vi "新想法.vi"() -> ()   [LabVIEW 2020]
uses:
  <vilib>/Utility/miscctls.llb/LVBoundsTypeDef.ctl
  <vilib>/Utility/miscctls.llb/LVRectTypeDef.ctl
  <vilib>/Instr/_visa.llb/VISA Find Search Mode.ctl
  <vilib>/Utility/miscctls.llb/LVPointTypeDef.ctl
  <vilib>/Utility/config.llb/Write Key (String).vi
  <vilib>/Utility/config.llb/Read Key (String).vi
  <vilib>/Utility/file.llb/Write Delimited Spreadsheet (string).vi
  <vilib>/Modbus/master/Modbus Master.lvclass
  <vilib>/Utility/config.llb/NI_LVConfig.lvlib
  pem/LABVIEW.dll
  <vilib>/Modbus/master/Create Master Instance (Serial).vi
panel:
  in  "数据分析":bool
  in  "实时数据":bool
  in  "按钮":bool
  in  "文本下拉列表":u16(ring)=50 items=["30"=300, "35"=350, "40"=400, "45"=450, "50"=500, "55"=550, "60"=600, "65"=650, "70"=700, "75"=750, "80"=800]
  out "当前温度 2":dbl
  out "error out":errorcluster caption="错误输出"
  out "退出":bool
  out "保存所有":bool
  out "分析":bool
  out "配置":bool
  out "连接":bool
  out "数组 2":refnum<vi>[](array[refnum])
  in  "选项卡控件 3":enum32{"选项卡 2"}(tab)
  in  "搜索设备":bool
  in  "通讯方式选择":enum32{"USB", "ETHERNET", "RS485", "GPIB"}(radio)
  in  "表格":string[][](table)
  in  "通道选择":enum32{"ALL", "A1", "A2", "A3", "A4"}(radio) caption="设置通道"
  in  "测试项目":enum32{"EIS", "极化曲线", "耐久性曲线", "线性扫描"}(radio)
  in  "1":bool
  in  "测试项目 2":enum32{"极化曲线", "耐久性测试", "EIS"}(tab)
  in  "Ⅱ区测试点数:":i32
  in  "Ⅰ区测试点数:":dbl
  in  "膜面积(cm^2):":dbl
  in  "工步 2":i32(listbox)
  out "电流密度(A/cm^2):":dbl
  in  "测试时长(H):":dbl
  in  "施加电流(A):":dbl
  in  "有效膜面积(cm^2):":dbl
  in  "VISA resource name 2":refnum<visa-resource-name>="COM3" caption="VISA resource name"
  in  "保存":bool
  in  "电解槽最大电压":dbl caption="电解槽最高温度设定："
  in  "循环水最差水质":dbl caption="冷却水最高温度："
  in  "水箱最低液位":dbl caption="冷却水最高温度："
  in  "氢气出口最大压力：":dbl caption="电解槽进口压力设定："
  in  "电解槽最高温度：":dbl caption="电解槽最高温度设定："
  in  "氢气最大露点：":dbl caption="氢气露点设定："
  in  "冷却水最高温度：":dbl
  in  "水箱补水液位：":dbl caption="水箱补水液位设定："
  in  "气液分离液位：":dbl caption="气液分离液位设定："
  in  "氢气出口背压设定：":dbl
  in  "水质换水":dbl caption="水质换水设定："
  in  "流量":T1(ring)
  in  "泵头":enum16{"YZ1515", "YZ2515", "KZ25", "YZ35"}(ring)
  in  "单选按钮":enum32{"正转", "反转"}(radio)
  in  "单选按钮 2":enum32{"四线", "二线"}(radio)
  in  "采样率":dbl
  in  "采样数":dbl
  in  "VISA resource name":refnum<visa-resource-name>="COM3"
  in  "温度25":u16(ring)=50 caption="文本下拉列表" items=["30℃"=300, "35℃"=350, "40℃"=400, "45℃"=450, "50℃"=500, "55℃"=550, "60℃"=600, "65℃"=650, "70℃"=700, "75℃"=750, "80℃"=800]
  in  "2":bool
  in  "VISA resource name 3":refnum<visa-resource-name>="COM3" caption="VISA resource name"
  in  "电源类型":u16(ring) items=["ITECH", "TDK"]
  in  "3":bool
  in  "4":bool
  out "停止测试时间:":string
  out "开始测试时间:":string
  out "报警信息":string
  out "当前电压":string
  out "当前电流":string
  in  "报警状态":bool
  in  "运行状态":bool
  out "当前温度":string
  out "通讯方式":string
  out "测试类型 2":string
  out "电压范围":string
  out "电流范围":string
  out "电源模式":string
  out "登录时间：":string
  out "用户：":string
  out "字符串 3":string
  out "队列输出 2":refnum<queue>
  in  "开始测量":bool
  in  "开始测量 3":bool caption="开始测量"
  in  "开始测量 2":bool caption="开始测量"
  in  "开始测量 4":bool caption="开始测量"
  in  "通道选择 2":enum32{"未选择", "A1", "A2", "A3", "A4"}(radio)=enum."A1"
  in  "导出曲线":bool caption="历史曲线"
  in  "保存工步":bool
  in  "添加工步":bool
  in  "历史曲线":bool
  out "刷新":bool
  in  "重排所有视图":bool
  in  "显示所有视图":bool
  in  "水质 2":bool
  in  "工步":bool
  in  "压强":bool
  in  "温度":bool
  in  "电流/电压":bool
  out "水箱液位 2":string
  out "氢中氧 2":string
  out "氢渗 2":string
  out "循环水压 2":string
  out "水质电导率 2":string
  out "电解电流 2":string
  in  "水质x轴网格线":bool
  in  "水质y轴网格线":bool
  in  "文本下拉列表 7":u16(ring) items=["线性", "散点", "分步", "分步水平"]
  in  "文本下拉列表 10":u16(ring) items=["导出数据到excel", "导出数据至剪贴板", "导出图像"]
  in  "压力x轴网格线":bool
  in  "压力y轴网格线":bool
  in  "文本下拉列表 6":u16(ring) items=["线性", "散点", "分步", "分步水平"]
  in  "文本下拉列表 9":u16(ring) items=["导出数据到excel", "导出数据至剪贴板", "导出图像"]
  in  "温度x轴网格线":bool
  in  "温度y轴网格线":bool
  in  "文本下拉列表 5":u16(ring) items=["线性", "散点", "分步", "分步水平"]
  in  "文本下拉列表 8":u16(ring) items=["导出数据到excel", "导出数据至剪贴板", "导出图像"]
  in  "文本下拉列表 2":u16(ring) items=["导出数据到excel", "导出数据至剪贴板", "导出图像"]
  in  "极化y轴网格线":bool
  in  "极化x轴网格线":bool
  in  "文本下拉列表 3":u16(ring) items=["极化曲线1", "极化曲线2"]
  in  "文本下拉列表 4":u16(ring) items=["线性", "散点", "分步", "分步水平"]
  in  "选项卡控件 2":T2(tab)
  in  "树形控件 2":string(tree)
  in  "撤销当前设置":bool
  in  "保存当前设置":bool
  in  "打开历史设置":bool
  out "水箱温度 2":string
  out "冷却水水压 2":string
  out "电解电压 2":string
  out "气分液位 2":string
  out "微量氧 2":string
  out "露点仪 2":string
  out "冷凝器液位 2":string
  out "冷凝器液位":string
  out "露点仪":string
  out "微量氧":string
  out "纯度仪":string
  out "气分液位":string
  out "电解电压":string
  out "电解电流":string
  out "水质电导率":string
  out "循环水压":string
  out "冷却水水压":string
  out "氢渗":string
  out "氢中氧":string
  out "水箱温度":string
  out "水箱液位":string
  out "纯度仪 2":string
  out "new picture":picture caption="新图片"
  in  "选项卡控件 4":enum32{"极化曲线", "温度", "压力", "水质"}(tab)
  in  "极化坐标":string
  in  "字符串 11":string
  in  "字符串 10":string
  in  "字符串 9":string
  in  "字符串 8":string
  out "XY图":cluster{"添加的数组":dbl[], "添加的数组":dbl[]}[](graph)
  in  "温度坐标":string
  out "波形图":dbl[](graph)
  in  "压力坐标":string
  out "波形图 2":dbl[](graph)
  in  "水质坐标":string
  out "波形图 3":dbl[](graph)
  out "字符串 2":string
  in  "寻找设备":bool
  in  "串口号":u16(ring)
  out "数组 8":string[](array[string])
  in  "字符串":string
  out "数值 6":i32
  out "电流":dbl
  out "电压":dbl
  out "数据":string
  in  "数组 4":refnum<vi>[](array[refnum])
  in  "数组 5":refnum<vi>[](array[refnum])
  in  "数组 6":refnum<vi>[](array[refnum])
  in  "数组 7":refnum<vi>[](array[refnum])
  out "新值":bool
  in  "字符串 4":string
  in  "字符串 5":string
  in  "字符串 6":string
  in  "字符串 7":string
  out "查找列表":string[](array[string])
  in  "数值 5":i32
  in  "数组 12":string[][](array[string]) caption="数组"
  in  "数组 11":string[][](array[string]) caption="数组"
  in  "数组 10":string[][](array[string]) caption="数组"
  in  "数组":string[][](array[string])
  in  "压力3":string[][](array[string])
  in  "压力4":string[][](array[string])
  in  "压力2":string[][](array[string])
  in  "压力1":string[][](array[string])
  out "数值":i32
  in  "test":bool
  in  "水质4":string[][](array[string])
  in  "温度4":string[][](array[string])
  in  "水质3":string[][](array[string])
  in  "温度3":string[][](array[string])
  in  "水质2":string[][](array[string])
  in  "温度2":string[][](array[string])
  in  "温度显示 4":dbl
  in  "温度显示 3":dbl
  in  "温度显示 2":dbl
  in  "温度显示":dbl
  in  "所有数据4":string[][](array[string])
  in  "所有数据3":string[][](array[string])
  in  "所有数据2":string[][](array[string])
  in  "所有数据":string[][](array[string])
  out "数值 4":i32
  out "数值 3":i32
  out "数值 2":i32
  in  "极化曲线4":dbl[][](array[numeric])
  in  "极化电压4":dbl
  in  "极化电流4":dbl
  in  "电压4":dbl[](array[numeric])
  in  "电流4":dbl[](array[numeric])
  in  "极化曲线3":dbl[][](array[numeric])
  in  "极化电压3":dbl
  in  "极化电流3":dbl
  in  "电压3":dbl[](array[numeric])
  in  "电流3":dbl[](array[numeric])
  in  "极化曲线2":dbl[][](array[numeric])
  in  "极化电压2":dbl
  in  "极化电流2":dbl
  in  "电压2":dbl[](array[numeric])
  in  "电流2":dbl[](array[numeric])
  in  "极化曲线1":dbl[][](array[numeric])
  in  "极化电压1":dbl
  in  "极化电流1":dbl
  in  "电压1":dbl[](array[numeric])
  in  "电流1":dbl[](array[numeric])
  in  "水质1":string[][](array[string])
  in  "温度1":string[][](array[string])
  in  "数组 3":refnum<vi>[](array[refnum])
  out "输出电磁阀":bool
  out "露点电磁阀":bool
  out "流量电磁阀":bool
  out "补水电磁阀":bool
  out "排水电磁阀":bool
  out "冷水控温阀":bool
  out "排尽电磁阀":bool
  out "冷却水温度过高报警":bool
  out "电堆超压报警":bool
  out "露点报警":bool
  out "电堆温度报警":bool
  out "积水报警":bool
  out "水质报警":bool
  out "水箱缺水报警":bool
  out "循环水温度报警":bool
  out "循环水流量报警":bool
  out "氢气出口超压报警":bool
  # "设备列表"
  # "参数设置"
  # "测试设置"
  # "VISA"
  # "VISA"
  # "MPa"
  # "MΩ.cm"
  # "cm"
  # "cm"
  # "报警参数设置"
  # "℃"
  # "℃"
  # "V"
  # "℃"
  # "cm"
  # "MPa"
  # "MΩ.cm"
  # "工作设置"
  # "电源设置"
  # "VISA"
  # "通道设置"
  # "工步设置"
  # "测试通道"
  # "CH1"
  # "CH2"
  # "CH3"
  # "CH4"
  # "电磁阀状态"
  # "报警状态"
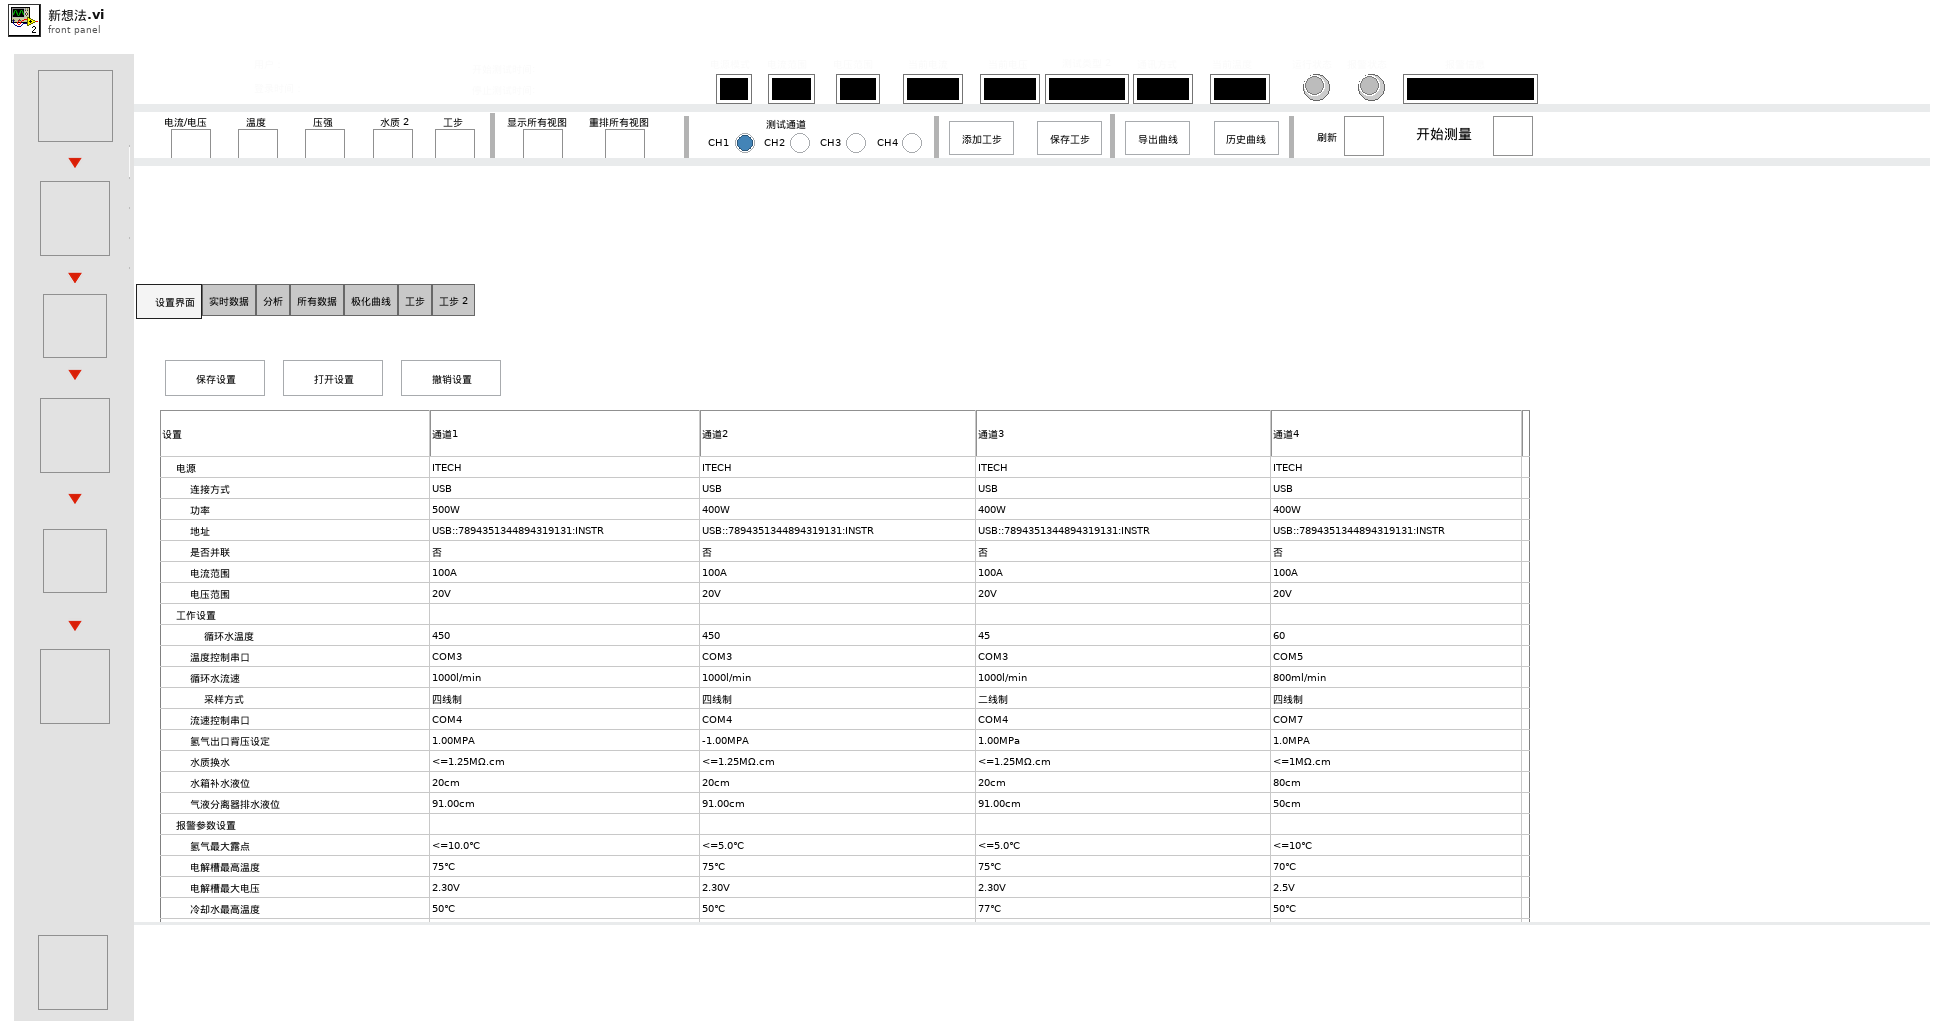
[diagram p1: front panel]
types:
  T1 = enum16{"200ml/min", "400lml/min", "600ml/min", "800ml/min", "1000ml/min", "1200ml/min", "1400ml/min", "1600ml/min"}
  T2 = enum32{"    设置界面", "实时数据", "分析", "所有数据", "极化曲线", "工步", "工步 2"}
  T3 = enum16{"Always On", "Always Off", "Off While Running"}
  T4 = enum8{"Enabled", "Disabled", "Disabled and Grayed Out"}
  T5 = typedef "LVBoundsTypeDef.ctl" = cluster{"Width":u32, "Height":u32}
  T6 = typedef "imagedata.ctl" = cluster{"image type":i32, "image depth":i32, "image":u8[], "mask":u8[], "colors":u32[], "Rectangle":cluster{"left":i16, "top":i16, "right":i16, "bottom":i16}}
  T7 = typedef "LVPointTypeDef.ctl" = cluster{"Horizontal":i16, "Vertical":i16}
  T8 = cluster{"温度1":refnum<vi>, "温度2":refnum<vi>, "温度3":refnum<vi>, "温度4":refnum<vi>}
  T9 = cluster{"水质1":refnum<vi>, "水质2":refnum<vi>, "水质3":refnum<vi>, "水质4":refnum<vi>}
  T10 = cluster{"极化曲线1":refnum<vi>, "极化曲线2":refnum<vi>, "极化曲线3":refnum<vi>, "极化曲线4":refnum<vi>}
  T11 = cluster{"电压1":refnum<vi>, "电压2":refnum<vi>, "电压3":refnum<vi>, "电压4":refnum<vi>}
  T12 = cluster{"电流1":refnum<vi>, "电流2":refnum<vi>, "电流3":refnum<vi>, "电流4":refnum<vi>}
  T13 = cluster{"压力1":refnum<vi>, "压力2":refnum<vi>, "压力3":refnum<vi>, "压力4":refnum<vi>}
  T14 = cluster{"所有数据":refnum<vi>, "所有数据2":refnum<vi>, "所有数据3":refnum<vi>, "所有数据4":refnum<vi>}
  T15 = enum32{"Invalid", "Standard", "Closed", "Hidden", "Minimized", "Maximized"}
  T16 = cluster{"所有数据":refnum<vi>, "数值":refnum<vi>, "极化曲线1":refnum<vi>, "极化电压1":refnum<vi>, "极化电流1":refnum<vi>, "电压1":refnum<vi>, "电流1":refnum<vi>, "水质1":refnum<vi>, "温度1":refnum<vi>, "温度显示":refnum<vi>, "压力1":refnum<vi>}
  T17 = cluster{"水质2":refnum<vi>, "温度2":refnum<vi>, "温度显示 2":refnum<vi>, "所有数据2":refnum<vi>, "数值 2":refnum<vi>, "极化曲线2":refnum<vi>, "极化电压2":refnum<vi>, "极化电流2":refnum<vi>, "电压2":refnum<vi>, "电流2":refnum<vi>, "压力2":refnum<vi>}
  T18 = cluster{"水质3":refnum<vi>, "温度3":refnum<vi>, "温度显示 3":refnum<vi>, "所有数据3":refnum<vi>, "数值 3":refnum<vi>, "极化曲线3":refnum<vi>, "极化电压3":refnum<vi>, "极化电流3":refnum<vi>, "电压3":refnum<vi>, "电流3":refnum<vi>, "压力3":refnum<vi>}
  T19 = cluster{"水质4":refnum<vi>, "温度4":refnum<vi>, "温度显示 4":refnum<vi>, "所有数据4":refnum<vi>, "数值 4":refnum<vi>, "极化曲线4":refnum<vi>, "极化电压4":refnum<vi>, "极化电流4":refnum<vi>, "电压4":refnum<vi>, "电流4":refnum<vi>, "压力4":refnum<vi>}
  T20 = typedef "LVRectTypeDef.ctl" = cluster{"Left":i16, "Top":i16, "Right":i16, "Bottom":i16}
  T21 = enum16{"open", "replace", "create", "open or create", "replace or create", "replace or create with confirmation"}
  T22 = typedef "LVPoint32TypeDef.ctl" = cluster{"Horizontal":i32, "Vertical":i32}
  T23 = enum32{"Bad", "Idle", "Run top level", "Running"}
  T24 = cluster{"添加的数组":dbl[], "添加的数组":dbl[], "添加的数组":dbl[], "添加的数组":dbl[], dbl}
  T25 = typedef "NI_LVConfig.lvlib/Config Data RefNum.ctl" = refnum<k1>
  T26 = cluster{string, string[], string, i32, bool, i32}
  T27 = typedef "VISA Find Search Mode.ctl" = u32
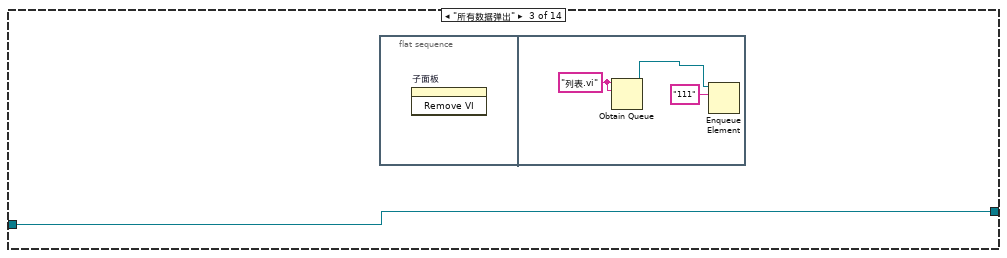
[diagram p4: hidden frame]
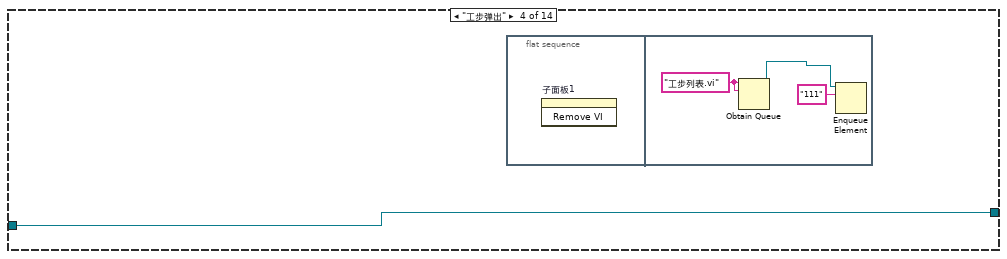
[diagram p5: hidden frame]
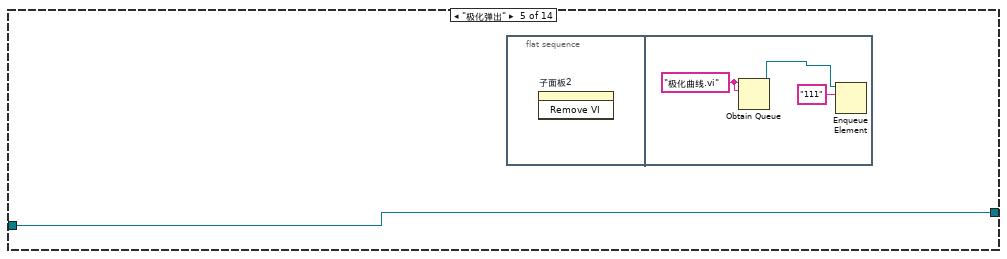
[diagram p6: hidden frame]
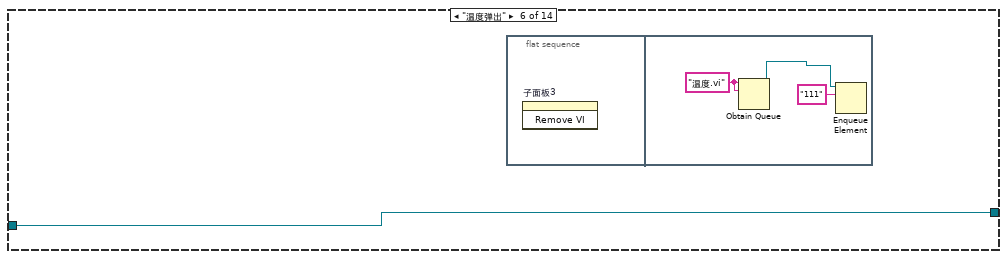
[diagram p7: hidden frame]
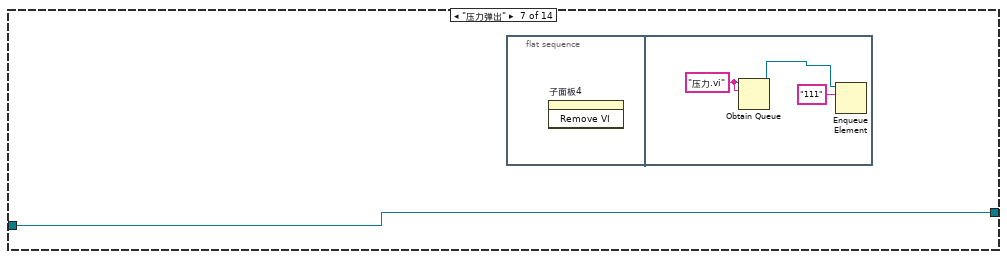
[diagram p8: hidden frame]
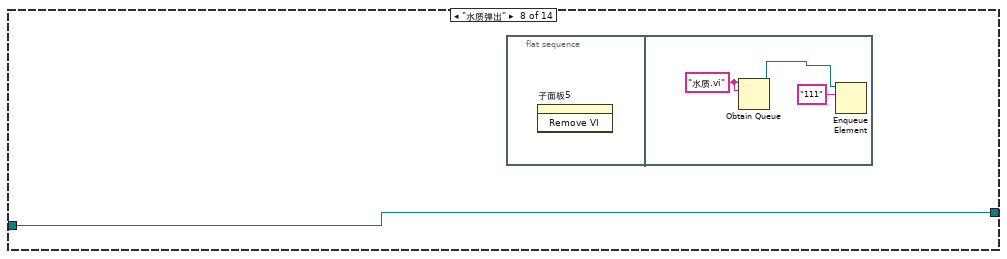
[diagram p9: hidden frame]
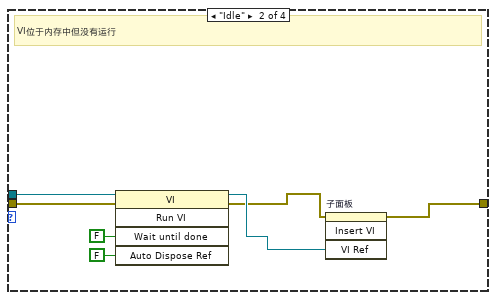
[diagram p12: hidden frame]
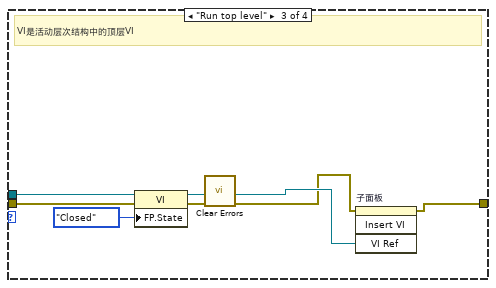
[diagram p13: hidden frame]
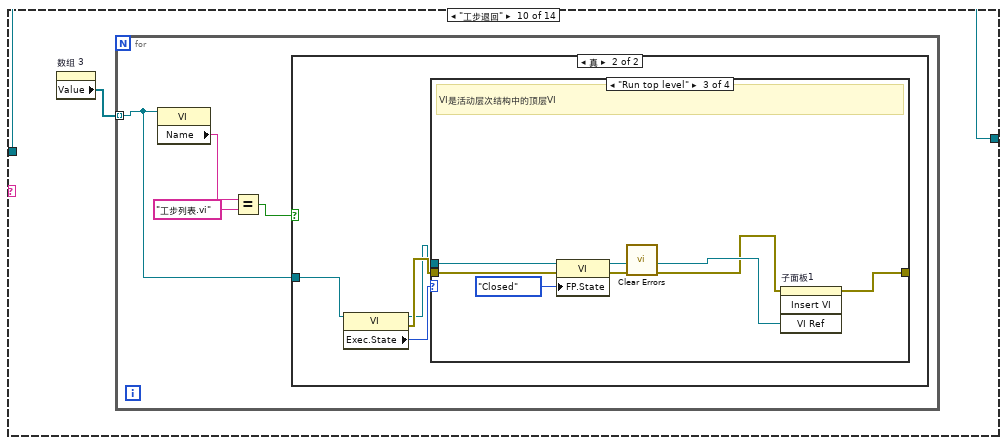
[diagram p14: hidden frame]
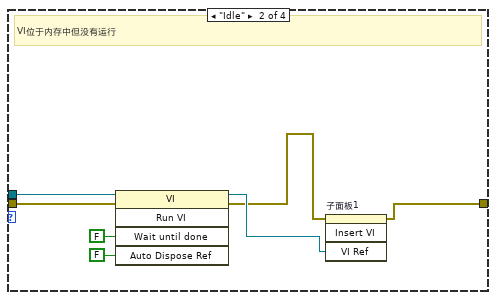
[diagram p17: hidden frame]
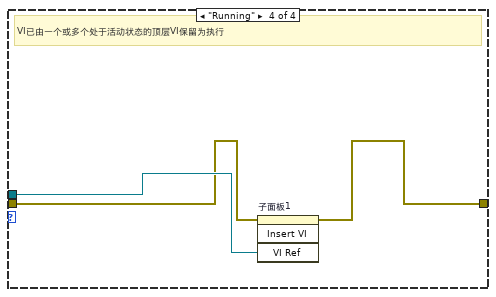
[diagram p18: hidden frame]
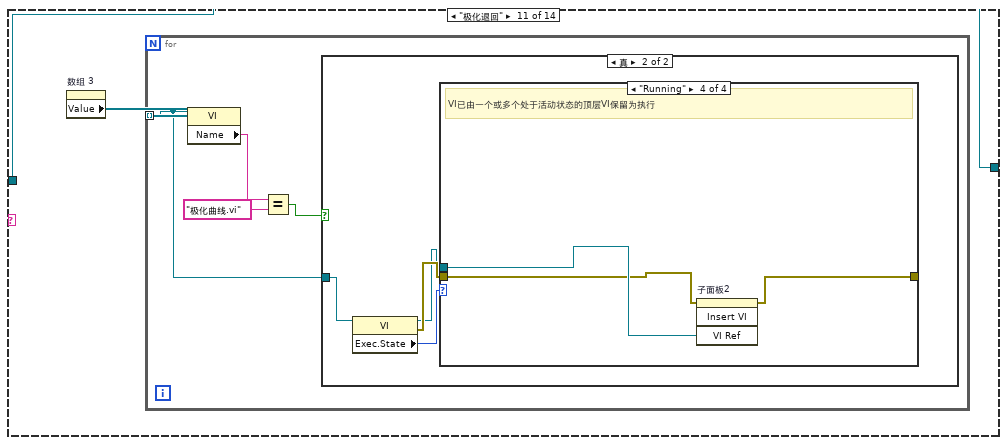
[diagram p19: hidden frame]
diagram:
  (unwired) string[] ["循环水温度", "温度控制串口", "循环水流速", "流速控制串口", "采样方式", "氢气出口背压设定", "水质换水", "水箱补水液位", "气液分离器排水液位", "氢气最大露点", "电解槽最高温度", "电解槽最大电压", "冷却水最高温度", "水箱最低液位", "氢气出口最大压力", "循环水最差水质"]
  (unwired) TRUE ("布尔 17")
  (unwired) "添加工步"
  # "A2"
  # "USB0::0x2EC7::0x3000::803489033757710010::INSTR"
  # "a1"
  # "USB0::0x2EC7::0x3000::803489033757710011::INSTR"
  n1 = flat-sequence {
    frame #0 {
      n2 = control-ref of="冷凝器液位 2"() -> (w98:refnum<vi>)
      n3 = control-ref of="露点仪 2"() -> (w99:refnum<vi>)
      n4 = control-ref of="微量氧 2"() -> (w100:refnum<vi>)
      n5 = control-ref of="纯度仪 2"() -> (w101:refnum<vi>)
      n6 = control-ref of="气分液位 2"() -> (w102:refnum<vi>)
      n7 = control-ref of="电解电压 2"() -> (w103:refnum<vi>)
      n8 = control-ref of="电解电流 2"() -> (w104:refnum<vi>)
      n9 = control-ref of="水质电导率 2"() -> (w105:refnum<vi>)
      n10 = control-ref of="循环水压 2"() -> (w106:refnum<vi>)
      n11 = control-ref of="冷却水水压 2"() -> (w107:refnum<vi>)
      n12 = control-ref of="氢渗 2"() -> (w108:refnum<vi>)
      n13 = control-ref of="氢中氧 2"() -> (w109:refnum<vi>)
      n14 = control-ref of="水箱温度 2"() -> (w110:refnum<vi>)
      n15 = control-ref of="水箱液位 2"() -> (w111:refnum<vi>)
      n16 = Build Array(w98, w99, w100, w101, w102, w103, w104, w105, w106, w107, w108, w109, w110, w111) -> (w112:refnum<vi>[])
      n17 = control-ref of="冷凝器液位"() -> (w83:refnum<vi>)
      n18 = control-ref of="露点仪"() -> (w84:refnum<vi>)
      n19 = control-ref of="微量氧"() -> (w85:refnum<vi>)
      n20 = control-ref of="纯度仪"() -> (w86:refnum<vi>)
      n21 = control-ref of="气分液位"() -> (w87:refnum<vi>)
      n22 = control-ref of="电解电压"() -> (w88:refnum<vi>)
      n23 = control-ref of="电解电流"() -> (w89:refnum<vi>)
      n24 = control-ref of="水质电导率"() -> (w90:refnum<vi>)
      n25 = control-ref of="循环水压"() -> (w91:refnum<vi>)
      n26 = control-ref of="冷却水水压"() -> (w92:refnum<vi>)
      n27 = control-ref of="氢渗"() -> (w93:refnum<vi>)
      n28 = control-ref of="氢中氧"() -> (w94:refnum<vi>)
      n29 = control-ref of="水箱温度"() -> (w95:refnum<vi>)
      n30 = control-ref of="水箱液位"() -> (w96:refnum<vi>)
      n31 = Build Array(w83, w84, w85, w86, w87, w88, w89, w90, w91, w92, w93, w94, w95, w96) -> (w97:refnum<vi>[])
      n32 = for {
        tunnel: w97 -> [w116] mode=indexing
        tunnel: w112 -> [w114] mode=indexing
        n33 = property class="Str"(reference=w114, "Visible"=FALSE ("可见")) -> ()  [unwired: 1 in, 2 out]
        n34 = property class="Str"(reference=w116, "Visible"=FALSE ("可见")) -> ()  [unwired: 1 in, 2 out]
      }
    }
    frame #1 {
      n35 = for {
        tunnel: i32[] [5] -> [w120] mode=indexing
        n36 = property on="窗格" class="Pane"() -> ("Decos[]"=w119:refnum<vi>[])  [unwired: 2 in, 2 out]
        n37 = Index Array(array=w119, index=w120) -> (element=w118:refnum<vi>)
        n38 = property class="Decor"(reference=w118, "Visible"=TRUE ("可见")) -> ()  [unwired: 1 in, 2 out]
      }
    }
    frame #2 {
      n39 = disable-structure shown="禁用" {
        frame Disabled {
          n40 = for {
            tunnel: i32[] [0, 1, 2, 3, 4] -> [w126] mode=indexing
            n41 = property on="窗格" class="Pane"() -> ("Decos[]"=w125:refnum<vi>[])  [unwired: 2 in, 2 out]
            n42 = Index Array(array=w125, index=w126) -> (element=w124:refnum<vi>)
            n43 = property class="Decor"(reference=w124, "Visible"=FALSE ("可见")) -> ()  [unwired: 1 in, 2 out]
          }
        }
        frame Enabled {
        }
      }
      n44 = property on="分隔栏 2" class="Splitter"("Position"=113 ("分隔栏位置")) -> ()  [unwired: 2 in, 2 out]
    }
    frame #3 {
      n45 = property on="分隔栏 3" class="Splitter"("Position"=116 ("分隔栏位置")) -> ()  [unwired: 2 in, 2 out]
    }
    frame #4 {
      n46 = stacked-sequence {
        frame #0 {
          n47 = property on="分隔栏 4" class="Splitter"() -> ("Position"=w129:i32)  [unwired: 2 in, 2 out]
          n48 = Add(x=w129, y=32 ("分隔栏位置")) -> (x+y=w131:i32)
          n49 = property on="分隔栏 5" class="Splitter"("Position"=w131) -> ()  [unwired: 2 in, 2 out]
        }
        frame #1 {
          n50 = property on="分隔栏 4" class="Splitter"() -> ("Position"=w134:i32)  [unwired: 2 in, 2 out]
          n51 = Add(x=w134, y=62 ("分隔栏位置")) -> (x+y=w133:i32)
          n52 = property on="分隔栏 6" class="Splitter"("Position"=w133) -> ()  [unwired: 2 in, 2 out]
        }
        frame #2 {
          n53 = property on="分隔栏 4" class="Splitter"() -> ("Position"=w137:i32)  [unwired: 2 in, 2 out]
          n54 = Add(x=w137, y=92 ("分隔栏位置")) -> (x+y=w136:i32)
          n55 = property on="分隔栏 7" class="Splitter"("Position"=w136) -> ()  [unwired: 2 in, 2 out]
        }
        frame #3 {
          n56 = property on="分隔栏 4" class="Splitter"() -> ("Position"=w140:i32)  [unwired: 2 in, 2 out]
          n57 = Add(x=w140, y=122 ("分隔栏位置")) -> (x+y=w138:i32)
          n58 = property on="分隔栏 8" class="Splitter"("Position"=w138) -> ()  [unwired: 2 in, 2 out]
        }
      }
    }
  }
  n59 = disable-structure shown="禁用" {
    frame Disabled {
      n60 = flat-sequence {
        frame #0 {
          w141 = "已完成" ("活动单元格:字符串")
          w142 = 8 ("活动单元格:活动列数")
          w145 = "A1" ("活动项:标识符")
          n61 = Add() -> (x=w144:dbl, x+y=w143:dbl)  [unwired: 1 in]
        }
        frame #1 {
          n62 = Index Array(array=w151, index (col)=0 ("禁用的索引 (列)")) -> (element=w149)  [unwired: 1 in]
          n63 = Search 1D Array(1D array=w149, element=" " ("元素")) -> (index of element=w147:i32)  [unwired: 1 in]
          n64 = Equal?(y=w147) -> (x = y?=w146:bool)  [unwired: 1 in]
          n65 = case shown="假" w146 {
            tunnel: [w157 _] -> w151
            frame False {
              w152 = u32 6618880
              w153 = "正在运行" ("活动单元格:字符串")
              w154 = 8 ("活动单元格:活动列数")
              w155 = "A1" ("活动项:标识符")
              w161 = 3 ("活动单元格:活动列数")
              w162 = "A1" ("活动项:标识符")
              w167 = 5 ("活动单元格:活动列数")
              w168 = "A1" ("活动项:标识符")
              w172 = 4 ("活动单元格:活动列数")
              w171 = "A1" ("活动项:标识符")
              w175 = 7 ("活动单元格:活动列数")
              w174 = "A1" ("活动项:标识符")
              n66 = Index Array(array=w157) -> (element=w164)  [unwired: 2 in]
              n67 = Increment() -> (x+1=w156:dbl)  [unwired: 1 in]
              n68 = Index Array(array=w164, index=3 ("索引")) -> (element=w165)
              n69 = Index Array(array=w164, index=2 ("索引")) -> (element=w169)
              n70 = Index Array(array=w164, index=5 ("索引")) -> (element=w173)
              n71 = Format Into String(w156) -> (resulting string=w159:string)  [unwired: 3 in, 1 out]
              n72 = Concatenate Strings("工步", w159) -> (w158:string)
            }
            frame True {
              w176 = "已完成" ("活动单元格:字符串")
              w177 = 8 ("活动单元格:活动列数")
              w178 = "A1" ("活动项:标识符")
            }
          }
        }
        frame #2 {
          n73 = case shown="真" {
            selector: _ -> [_ _]
            tunnel: [w180 w201] -> w179
            frame False {
              n74 = Index Array(array=w188) -> (element=w189, index=w190:i32)
              n75 = Unbundle(w189) -> (w183, w185)
              n76 = Build Array(w183) -> (w184:void[], w182)
              n77 = Build Array (concatenate)(w185) -> (w186:void[], w181:void[])
              n78 = Bundle(w184, w186) -> (w187:cluster{void[], void[]})  [unwired: 1 in]
              n79 = Replace Array Subset(new element=w187, index=w190) -> (array=w188:cluster{void[], void[]}[], w180:cluster{void[], void[]}[])
            }
            frame True {
              n80 = Array Size() -> (array=w196:dbl[], size(s)=w197:i32)
              n81 = Index Array(array=w196, index=w197) -> (element=w198)
              n82 = Unbundle(w198) -> (w195, w194)
              n83 = Build Array (concatenate)(w195) -> (w193:void[], w200:void[])
              n84 = Build Array (concatenate)(w194) -> (w192:void[], w199:void[])
              n85 = Bundle(w193, w192) -> (w191:cluster{void[], void[]})  [unwired: 1 in]
              n86 = Insert Into Array(array=w196, new element=w191) -> (w201:cluster{void[], void[]}[])  [unwired: 1 in]
            }
          }
        }
      }
    }
    frame Enabled {
    }
  }
  n87 = disable-structure shown="禁用" {
    frame Disabled {
      n88 = case shown="\"YZ35\"" {
        selector: _ -> [_ _ _ _]
        tunnel: ["YZ1515" "yz2515" "KZ25" "YZ35"] -> _
        frame "YZ1515", Default {
        }
        frame "YZ2515" {
        }
        frame "KZ25" {
        }
        frame "YZ35" {
        }
      }
    }
    frame Enabled {
    }
  }
  n89 = property on="电压" class="DigNum (严格)"() -> ("Value"=w45:dbl)  [unwired: 2 in, 2 out]
  n90 = property on="电流" class="DigNum (严格)"() -> ("Value"=w42:dbl)  [unwired: 2 in, 2 out]
  n91 = flat-sequence {
    tunnel: [w222] -> w2
    frame #0 {
      w243 = u16 1 items=["ITECK", "TDK"] ("电源类型")
      w259 = T4."Enabled" ("禁用")
      w247 = string[][] []
      n92 = property on="重排所有视图" class="Bool (严格)"("Value"=FALSE ("重排所有视图")) -> (error out=w209:errorcluster)  [unwired: 2 in, 1 out]
      n93 = property on="显示所有视图" class="Bool (严格)"(error in=w209, "Value"=FALSE ("显示所有视图")) -> (error out=w208:errorcluster)  [unwired: 1 in, 1 out]
      n94 = property on="压强" class="Bool (严格)"(error in=w208, "Value"=FALSE ("压强")) -> (error out=w216:errorcluster)  [unwired: 1 in, 1 out]
      n95 = property on="电流/电压" class="Bool (严格)"(error in=w216, "Value"=FALSE ("电流/电压")) -> (error out=w215:errorcluster)  [unwired: 1 in, 1 out]
      n96 = property on="温度" class="Bool (严格)"(error in=w215, "Value"=FALSE ("温度")) -> (error out=w214:errorcluster)  [unwired: 1 in, 1 out]
      n97 = property on="工步" class="Bool (严格)"(error in=w214, "Value"=FALSE ("工步")) -> (error out=w213:errorcluster)  [unwired: 1 in, 1 out]
      n98 = property on="水质 2" class="Bool (严格)"(error in=w213, "Value"=FALSE ("水质 2")) -> (error out=w212:errorcluster)  [unwired: 1 in, 1 out]
      n99 = property on="选项卡控件 4" class="TabCtl (严格)"(error in=w212, "Value"=enum32{"极化曲线", "温度", "压力", "水质"}."极化曲线" ("选项卡控件 4")) -> (error out=w231:errorcluster)  [unwired: 1 in, 1 out]
      n100 = property on="电源类型" class="Ring (严格)"(error in=w231, "Value"=w243) -> (error out=w242:errorcluster)  [unwired: 1 in, 1 out]
      n101 = property on="选项卡控件 2" class="TabCtl (严格)"(error in=w242, "Value"=T2."    设置界面" ("选项卡控件 2")) -> (error out=w207:errorcluster)  [unwired: 1 in, 1 out]
      n102 = property on="通道选择 2" class="RadioBtnsControl (严格)"(error in=w207, "Value"=enum32{"未选择", "A1", "A2", "A3", "A4"}."A1" ("通道选择 2")) -> (error out=w265:errorcluster)  [unwired: 1 in, 1 out]
      n103 = property on="通道选择" class="RadioBtnsControl (严格)"(error in=w265, "Value"=enum32{"ALL", "A1", "A2", "A3", "A4"}."ALL" ("通道选择")) -> (error out=w263:errorcluster)  [unwired: 1 in, 1 out]
      n104 = property on="测试项目" class="RadioBtnsControl (严格)"(error in=w263, "Value"=enum32{"EIS", "极化曲线", "耐久性曲线", "线性扫描"}."极化曲线" ("测试项目：")) -> (error out=w261:errorcluster)  [unwired: 1 in, 1 out]
      n105 = property on="测试项目 2" class="TabCtl (严格)"(error in=w261, "Value"=enum32{"极化曲线", "耐久性测试", "EIS"}."极化曲线" ("测试项目 2")) -> (error out=w260:errorcluster)  [unwired: 1 in, 1 out]
      n106 = property on="数组 3" class="Arr (严格)"(error in=w260, "Value"=refnum<vi>[] [] ("数组 3")) -> (error out=w289:errorcluster)  [unwired: 1 in, 1 out]
      n107 = property on="数组" class="Arr (严格)"(error in=w289, "Value"=w247) -> (error out=w248:errorcluster)  [unwired: 1 in, 1 out]
      n108 = property on="数组 10" class="Arr (严格)"(error in=w248, "Value"=w247) -> (error out=w245:errorcluster)  [unwired: 1 in, 1 out]
      n109 = property on="数组 11" class="Arr (严格)"(error in=w245, "Value"=w247) -> (error out=w246:errorcluster)  [unwired: 1 in, 1 out]
      n110 = property on="数组 12" class="Arr (严格)"(error in=w246, "Value"=w247) -> (error out=w244:errorcluster)  [unwired: 1 in, 1 out]
      n111 = property on="数组 2" class="Arr (严格)"(error in=w244, "Value"=refnum<vi>[] [] ("数组 2")) -> (error out=w272:errorcluster)  [unwired: 1 in, 1 out]
      n112 = property on="数组 4" class="Arr (严格)"(error in=w272, "Value"=refnum<vi>[] [] ("数组 4")) -> (error out=w258:errorcluster)  [unwired: 1 in, 1 out]
      n113 = property on="分析" class="Bool (严格)"(error in=w258, "DisabledEnum"=w259) -> (error out=w257:errorcluster)  [unwired: 1 in, 1 out]
      n114 = property on="保存所有" class="Bool (严格)"(error in=w257, "DisabledEnum"=w259) -> (error out=w256:errorcluster)  [unwired: 1 in, 1 out]
      n115 = property on="连接" class="Bool (严格)"(error in=w256, "DisabledEnum"=w259) -> (error out=w255:errorcluster)  [unwired: 1 in, 1 out]
      n116 = property on="配置" class="Bool (严格)"(error in=w255, "DisabledEnum"=w259) -> (error out=w254:errorcluster)  [unwired: 1 in, 1 out]
      n117 = property on="通道选择" class="RadioBtnsControl (严格)"(error in=w254, "DisabledEnum"=w259) -> (error out=w253:errorcluster)  [unwired: 1 in, 1 out]
      n118 = property on="2" class="Bool (严格)"(error in=w253, "DisabledEnum"=w259) -> (error out=w252:errorcluster)  [unwired: 1 in, 1 out]
      n119 = property on="3" class="Bool (严格)"(error in=w252, "DisabledEnum"=w259) -> (error out=w251:errorcluster)  [unwired: 1 in, 1 out]
      n120 = property on="4" class="Bool (严格)"(error in=w251, "DisabledEnum"=w259) -> (error out=w250:errorcluster)  [unwired: 1 in, 1 out]
      n121 = property on="数组 5" class="Arr (严格)"(error in=w250, "Value"=refnum<vi>[] [] ("数组 4")) -> (error out=w270:errorcluster)  [unwired: 1 in, 1 out]
      n122 = property on="数组 6" class="Arr (严格)"(error in=w270, "Value"=refnum<vi>[] [] ("数组 4")) -> (error out=w269:errorcluster)  [unwired: 1 in, 1 out]
      n123 = property on="数组 7" class="Arr (严格)"(error in=w269, "Value"=refnum<vi>[] [] ("数组 4")) -> (error out=w241:errorcluster)  [unwired: 1 in, 1 out]
      n124 = property on="开始测量" class="Bool (严格)"(error in=w241, "Visible"=TRUE ("可见")) -> (error out=w284:errorcluster)  [unwired: 1 in, 1 out]
      n125 = property on="开始测量 2" class="Bool (严格)"(error in=w284, "Visible"=FALSE ("可见")) -> (error out=w283:errorcluster)  [unwired: 1 in, 1 out]
      n126 = property on="开始测量 3" class="Bool (严格)"(error in=w283, "Visible"=FALSE ("可见")) -> (error out=w282:errorcluster)  [unwired: 1 in, 1 out]
      n127 = property on="开始测量 4" class="Bool (严格)"(error in=w282, "Visible"=FALSE ("可见")) -> (error out=w281:errorcluster)  [unwired: 1 in, 1 out]
      n128 = property on="开始测量" class="Bool (严格)"(error in=w281, "Value"=FALSE ("开始测量")) -> (error out=w279:errorcluster)  [unwired: 1 in, 1 out]
      n129 = property on="开始测量 2" class="Bool (严格)"(error in=w279, "Value"=FALSE ("开始测量 2")) -> (error out=w277:errorcluster)  [unwired: 1 in, 1 out]
      n130 = property on="开始测量 3" class="Bool (严格)"(error in=w277, "Value"=FALSE ("开始测量 3")) -> (error out=w275:errorcluster)  [unwired: 1 in, 1 out]
      n131 = property on="开始测量 4" class="Bool (严格)"(error in=w275, "Value"=FALSE ("开始测量 4")) -> (error out=w240:errorcluster)  [unwired: 1 in, 1 out]
      n132 = property on="表格" class="Tbl (严格)"(error in=w240, "Value"=string[][] [] ("表格")) -> (error out=w237:errorcluster)  [unwired: 1 in, 1 out]
      n133 = property on="字符串 4" class="Str"(error in=w237, "Value"="" ("字符串 4")) -> (error out=w235:errorcluster)  [unwired: 1 in, 1 out]
      n134 = property on="新值" class="Bool (严格)"(error in=w235, "Value"=FALSE ("新值")) -> (error out=w233:errorcluster)  [unwired: 1 in, 1 out]
      n135 = property on="导出曲线" class="Bool (严格)"(error in=w233, "Value"=FALSE ("导出曲线")) -> (error out=w230:errorcluster)  [unwired: 1 in, 1 out]
      n136 = property on="极化坐标" class="Str"(error in=w230, "Visible"=FALSE ("可见")) -> (error out=w225:errorcluster)  [unwired: 1 in, 1 out]
      n137 = property on="水质坐标" class="Str"(error in=w225, "Visible"=FALSE ("可见")) -> (error out=w224:errorcluster)  [unwired: 1 in, 1 out]
      n138 = property on="压力坐标" class="Str"(error in=w224, "Visible"=FALSE ("可见")) -> (error out=w223:errorcluster)  [unwired: 1 in, 1 out]
      n139 = property on="温度坐标" class="Str"(error in=w223, "Visible"=FALSE ("可见")) -> (error out=w222:errorcluster)  [unwired: 1 in, 1 out]
    }
  }
  n140 = Bundle By Name(cluster=cluster{"状态":bool, "错误码":i32, string} {"状态"=TRUE, "错误码"=0, ""} ("输入簇"), "状态"=TRUE, "错误码"=0) -> (w78:cluster{"状态":bool, "错误码":i32, string})
  n141 = Number To Fractional String(number=w42, precision (6)=i16 1 ("精度(6)")) -> (F-format string=→"当前电压":string)  [unwired: 2 in]
  n142 = Number To Fractional String(number=w45, precision (6)=i16 1 ("精度(6)")) -> (F-format string=→"当前电流":string)  [unwired: 2 in]
  n143 = control-ref of="窗格 9"() -> (w58:refnum<vi>)
  n144 = Obtain Queue(name (unnamed)="数据处理队列" ("名称（未命名）"), element data type=w78, create if not found? (T)=TRUE ("如未找到则创建？(T)")) -> (queue out=w76:refnum<queue>)  [unwired: 2 in, 2 out]
  "队列输出 2" <- w76
  n145 = property class="Pane"(reference=w58, "VertScrollbarVisibility"=T3."Always Off" ("垂直滚动条可见")) -> (error out=w56:errorcluster)  [unwired: 1 in, 1 out]
  n146 = control-ref of="水质1"() -> ()  [unwired: 1 out]
  n147 = control-ref of="水质2"() -> ()  [unwired: 1 out]
  n148 = control-ref of="水质3"() -> ()  [unwired: 1 out]
  n149 = control-ref of="水质4"() -> ()  [unwired: 1 out]
  n150 = property on="4" class="Bool (严格)"(error in=w56, "Value"=FALSE ("3 2")) -> (error out=w59:errorcluster)  [unwired: 1 in, 1 out]
  n151 = while {
    tunnel: w76 -> [w293]
    tunnel: [w292] -> w75
    stop <- FALSE stop-if-true
    n152 = event shown="[0] 超时" {
      selector: _ -> [_]
      dyn-events: _ -> [_]
      timeout: 100 -> [_]
      tunnel: w293 -> [w302]
      tunnel: [w299] -> w292
      event Timeout {
        n153 = event-data() -> ()  [unwired: 1 in, 3 out]
        n154 = Dequeue Element(queue=w302, timeout in ms (-1)=-1 ("超时毫秒(-1)")) -> (queue out=w299:refnum<queue>, element=w300:cluster{"状态":bool, "错误码":i32, string})  [unwired: 1 in, 2 out]
        n155 = Unbundle(w300) -> ("状态"=w296:bool, "错误码"=w297:i32, w298:string)
        n156 = case shown="真" w296 {
          tunnel: w298 -> [_ w308]
          tunnel: w297 -> [_ w306]
          frame False {
          }
          frame True {
            n157 = Format Into String(w306) -> (resulting string=w305:string)  [unwired: 3 in, 1 out]
            n158 = Concatenate Strings(w308, "错误：" ("字符串"), w305) -> (w304:string)
            n159 = One Button Dialog(message=w304, button name ("OK")="确定" ("按钮名称（“确定”）")) -> ()  [unwired: 1 out]
          }
        }
      }
    }
  }
  n160 = property on="1" class="Bool (严格)"(error in=w59, "Value"=FALSE ("1")) -> (error out=w71:errorcluster)  [unwired: 1 in, 1 out]
  n161 = property on="2" class="Bool (严格)"(error in=w71, "Value"=FALSE ("2")) -> (error out=w70:errorcluster)  [unwired: 1 in, 1 out]
  n162 = property on="3" class="Bool (严格)"(error in=w70, "Value"=FALSE ("3")) -> (error out=w67:errorcluster)  [unwired: 1 in, 1 out]
  n163 = control-ref of="窗格 6"() -> (w69:refnum<vi>)
  n164 = property class="Pane"(reference=w69, error in=w67, "VertScrollbarVisibility"=T3."Always Off" ("垂直滚动条可见")) -> (error out=w64:errorcluster)  [unwired: 1 out]
  n165 = Release Queue(queue=w75) -> ()  [unwired: 2 in, 3 out]
  n166 = control-ref of="窗格 7"() -> (w65:refnum<vi>)
  n167 = property class="Pane"(reference=w65, error in=w64, "VertScrollbarVisibility"=T3."Always Off" ("垂直滚动条可见")) -> (error out=w61:errorcluster)  [unwired: 1 out]
  n168 = control-ref of="窗格 8"() -> (w62:refnum<vi>)
  n169 = property class="Pane"(reference=w62, error in=w61, "VertScrollbarVisibility"=T3."Always Off" ("垂直滚动条可见")) -> (error out=w39:errorcluster)  [unwired: 1 out]
  n170 = flat-sequence {
    tunnel: [w347] -> w1
    tunnel: w2 -> [w309]
    frame #0 {
      w339 = 0 ("数值 2")
      w355 = string[][] [] ("温度1")
      w356 = dbl[] [] ("电压1")
      w345 = string[][] [] ("温度1")
      n171 = property on="数值 4" class="DigNum (严格)"(error in=w309, "Value"=0 ("数值 4")) -> (error out=w323:errorcluster)  [unwired: 1 in, 1 out]
      n172 = property on="电压4" class="Arr (严格)"(error in=w323, "Value"=dbl[] [] ("电压4")) -> (error out=w322:errorcluster)  [unwired: 1 in, 1 out]
      n173 = property on="电流4" class="Arr (严格)"(error in=w322, "Value"=dbl[] [] ("电流4")) -> (error out=w321:errorcluster)  [unwired: 1 in, 1 out]
      n174 = property on="极化曲线4" class="Arr (严格)"(error in=w321, "Value"=dbl[][] [] ("极化曲线4")) -> (error out=w320:errorcluster)  [unwired: 1 in, 1 out]
      n175 = property on="所有数据4" class="Arr (严格)"(error in=w320, "Value"=string[][] [] ("所有数据4")) -> (error out=w319:errorcluster)  [unwired: 1 in, 1 out]
      n176 = property on="水质4" class="Arr (严格)"(error in=w319, "Value"=string[][] [] ("水质4")) -> (error out=w318:errorcluster)  [unwired: 1 in, 1 out]
      n177 = property on="温度4" class="Arr (严格)"(error in=w318, "Value"=string[][] [] ("温度4")) -> (error out=w317:errorcluster)  [unwired: 1 in, 1 out]
      n178 = property on="数值 3" class="DigNum (严格)"(error in=w317, "Value"=0 ("数值 3")) -> (error out=w316:errorcluster)  [unwired: 1 in, 1 out]
      n179 = property on="所有数据3" class="Arr (严格)"(error in=w316, "Value"=string[][] [] ("所有数据3")) -> (error out=w315:errorcluster)  [unwired: 1 in, 1 out]
      n180 = property on="水质3" class="Arr (严格)"(error in=w315, "Value"=string[][] [] ("水质3")) -> (error out=w314:errorcluster)  [unwired: 1 in, 1 out]
      n181 = property on="温度3" class="Arr (严格)"(error in=w314, "Value"=string[][] [] ("温度3")) -> (error out=w313:errorcluster)  [unwired: 1 in, 1 out]
      n182 = property on="电压3" class="Arr (严格)"(error in=w313, "Value"=dbl[] [] ("电压3")) -> (error out=w312:errorcluster)  [unwired: 1 in, 1 out]
      n183 = property on="电流3" class="Arr (严格)"(error in=w312, "Value"=dbl[] [] ("电流3")) -> (error out=w311:errorcluster)  [unwired: 1 in, 1 out]
      n184 = property on="极化曲线3" class="Arr (严格)"(error in=w311, "Value"=dbl[][] [] ("极化曲线3")) -> (error out=w310:errorcluster)  [unwired: 1 in, 1 out]
      n185 = property on="数值 2" class="DigNum (严格)"(error in=w310, "Value"=w339) -> (error out=w338:errorcluster)  [unwired: 1 in, 1 out]
      n186 = property on="数值" class="DigNum (严格)"(error in=w338, "Value"=w339) -> (error out=w346:errorcluster)  [unwired: 1 in, 1 out]
      n187 = property on="温度1" class="Arr (严格)"(error in=w346, "Value"=string[][] [] ("温度1")) -> (error out=w344:errorcluster)  [unwired: 1 in, 1 out]
      n188 = property on="压力1" class="Arr (严格)"(error in=w344, "Value"=w345) -> (error out=w343:errorcluster)  [unwired: 1 in, 1 out]
      n189 = property on="压力2" class="Arr (严格)"(error in=w343, "Value"=w345) -> (error out=w342:errorcluster)  [unwired: 1 in, 1 out]
      n190 = property on="压力3" class="Arr (严格)"(error in=w342, "Value"=w345) -> (error out=w341:errorcluster)  [unwired: 1 in, 1 out]
      n191 = property on="压力4" class="Arr (严格)"(error in=w341, "Value"=w345) -> (error out=w340:errorcluster)  [unwired: 1 in, 1 out]
      n192 = property on="水质1" class="Arr (严格)"(error in=w340, "Value"=w345) -> (error out=w363:errorcluster)  [unwired: 1 in, 1 out]
      n193 = property on="所有数据" class="Arr (严格)"(error in=w363, "Value"=string[][] [] ("温度1")) -> (error out=w361:errorcluster)  [unwired: 1 in, 1 out]
      n194 = property on="极化曲线1" class="Arr (严格)"(error in=w361, "Value"=dbl[][] [] ("极化曲线1")) -> (error out=w360:errorcluster)  [unwired: 1 in, 1 out]
      n195 = property on="电流1" class="Arr (严格)"(error in=w360, "Value"=dbl[] [] ("电压1")) -> (error out=w359:errorcluster)  [unwired: 1 in, 1 out]
      n196 = property on="电压1" class="Arr (严格)"(error in=w359, "Value"=dbl[] [] ("电压1")) -> (error out=w353:errorcluster)  [unwired: 1 in, 1 out]
      n197 = property on="电压2" class="Arr (严格)"(error in=w353, "Value"=w356) -> (error out=w352:errorcluster)  [unwired: 1 in, 1 out]
      n198 = property on="电流2" class="Arr (严格)"(error in=w352, "Value"=w356) -> (error out=w351:errorcluster)  [unwired: 1 in, 1 out]
      n199 = property on="水质2" class="Arr (严格)"(error in=w351, "Value"=w355) -> (error out=w350:errorcluster)  [unwired: 1 in, 1 out]
      n200 = property on="温度2" class="Arr (严格)"(error in=w350, "Value"=w355) -> (error out=w349:errorcluster)  [unwired: 1 in, 1 out]
      n201 = property on="所有数据2" class="Arr (严格)"(error in=w349, "Value"=w355) -> (error out=w348:errorcluster)  [unwired: 1 in, 1 out]
      n202 = property on="极化曲线2" class="Arr (严格)"(error in=w348, "Value"=dbl[][] [] ("极化曲线1")) -> (error out=w347:errorcluster)  [unwired: 1 in, 1 out]
    }
  }
  n203 = flat-sequence {
    frame #0 {
      n204 = call <vilib>:"Application Directory.vi"() -> ("Application Directory"=w368:path)
      n205 = Build Path(base path=w368, name or relative path="1.jpg") -> (appended path=w366:path)
      n206 = call <vilib>:"Read JPEG File.vi"("path to JPEG file"=w366) -> ("image data"=w369:T6)  [unwired: 8 in, 2 out]
      n207 = call <vilib>:"Draw Flattened Pixmap.vi"("image data"=w369) -> ("new picture"=→"new picture":picture)  [unwired: 8 in]
    }
    frame #1 {
    }
    frame #2 {
      n208 = property on="new picture" class="Pict"("Draw Area Size"=T5 {"Width"=1776, "Height"=860} ("绘图区域大小")) -> ()  [unwired: 2 in, 2 out]
    }
  }
  n209 = property on="当前温度 2" class="DigNum (严格)" props=["Value"]() -> ()  [unwired: 2 in, 3 out]
  n210 = property on="温度1" class="Arr (严格)" props=["Value"]() -> ()  [unwired: 2 in, 3 out]
  n211 = property on="队列输出 2" class="TypRef (严格)" props=["Value"]() -> ()  [unwired: 2 in, 3 out]
  n212 = while {
    shift-right: [w373] -> _
    shift-left: FALSE -> [w372]
    tunnel: w39 -> [_]
    stop <- FALSE stop-if-true
    n213 = event shown="[1] \"1\", \"2\", \"3\", \"4\": 值改变" {
      selector: _ -> [_ _]
      dyn-events: _ -> [_ _]
      timeout: 100 -> [_ _]
      tunnel: [w376 w381] -> w373
      tunnel: w372 -> [_ w382]
      event Timeout {
        n214 = event-data() -> ()  [unwired: 1 in, 3 out]
        n215 = property on="1" class="Bool (严格)"() -> ("Value"=w380:bool)  [unwired: 2 in, 2 out]
        n216 = property on="2" class="Bool (严格)"() -> ("Value"=w379:bool)  [unwired: 2 in, 2 out]
        n217 = property on="3" class="Bool (严格)"() -> ("Value"=w378:bool)  [unwired: 2 in, 2 out]
        n218 = property on="4" class="Bool (严格)"() -> ("Value"=w377:bool)  [unwired: 2 in, 2 out]
        n219 = Compound Arithmetic op=OR ("复合运算")(w380, w379, w378, w377) -> (w376:bool)
      }
      event "1", "2", "3", "4": Value Change {
        n220 = event-data() -> ("CtlRef"=w384:refnum<vi>, "NewVal"=w383:bool)  [unwired: 1 in, 4 out]
        n221 = case shown="真" w383 {
          tunnel: w384 -> [w386 w426]
          tunnel: w382 -> [_ w425]
          tunnel: [_ w425] -> w381
          frame False {
            n222 = property class="Bool (严格)"(reference=w386) -> ("Label.Text"=w385:string)  [unwired: 1 in, 2 out]
            n223 = Scan From String(format string="%d" ("格式字符串"), input string=w385) -> (output 1=w387:i32)  [unwired: 3 in, 3 out]
            n224 = control-ref of="窗格 6"() -> (w391:refnum<vi>)
            n225 = control-ref of="窗格 7"() -> (w390:refnum<vi>)
            n226 = control-ref of="窗格 8"() -> (w389:refnum<vi>)
            n227 = control-ref of="窗格 9"() -> (w398:refnum<vi>)
            n228 = Build Array(w391, w390, w389, w398) -> (w388:refnum<vi>[])
            n229 = Decrement(x=w387) -> (x-1=w392:i32)
            n230 = Delete From Array(array=w388, length=1 ("长度"), index=w392) -> (deleted portion=w395:refnum<vi>[])  [unwired: 1 out]
            n231 = Index Array(array=w395, index=0 ("索引")) -> (element=w397:refnum<vi>)
            n232 = case shown="\"4\"" w385 {
              tunnel: w397 -> [_ w400 w405 w412 w421]
              frame "假", Default {
              }
              frame "1" {
                n233 = property class="Pane"(reference=w400, "Origin"=T7 {"Horizontal"=0, "Vertical"=0} ("原点")) -> ()  [unwired: 1 in, 2 out]
                n234 = property class="Pane"(reference=w400, "VertScrollbarVisibility"=T3."Always Off" ("垂直滚动条可见")) -> ()  [unwired: 1 in, 2 out]
                n235 = property on="分隔栏 5" class="Splitter"() -> ("Position"=w403:i32)  [unwired: 2 in, 2 out]
                n236 = Subtract(x=w403, y=751) -> (x-y=w404:i32)
                n237 = property on="分隔栏 5" class="Splitter"("Position"=w404) -> ()  [unwired: 2 in, 2 out]
              }
              frame "2" {
                n238 = property on="分隔栏 6" class="Splitter"() -> ("Position"=w409:i32)  [unwired: 2 in, 2 out]
                n239 = property class="Pane"(reference=w405, "Origin"=T7 {"Horizontal"=0, "Vertical"=0} ("原点")) -> ()  [unwired: 1 in, 2 out]
                n240 = property class="Pane"(reference=w405, "VertScrollbarVisibility"=T3."Always Off" ("垂直滚动条可见")) -> ()  [unwired: 1 in, 2 out]
                n241 = Subtract(x=w409, y=751) -> (x-y=w410:i32)
                n242 = property on="分隔栏 6" class="Splitter"("Position"=w410) -> ()  [unwired: 2 in, 2 out]
              }
              frame "3" {
                n243 = property class="Pane"(reference=w412, "VertScrollbarVisibility"=T3."Always Off" ("垂直滚动条可见")) -> (reference out=w411:refnum<vi>)  [unwired: 1 in, 1 out]
                n244 = property on="分隔栏 7" class="Splitter"() -> ("Position"=w416:i32)  [unwired: 2 in, 2 out]
                n245 = Subtract(x=w416, y=751) -> (x-y=w415:i32)
                n246 = property on="分隔栏 7" class="Splitter"("Position"=w415) -> ()  [unwired: 2 in, 2 out]
                n247 = property class="Pane"(reference=w411, "Origin"=T7 {"Horizontal"=0, "Vertical"=0} ("原点")) -> ()  [unwired: 1 in, 2 out]
              }
              frame "4" {
                n248 = property class="Pane"(reference=w421, "VertScrollbarVisibility"=T3."Always Off" ("垂直滚动条可见")) -> (reference out=w420:refnum<vi>)  [unwired: 1 in, 1 out]
                n249 = property on="分隔栏 8" class="Splitter"() -> ("Position"=w419:i32)  [unwired: 2 in, 2 out]
                n250 = Subtract(x=w419, y=751) -> (x-y=w418:i32)
                n251 = property on="分隔栏 8" class="Splitter"("Position"=w418) -> ()  [unwired: 2 in, 2 out]
                n252 = property class="Pane"(reference=w420, "Origin"=T7 {"Horizontal"=0, "Vertical"=0} ("原点")) -> ()  [unwired: 1 in, 2 out]
              }
            }
          }
          frame True {
            n253 = case shown="真" w425 {
              tunnel: w426 -> [w437 w458]
              frame False {
                n254 = property class="Bool (严格)"(reference=w437) -> ("Label.Text"=w432:string)  [unwired: 1 in, 2 out]
                n255 = Scan From String(format string="%d" ("格式字符串"), input string=w432) -> (output 1=w430:i32)  [unwired: 3 in, 3 out]
                n256 = control-ref of="窗格 6"() -> (w435:refnum<vi>)
                n257 = control-ref of="窗格 7"() -> (w434:refnum<vi>)
                n258 = control-ref of="窗格 8"() -> (w433:refnum<vi>)
                n259 = control-ref of="窗格 9"() -> (w436:refnum<vi>)
                n260 = Decrement(x=w430) -> (x-1=w429:i32)
                n261 = Build Array(w435, w434, w433, w436) -> (w428:refnum<vi>[])
                n262 = Delete From Array(array=w428, index=w429) -> (deleted portion=w427:refnum<vi>)  [unwired: 1 in, 1 out]
                n263 = case shown="\"2\"" w432 {
                  tunnel: w427 -> [_ w439 w443 w448 w455]
                  frame "假", Default {
                  }
                  frame "1" {
                    n264 = property class="Pane"(reference=w439, "VertScrollbarVisibility"=T3."Always On" ("垂直滚动条可见")) -> ()  [unwired: 1 in, 2 out]
                    n265 = property on="分隔栏 5" class="Splitter"() -> ("Position"=w441:i32)  [unwired: 2 in, 2 out]
                    n266 = Add(x=w441, y=751) -> (x+y=w442:i32)
                    n267 = property on="分隔栏 5" class="Splitter"("Position"=w442) -> ()  [unwired: 2 in, 2 out]
                  }
                  frame "2" {
                    n268 = property class="Pane"(reference=w443, "VertScrollbarVisibility"=T3."Always On" ("垂直滚动条可见")) -> ()  [unwired: 1 in, 2 out]
                    n269 = property on="分隔栏 6" class="Splitter"() -> ("Position"=w446:i32)  [unwired: 2 in, 2 out]
                    n270 = Add(x=w446, y=751) -> (x+y=w447:i32)
                    n271 = property on="分隔栏 6" class="Splitter"("Position"=w447) -> ()  [unwired: 2 in, 2 out]
                  }
                  frame "3" {
                    n272 = property class="Pane"(reference=w448, "VertScrollbarVisibility"=T3."Always On" ("垂直滚动条可见")) -> ()  [unwired: 1 in, 2 out]
                    n273 = property on="分隔栏 7" class="Splitter"() -> ("Position"=w451:i32)  [unwired: 2 in, 2 out]
                    n274 = Add(x=w451, y=751) -> (x+y=w450:i32)
                    n275 = property on="分隔栏 7" class="Splitter"("Position"=w450) -> ()  [unwired: 2 in, 2 out]
                  }
                  frame "4" {
                    n276 = property class="Pane"(reference=w455, "VertScrollbarVisibility"=T3."Always On" ("垂直滚动条可见")) -> ()  [unwired: 1 in, 2 out]
                    n277 = property on="分隔栏 8" class="Splitter"() -> ("Position"=w454:i32)  [unwired: 2 in, 2 out]
                    n278 = Add(x=w454, y=751) -> (x+y=w453:i32)
                    n279 = property on="分隔栏 8" class="Splitter"("Position"=w453) -> ()  [unwired: 2 in, 2 out]
                  }
                }
              }
              frame True {
                n280 = stacked-sequence {
                  tunnel: w458 -> [w466 _]
                  tunnel: w458 -> [_ w516]
                  frame #0 {
                    n281 = control-ref of="1"() -> (w467:refnum<vi>)
                    n282 = control-ref of="2"() -> (w468:refnum<vi>)
                    n283 = control-ref of="3"() -> (w469:refnum<vi>)
                    n284 = control-ref of="4"() -> (w470:refnum<vi>)
                    n285 = property class="Bool (严格)"(reference=w466) -> ("Label.Text"=w465:string)  [unwired: 1 in, 2 out]
                    n286 = Scan From String(format string="%d" ("格式字符串"), input string=w465) -> (output 1=w463:i32)  [unwired: 3 in, 3 out]
                    n287 = Build Array(w467, w468, w469, w470) -> (w460:refnum<vi>[])
                    n288 = Decrement(x=w463) -> (x-1=w462:i32)
                    n289 = Delete From Array(array=w460, length=1 ("长度"), index=w462) -> (array with subset deleted=w459:refnum<vi>[])  [unwired: 1 out]
                    n290 = for {
                      tunnel: w459 -> [w472] mode=indexing
                      n291 = property class="Bool (严格)"(reference=w472) -> ("Value"=w471:bool)  [unwired: 1 in, 2 out]
                      n292 = Equal?(x=w471, y=TRUE) -> (x = y?=w473:bool)
                      n293 = case shown="真" w473 {
                        tunnel: w472 -> [_ w476]
                        frame False {
                        }
                        frame True {
                          n294 = property class="Bool (严格)"(reference=w476) -> ("Label.Text"=w480:string)  [unwired: 1 in, 2 out]
                          n295 = property class="Bool (严格)"(reference=w476, "Value"=FALSE ("值")) -> ()  [unwired: 1 in, 2 out]
                          n296 = Scan From String(format string="%d" ("格式字符串"), input string=w480) -> (output 1=w475:i32)  [unwired: 3 in, 3 out]
                          n297 = control-ref of="窗格 6"() -> (w484:refnum<vi>)
                          n298 = control-ref of="窗格 7"() -> (w483:refnum<vi>)
                          n299 = control-ref of="窗格 8"() -> (w482:refnum<vi>)
                          n300 = control-ref of="窗格 9"() -> (w488:refnum<vi>)
                          n301 = Decrement(x=w475) -> (x-1=w485:i32)
                          n302 = Build Array(w484, w483, w482, w488) -> (w481:refnum<vi>[])
                          n303 = Delete From Array(array=w481, length=1 ("长度"), index=w485) -> (deleted portion=w486:refnum<vi>[])  [unwired: 1 out]
                          n304 = Index Array(array=w486, index=0 ("索引")) -> (element=w487:refnum<vi>)
                          n305 = case shown="\"1\"" w480 {
                            tunnel: w487 -> [_ w491 w496 w503 w512]
                            frame "假", Default {
                            }
                            frame "1" {
                              n306 = property class="Pane"(reference=w491, "Origin"=T7 {"Horizontal"=0, "Vertical"=0} ("原点")) -> ()  [unwired: 1 in, 2 out]
                              n307 = property class="Pane"(reference=w491, "VertScrollbarVisibility"=T3."Always Off" ("垂直滚动条可见")) -> ()  [unwired: 1 in, 2 out]
                              n308 = property on="分隔栏 5" class="Splitter"() -> ("Position"=w494:i32)  [unwired: 2 in, 2 out]
                              n309 = Subtract(x=w494, y=751) -> (x-y=w495:i32)
                              n310 = property on="分隔栏 5" class="Splitter"("Position"=w495) -> ()  [unwired: 2 in, 2 out]
                            }
                            frame "2" {
                              n311 = property class="Pane"(reference=w496, "Origin"=T7 {"Horizontal"=0, "Vertical"=0} ("原点")) -> ()  [unwired: 1 in, 2 out]
                              n312 = property class="Pane"(reference=w496, "VertScrollbarVisibility"=T3."Always Off" ("垂直滚动条可见")) -> ()  [unwired: 1 in, 2 out]
                              n313 = property on="分隔栏 6" class="Splitter"() -> ("Position"=w500:i32)  [unwired: 2 in, 2 out]
                              n314 = Subtract(x=w500, y=751) -> (x-y=w501:i32)
                              n315 = property on="分隔栏 6" class="Splitter"("Position"=w501) -> ()  [unwired: 2 in, 2 out]
                            }
                            frame "3" {
                              n316 = property class="Pane"(reference=w503, "VertScrollbarVisibility"=T3."Always Off" ("垂直滚动条可见")) -> (reference out=w502:refnum<vi>)  [unwired: 1 in, 1 out]
                              n317 = property on="分隔栏 7" class="Splitter"() -> ("Position"=w507:i32)  [unwired: 2 in, 2 out]
                              n318 = Subtract(x=w507, y=751) -> (x-y=w506:i32)
                              n319 = property on="分隔栏 7" class="Splitter"("Position"=w506) -> ()  [unwired: 2 in, 2 out]
                              n320 = property class="Pane"(reference=w502, "Origin"=T7 {"Horizontal"=0, "Vertical"=0} ("原点")) -> ()  [unwired: 1 in, 2 out]
                            }
                            frame "4" {
                              n321 = property class="Pane"(reference=w512, "VertScrollbarVisibility"=T3."Always Off" ("垂直滚动条可见")) -> (reference out=w511:refnum<vi>)  [unwired: 1 in, 1 out]
                              n322 = property on="分隔栏 8" class="Splitter"() -> ("Position"=w510:i32)  [unwired: 2 in, 2 out]
                              n323 = Subtract(x=w510, y=751) -> (x-y=w509:i32)
                              n324 = property on="分隔栏 8" class="Splitter"("Position"=w509) -> ()  [unwired: 2 in, 2 out]
                              n325 = property class="Pane"(reference=w511, "Origin"=T7 {"Horizontal"=0, "Vertical"=0} ("原点")) -> ()  [unwired: 1 in, 2 out]
                            }
                          }
                        }
                      }
                    }
                  }
                  frame #1 {
                    n326 = property class="Bool (严格)"(reference=w516) -> ("Label.Text"=w522:string)  [unwired: 1 in, 2 out]
                    n327 = Scan From String(format string="%d" ("格式字符串"), input string=w522) -> (output 1=w521:i32)  [unwired: 3 in, 3 out]
                    n328 = control-ref of="窗格 6"() -> (w525:refnum<vi>)
                    n329 = control-ref of="窗格 7"() -> (w524:refnum<vi>)
                    n330 = control-ref of="窗格 8"() -> (w523:refnum<vi>)
                    n331 = control-ref of="窗格 9"() -> (w526:refnum<vi>)
                    n332 = Decrement(x=w521) -> (x-1=w520:i32)
                    n333 = Build Array(w525, w524, w523, w526) -> (w519:refnum<vi>[])
                    n334 = Delete From Array(array=w519, index=w520) -> (deleted portion=w518:refnum<vi>)  [unwired: 1 in, 1 out]
                    n335 = case shown="\"4\"" w522 {
                      tunnel: w518 -> [_ w528 w532 w537 w544]
                      frame "假", Default {
                      }
                      frame "1" {
                        n336 = property on="分隔栏 5" class="Splitter"() -> ("Position"=w530:i32)  [unwired: 2 in, 2 out]
                        n337 = property class="Pane"(reference=w528, "VertScrollbarVisibility"=T3."Always On" ("垂直滚动条可见")) -> ()  [unwired: 1 in, 2 out]
                        n338 = Add(x=w530, y=751) -> (x+y=w531:i32)
                        n339 = property on="分隔栏 5" class="Splitter"("Position"=w531) -> ()  [unwired: 2 in, 2 out]
                      }
                      frame "2" {
                        n340 = property on="分隔栏 6" class="Splitter"() -> ("Position"=w535:i32)  [unwired: 2 in, 2 out]
                        n341 = property class="Pane"(reference=w532, "VertScrollbarVisibility"=T3."Always On" ("垂直滚动条可见")) -> ()  [unwired: 1 in, 2 out]
                        n342 = Add(x=w535, y=751) -> (x+y=w536:i32)
                        n343 = property on="分隔栏 6" class="Splitter"("Position"=w536) -> ()  [unwired: 2 in, 2 out]
                      }
                      frame "3" {
                        n344 = property on="分隔栏 7" class="Splitter"() -> ("Position"=w540:i32)  [unwired: 2 in, 2 out]
                        n345 = property class="Pane"(reference=w537, "VertScrollbarVisibility"=T3."Always On" ("垂直滚动条可见")) -> ()  [unwired: 1 in, 2 out]
                        n346 = Add(x=w540, y=751) -> (x+y=w539:i32)
                        n347 = property on="分隔栏 7" class="Splitter"("Position"=w539) -> ()  [unwired: 2 in, 2 out]
                      }
                      frame "4" {
                        n348 = property on="分隔栏 8" class="Splitter"() -> ("Position"=w543:i32)  [unwired: 2 in, 2 out]
                        n349 = property class="Pane"(reference=w544, "VertScrollbarVisibility"=T3."Always On" ("垂直滚动条可见")) -> ()  [unwired: 1 in, 2 out]
                        n350 = Add(x=w543, y=751) -> (x+y=w542:i32)
                        n351 = property on="分隔栏 8" class="Splitter"("Position"=w542) -> ()  [unwired: 2 in, 2 out]
                      }
                    }
                  }
                }
              }
            }
          }
        }
      }
    }
  }
  n352 = property on="窗格" class="Pane"() -> ("Decos[]"=w36:refnum<vi>[])  [unwired: 2 in, 2 out]
  n353 = for {
    tunnel: w36 -> [w548] mode=indexing
    n354 = property class="Decor"(reference=w548, "Visible"=TRUE ("可见")) -> ()  [unwired: 1 in, 2 out]
  }
  n355 = disable-structure shown="禁用" {
    disable-tunnel: [w550 _] -> w38
    frame Disabled {
      w558 = u16 0 items=["无", "奇", "偶"] ("parity (Even)")
      n356 = To Variant() -> (anything=w549:cluster{}, Variant=w555:variant)
      n357 = Variant To Data(type="", Variant=w555) -> (data=→"数据":string)  [unwired: 1 in, 1 out]
      n358 = call-poly <vilib>:"Create Master Instance.vi"("serial type"=enum16{"RTU", "ASCII"}."RTU", "parity (Even)"=w558, "unit ID"=u8 1, "baud rate (9600)"=u32 9600, "VISA resource name"=w549) -> ("error out"=w552:errorcluster, "serial master instance"=w550:refnum<class "Modbus Master.lvclass">)  [unwired: 5 in]
      n359 = property on="字符串" class="Str"("Value"="1" ("字符串")) -> ()  [unwired: 2 in, 2 out]
      n360 = while {
        tunnel: w550 -> [w563]
        tunnel: w552 -> [w561]
        stop <- FALSE stop-if-true
        n361 = Wait (ms)(milliseconds to wait=u32 100 ("等待时间（毫秒）")) -> ()  [unwired: 1 out]
        n362 = case shown="\"1\", 默认" "字符串" {
          tunnel: w563 -> [w576 w592 _]
          tunnel: w561 -> [w575 w591 _]
          tunnel: [w572 w582 _] -> _
          tunnel: [w571 w581 _] -> _
          frame "1", Default {
            n363 = call-dynamic "Read Holding Registers.vi"("error in (no error)"=w575, "number of holding registers"=u16 1, "starting address"=u16 258, "Modbus master in"=w576) -> ("error out"=w571:errorcluster, "register values"=w570:u16[], "Modbus master out"=w572:refnum<class "Modbus Master.lvclass">)  [unwired: 5 in]
            "error out" <- w571
            n364 = Index Array(array=w570, index=0 ("索引")) -> (element=w568:u16)
            n365 = To Double Precision Float(number=w568) -> (double precision float=w567:dbl)
            n366 = Divide(x=w567, y=10.0) -> (x/y=→"当前温度 2":dbl)
          }
          frame "2" {
            n367 = call-dynamic "Read Holding Registers.vi"("error in (no error)"=w591, "number of holding registers"=u16 1, "starting address"=u16 258, "Modbus master in"=w592) -> ("error out"=w581:errorcluster, "register values"=w588:u16[], "Modbus master out"=w582:refnum<class "Modbus Master.lvclass">)  [unwired: 5 in]
            n368 = Index Array(array=w588, index=0 ("索引")) -> (element=w586:u16)
            n369 = To Double Precision Float(number=w586) -> (double precision float=w585:dbl)
            n370 = Divide(x=w585, y=10.0) -> (x/y=w577:dbl)
            n371 = Divide(x="文本下拉列表", y=u16 100) -> (x/y=w579:dbl)
            n372 = Greater Or Equal?(x=w577, y=w579) -> (x >= y?=w583:bool)
            n373 = case shown="真" w583 {
              tunnel: w582 -> [_ w594]
              tunnel: w581 -> [_ w593]
              frame False {
              }
              frame True {
                n374 = flat-sequence {
                  tunnel: w594 -> [w596]
                  tunnel: w593 -> [w595]
                  frame #0 {
                    n375 = call-dynamic "Write Single Holding Register.vi"("error in (no error)"=w595, "holding register value"=u16 2, "address"=u16 56, "Modbus master in"=w596) -> ()  [unwired: 6 in, 2 out]
                  }
                  frame #1 {
                    n376 = property on="字符串" class="Str"("Value"="1" ("字符串")) -> ()  [unwired: 2 in, 2 out]
                  }
                }
              }
            }
          }
          frame "0" {
          }
        }
      }
    }
    frame Enabled {
    }
  }
  n377 = while {
    tunnel: w38 -> [w600]
    tunnel: w1 -> [_]
    stop <- FALSE stop-if-true
    n378 = event shown="[1] \"保存所有\", \"配置\", \"连接\", \"分析\": 鼠标按下" {
      selector: _ -> [_ _ _ _ _ _ _ _ _ _ _ _ _ _ _ _ _ _ _ _ _ _ _ _ _ _ _ _]
      dyn-events: _ -> [_ _ _ _ _ _ _ _ _ _ _ _ _ _ _ _ _ _ _ _ _ _ _ _ _ _ _ _]
      timeout: 100 -> [_ _ _ _ _ _ _ _ _ _ _ _ _ _ _ _ _ _ _ _ _ _ _ _ _ _ _ _]
      tunnel: w600 -> [_ _ _ _ _ _ _ _ _ _ _ _ _ _ _ _ _ _ _ _ _ _ _ _ _ w2554 _ _]
      event Timeout {
        n379 = event-data() -> ()  [unwired: 1 in, 3 out]
      }
      event "保存所有", "配置", "连接", "分析": Mouse Down {
        n380 = event-data() -> ("CtlRef"=w604:refnum<vi>)  [unwired: 1 in, 7 out]
        n381 = flat-sequence {
          tunnel: w604 -> [w606]
          tunnel: [w605] -> w603
          tunnel: w603 -> [w628]
          frame #0 {
            n382 = property class="Bool (严格)"(reference=w606) -> ("Label.Text"=w605:string)  [unwired: 1 in, 2 out]
            n383 = disable-structure shown="禁用" {
              disable-tunnel: w605 -> [w607 _]
              frame Disabled {
                # "6"
                # "4"
                n384 = Search 1D Array(1D array=string[] ["保存所有", "分析", "配置", "连接", "退出"], element=w607, start index (0)=0 ("开始索引(0)")) -> (index of element=w613:i32)
                n385 = Delete From Array(array=i32[] [0, 0, 0, 0, 0, 0, 0, 0], length=1 ("长度"), index=w613) -> (deleted portion=w610:i32[], array with subset deleted=w611:i32[])
                n386 = Index Array(array=w610, index=0 ("索引")) -> (element=w608:i32)
                n387 = flat-sequence {
                  tunnel: w611 -> [w619]
                  tunnel: [w618] -> w617
                  tunnel: w608 -> [w618]
                  tunnel: w617 -> [w625]
                  frame #0 {
                    n388 = for {
                      tunnel: w619 -> [w623] mode=indexing
                      n389 = property on="窗格" class="Pane"() -> ("Decos[]"=w620:refnum<vi>[])  [unwired: 2 in, 2 out]
                      n390 = Index Array(array=w620, index=w623) -> (element=w622:refnum<vi>)
                      n391 = property class="Decor"(reference=w622, "Visible"=TRUE ("可见")) -> ()  [unwired: 1 in, 2 out]
                    }
                  }
                  frame #1 {
                    n392 = property on="窗格" class="Pane"() -> ("Decos[]"=w624:refnum<vi>[])  [unwired: 2 in, 2 out]
                    n393 = Index Array(array=w624, index=w625) -> (element=w626:refnum<vi>)
                    n394 = property class="Decor"(reference=w626, "Visible"=TRUE ("可见")) -> ()  [unwired: 1 in, 2 out]
                  }
                }
              }
              frame Enabled {
              }
            }
          }
          frame #1 {
            n395 = case shown="\"分析\"" w628 {
              frame "假", Default {
              }
              frame "连接" {
                n396 = disable-structure shown="禁用" {
                  frame Disabled {
                    n397 = control-ref of="冷凝器液位 2"() -> (w645:refnum<vi>)
                    n398 = control-ref of="露点仪 2"() -> (w644:refnum<vi>)
                    n399 = control-ref of="微量氧 2"() -> (w643:refnum<vi>)
                    n400 = control-ref of="纯度仪 2"() -> (w642:refnum<vi>)
                    n401 = control-ref of="气分液位 2"() -> (w641:refnum<vi>)
                    n402 = control-ref of="电解电压 2"() -> (w640:refnum<vi>)
                    n403 = control-ref of="电解电流 2"() -> (w639:refnum<vi>)
                    n404 = control-ref of="水质电导率 2"() -> (w638:refnum<vi>)
                    n405 = control-ref of="循环水压 2"() -> (w637:refnum<vi>)
                    n406 = control-ref of="冷却水水压 2"() -> (w636:refnum<vi>)
                    n407 = control-ref of="氢渗 2"() -> (w635:refnum<vi>)
                    n408 = control-ref of="氢中氧 2"() -> (w634:refnum<vi>)
                    n409 = control-ref of="水箱温度 2"() -> (w633:refnum<vi>)
                    n410 = control-ref of="水箱液位 2"() -> (w632:refnum<vi>)
                    n411 = Build Array(w645, w644, w643, w642, w641, w640, w639, w638, w637, w636, w635, w634, w633, w632) -> (w631:refnum<vi>[])
                    n412 = control-ref of="冷凝器液位"() -> (w660:refnum<vi>)
                    n413 = control-ref of="露点仪"() -> (w659:refnum<vi>)
                    n414 = control-ref of="微量氧"() -> (w658:refnum<vi>)
                    n415 = control-ref of="纯度仪"() -> (w657:refnum<vi>)
                    n416 = control-ref of="气分液位"() -> (w656:refnum<vi>)
                    n417 = control-ref of="电解电压"() -> (w655:refnum<vi>)
                    n418 = control-ref of="电解电流"() -> (w654:refnum<vi>)
                    n419 = control-ref of="水质电导率"() -> (w653:refnum<vi>)
                    n420 = control-ref of="循环水压"() -> (w652:refnum<vi>)
                    n421 = control-ref of="冷却水水压"() -> (w651:refnum<vi>)
                    n422 = control-ref of="氢渗"() -> (w650:refnum<vi>)
                    n423 = control-ref of="氢中氧"() -> (w649:refnum<vi>)
                    n424 = control-ref of="水箱温度"() -> (w648:refnum<vi>)
                    n425 = control-ref of="水箱液位"() -> (w647:refnum<vi>)
                    n426 = Build Array(w660, w659, w658, w657, w656, w655, w654, w653, w652, w651, w650, w649, w648, w647) -> (w646:refnum<vi>[])
                    n427 = for {
                      tunnel: w646 -> [w664] mode=indexing
                      tunnel: w631 -> [w662] mode=indexing
                      n428 = property class="Str"(reference=w662, "Visible"=TRUE ("可见")) -> ()  [unwired: 1 in, 2 out]
                      n429 = property class="Str"(reference=w664, "Visible"=FALSE ("可见")) -> ()  [unwired: 1 in, 2 out]
                    }
                  }
                  frame Enabled {
                  }
                }
                n430 = property on="new picture" class="Pict"("ZoomFactor"=sgl 0.73 ("缩放因子")) -> ()  [unwired: 2 in, 2 out]
                n431 = property on="选项卡控件 2" class="TabCtl (严格)"("Value"=T2."工步 2" ("选项卡控件 2")) -> ()  [unwired: 2 in, 2 out]
                n432 = flat-sequence {
                  frame #0 {
                    n433 = property on="分隔栏 3" class="Splitter"() -> ("Position"=w667:i32)  [unwired: 2 in, 2 out]
                    n434 = Equal?(x=w667, y=116) -> (x = y?=w665:bool)
                    n435 = case shown="假" w665 {
                      frame False {
                        n436 = property on="分隔栏 3" class="Splitter"() -> ("Position"=w669:i32)  [unwired: 2 in, 2 out]
                        n437 = Greater?(x=w669, y=508) -> (0:w668:bool)
                        n438 = case shown="真" w668 {
                          frame False {
                          }
                          frame True {
                            n439 = while {
                              i -> [w678]
                              stop <- w671 stop-if-true
                              n440 = Multiply(x=50, y=w678) -> (x*y=w675:i32)
                              n441 = Subtract(x=509, y=w675) -> (x-y=w672:i32)
                              n442 = Less?(x=w672, y=166) -> (x < y?=w673:bool)
                              n443 = case shown="假" w673 {
                                tunnel: w672 -> [w679 _]
                                tunnel: [FALSE TRUE] -> w671
                                frame False {
                                n444 = property on="分隔栏 3" class="Splitter"("Position"=w679) -> ()  [unwired: 2 in, 2 out]
                                }
                                frame True {
                                n445 = property on="分隔栏 3" class="Splitter"("Position"=116 ("分隔栏位置")) -> ()  [unwired: 2 in, 2 out]
                                }
                              }
                            }
                          }
                        }
                      }
                      frame True {
                      }
                    }
                  }
                  frame #1 {
                    n446 = property on="分隔栏 2" class="Splitter"() -> ("Position"=w685:i32)  [unwired: 2 in, 2 out]
                    n447 = Equal?(x=w685, y=113) -> (x = y?=w684:bool)
                    n448 = case shown="真" w684 {
                      frame True {
                        n449 = while {
                          i -> [w693]
                          stop <- w686 stop-if-true
                          n450 = Multiply(x=50, y=w693) -> (x*y=w690:i32)
                          n451 = Add(x=113, y=w690) -> (x+y=w687:i32)
                          n452 = Greater?(x=w687, y=398) -> (0:w688:bool)
                          n453 = case shown="真" w688 {
                            tunnel: w687 -> [w694 _]
                            tunnel: [FALSE TRUE] -> w686
                            frame False {
                              n454 = property on="分隔栏 2" class="Splitter"("Position"=w694) -> ()  [unwired: 2 in, 2 out]
                            }
                            frame True {
                              n455 = property on="分隔栏 2" class="Splitter"("Position"=505 ("分隔栏位置")) -> ()  [unwired: 2 in, 2 out]
                            }
                          }
                        }
                      }
                      frame False {
                        n456 = while {
                          i -> [w705]
                          stop <- w698 stop-if-true
                          n457 = Multiply(x=50, y=w705) -> (x*y=w702:i32)
                          n458 = Subtract(x=448, y=w702) -> (x-y=w699:i32)
                          n459 = Less?(x=w699, y=163) -> (x < y?=w700:bool)
                          n460 = case shown="真" w700 {
                            tunnel: w699 -> [w706 _]
                            tunnel: [FALSE TRUE] -> w698
                            frame False {
                              n461 = property on="分隔栏 2" class="Splitter"("Position"=w706) -> ()  [unwired: 2 in, 2 out]
                            }
                            frame True {
                              n462 = property on="分隔栏 2" class="Splitter"("Position"=113 ("分隔栏位置")) -> ()  [unwired: 2 in, 2 out]
                            }
                          }
                        }
                      }
                    }
                  }
                }
              }
              frame "配置" {
                n463 = property on="选项卡控件 2" class="TabCtl (严格)"("Value"=T2."    设置界面" ("选项卡控件 2")) -> ()  [unwired: 2 in, 2 out]
                n464 = disable-structure shown="禁用" {
                  frame Disabled {
                    n465 = control-ref of="冷凝器液位 2"() -> (w726:refnum<vi>)
                    n466 = control-ref of="露点仪 2"() -> (w725:refnum<vi>)
                    n467 = control-ref of="微量氧 2"() -> (w724:refnum<vi>)
                    n468 = control-ref of="纯度仪 2"() -> (w723:refnum<vi>)
                    n469 = control-ref of="气分液位 2"() -> (w722:refnum<vi>)
                    n470 = control-ref of="电解电压 2"() -> (w721:refnum<vi>)
                    n471 = control-ref of="电解电流 2"() -> (w720:refnum<vi>)
                    n472 = control-ref of="水质电导率 2"() -> (w719:refnum<vi>)
                    n473 = control-ref of="循环水压 2"() -> (w718:refnum<vi>)
                    n474 = control-ref of="冷却水水压 2"() -> (w717:refnum<vi>)
                    n475 = control-ref of="氢渗 2"() -> (w716:refnum<vi>)
                    n476 = control-ref of="氢中氧 2"() -> (w715:refnum<vi>)
                    n477 = control-ref of="水箱温度 2"() -> (w714:refnum<vi>)
                    n478 = control-ref of="水箱液位 2"() -> (w713:refnum<vi>)
                    n479 = Build Array(w726, w725, w724, w723, w722, w721, w720, w719, w718, w717, w716, w715, w714, w713) -> (w712:refnum<vi>[])
                    n480 = control-ref of="冷凝器液位"() -> (w741:refnum<vi>)
                    n481 = control-ref of="露点仪"() -> (w740:refnum<vi>)
                    n482 = control-ref of="微量氧"() -> (w739:refnum<vi>)
                    n483 = control-ref of="纯度仪"() -> (w738:refnum<vi>)
                    n484 = control-ref of="气分液位"() -> (w737:refnum<vi>)
                    n485 = control-ref of="电解电压"() -> (w736:refnum<vi>)
                    n486 = control-ref of="电解电流"() -> (w735:refnum<vi>)
                    n487 = control-ref of="水质电导率"() -> (w734:refnum<vi>)
                    n488 = control-ref of="循环水压"() -> (w733:refnum<vi>)
                    n489 = control-ref of="冷却水水压"() -> (w732:refnum<vi>)
                    n490 = control-ref of="氢渗"() -> (w731:refnum<vi>)
                    n491 = control-ref of="氢中氧"() -> (w730:refnum<vi>)
                    n492 = control-ref of="水箱温度"() -> (w729:refnum<vi>)
                    n493 = control-ref of="水箱液位"() -> (w728:refnum<vi>)
                    n494 = Build Array(w741, w740, w739, w738, w737, w736, w735, w734, w733, w732, w731, w730, w729, w728) -> (w727:refnum<vi>[])
                    n495 = for {
                      tunnel: w727 -> [w745] mode=indexing
                      tunnel: w712 -> [w743] mode=indexing
                      n496 = property class="Str"(reference=w743, "Visible"=TRUE ("可见")) -> ()  [unwired: 1 in, 2 out]
                      n497 = property class="Str"(reference=w745, "Visible"=FALSE ("可见")) -> ()  [unwired: 1 in, 2 out]
                    }
                  }
                  frame Enabled {
                  }
                }
                n498 = property on="new picture" class="Pict"("ZoomFactor"=sgl 0.73 ("缩放因子")) -> ()  [unwired: 2 in, 2 out]
                n499 = flat-sequence {
                  frame #0 {
                    n500 = property on="分隔栏 2" class="Splitter"() -> ("Position"=w746:i32)  [unwired: 2 in, 2 out]
                    n501 = Equal?(x=w746, y=113) -> (x = y?=w747:bool)
                    n502 = case shown="假" w747 {
                      frame False {
                        n503 = while {
                          i -> [w756]
                          stop <- w749 stop-if-true
                          n504 = Multiply(x=50, y=w756) -> (x*y=w753:i32)
                          n505 = Subtract(x=448, y=w753) -> (x-y=w750:i32)
                          n506 = Less?(x=w750, y=163) -> (x < y?=w751:bool)
                          n507 = case shown="真" w751 {
                            tunnel: w750 -> [w757 _]
                            tunnel: [FALSE TRUE] -> w749
                            frame False {
                              n508 = property on="分隔栏 2" class="Splitter"("Position"=w757) -> ()  [unwired: 2 in, 2 out]
                            }
                            frame True {
                              n509 = property on="分隔栏 2" class="Splitter"("Position"=113 ("分隔栏位置")) -> ()  [unwired: 2 in, 2 out]
                            }
                          }
                        }
                      }
                      frame True {
                      }
                    }
                  }
                  frame #1 {
                    n510 = property on="分隔栏 3" class="Splitter"() -> ("Position"=w761:i32)  [unwired: 2 in, 2 out]
                    n511 = Equal?(x=w761, y=116) -> (x = y?=w763:bool)
                    n512 = case shown="假" w763 {
                      frame True {
                        n513 = while {
                          i -> [w771]
                          stop <- w764 stop-if-true
                          n514 = Multiply(x=50, y=w771) -> (x*y=w768:i32)
                          n515 = Add(x=116, y=w768) -> (x+y=w765:i32)
                          n516 = Greater?(x=w765, y=459) -> (0:w766:bool)
                          n517 = case shown="真" w766 {
                            tunnel: w765 -> [w772 _]
                            tunnel: [FALSE TRUE] -> w764
                            frame False {
                              n518 = property on="分隔栏 3" class="Splitter"("Position"=w772) -> ()  [unwired: 2 in, 2 out]
                            }
                            frame True {
                              n519 = property on="分隔栏 3" class="Splitter"("Position"=509 ("分隔栏位置")) -> ()  [unwired: 2 in, 2 out]
                            }
                          }
                        }
                      }
                      frame False {
                        n520 = while {
                          i -> [w783]
                          stop <- w776 stop-if-true
                          n521 = Multiply(x=50, y=w783) -> (x*y=w780:i32)
                          n522 = Subtract(x=509, y=w780) -> (x-y=w777:i32)
                          n523 = Less?(x=w777, y=166) -> (x < y?=w778:bool)
                          n524 = case shown="真" w778 {
                            tunnel: w777 -> [w784 _]
                            tunnel: [FALSE TRUE] -> w776
                            frame False {
                              n525 = property on="分隔栏 3" class="Splitter"("Position"=w784) -> ()  [unwired: 2 in, 2 out]
                            }
                            frame True {
                              n526 = property on="分隔栏 3" class="Splitter"("Position"=116 ("分隔栏位置")) -> ()  [unwired: 2 in, 2 out]
                            }
                          }
                        }
                      }
                    }
                  }
                }
              }
              frame "保存所有" {
              }
              frame "分析" {
                n527 = invoke on="子面板10" class="SubPnl" method="Remove VI"() -> ()  [unwired: 3 in, 3 out]
                n528 = property on="测试项目" class="RadioBtnsControl (严格)"() -> ("Value"=w788:enum32{"EIS", "极化曲线", "耐久性曲线", "线性扫描"})  [unwired: 2 in, 2 out]
                n529 = case shown="\"极化曲线\"" w788 {
                  frame "EIS", Default {
                  }
                  frame "极化曲线" {
                    n530 = flat-sequence {
                      frame #0 {
                        n531 = flat-sequence {
                          frame #0 {
                            n532 = property on="选项卡控件 2" class="TabCtl (严格)"("Value"=T2."所有数据" ("选项卡控件 2")) -> ()  [unwired: 2 in, 2 out]
                            n533 = property on="数组 3" class="Arr (严格)"() -> ("Value"=w790:refnum<vi>[])  [unwired: 2 in, 2 out]
                            n534 = for {
                              tunnel: w790 -> [w792] mode=indexing
                              n535 = property class="VI"(reference=w792) -> ("Name"=w793:string)  [unwired: 1 in, 2 out]
                              n536 = case shown="\"极化曲线.vi\", 默认" w793 {
                                tunnel: w792 -> [w794 w795 w796 w797 w798 _]
                                frame "极化曲线.vi", Default {
                                n537 = invoke on="子面板6" class="SubPnl" method="Remove VI"() -> ()  [unwired: 3 in, 3 out]
                                n538 = invoke on="子面板2" class="SubPnl" method="Insert VI"("VI Ref"=w794) -> ()  [unwired: 3 in, 4 out]
                                }
                                frame "温度.vi" {
                                n539 = invoke on="子面板3" class="SubPnl" method="Insert VI"("VI Ref"=w795) -> ()  [unwired: 3 in, 4 out]
                                }
                                frame "压力.vi" {
                                n540 = invoke on="子面板4" class="SubPnl" method="Insert VI"("VI Ref"=w796) -> ()  [unwired: 3 in, 4 out]
                                }
                                frame "水质.vi" {
                                n541 = invoke on="子面板5" class="SubPnl" method="Insert VI"("VI Ref"=w797) -> ()  [unwired: 3 in, 4 out]
                                }
                                frame "工步列表.vi" {
                                n542 = invoke on="子面板1" class="SubPnl" method="Insert VI"("VI Ref"=w798) -> ()  [unwired: 3 in, 4 out]
                                }
                                frame "列表.vi" {
                                }
                              }
                            }
                            n543 = property on="数组 8" class="Arr (严格)"("Value"=string[] [] ("数组 8")) -> ()  [unwired: 2 in, 2 out]
                          }
                          frame #1 {
                            n544 = property on="数组 8" class="Arr (严格)"("Value"=string[] ["温度", "水质", "极化曲线", "压力", "工步列表", "列表"]) -> ()  [unwired: 2 in, 2 out]
                          }
                          frame #2 {
                            n545 = property on="数组 3" class="Arr (严格)"() -> ("Value"=w800:refnum<vi>[])  [unwired: 2 in, 2 out]
                            n546 = for {
                              tunnel: w800 -> [w864] mode=indexing
                              n547 = property class="VI"(reference=w864) -> ("Name"=w863:string)  [unwired: 1 in, 2 out]
                              n548 = Search/Split String(string=w863, search string/char (-)=".") -> (substring before match=w861:string)  [unwired: 1 in, 2 out]
                              n549 = property on="数组 8" class="Arr (严格)"() -> ("Value"=w860:string[])  [unwired: 2 in, 2 out]
                              n550 = Search 1D Array(1D array=w860, element=w861) -> (index of element=w859:i32)  [unwired: 1 in]
                              n551 = Delete From Array(array=w860, index=w859) -> (array with subset deleted=w858:string[])  [unwired: 1 in, 1 out]
                              n552 = property on="数组 8" class="Arr (严格)"("Value"=w858) -> ()  [unwired: 2 in, 2 out]
                            }
                            n553 = stacked-sequence {
                              frame #0 {
                                n554 = flat-sequence {
                                frame #0 {
                                n555 = stacked-sequence {
                                frame #0 {
                                n556 = property on="分隔栏 4" class="Splitter"() -> ("Position"=w801:i32)  [unwired: 2 in, 2 out]
                                n557 = Add(x=w801, y=32 ("分隔栏位置")) -> (x+y=w803:i32)
                                n558 = property on="分隔栏 5" class="Splitter"("Position"=w803) -> ()  [unwired: 2 in, 2 out]
                                }
                                frame #1 {
                                n559 = property on="分隔栏 4" class="Splitter"() -> ("Position"=w806:i32)  [unwired: 2 in, 2 out]
                                n560 = Add(x=w806, y=62 ("分隔栏位置")) -> (x+y=w805:i32)
                                n561 = property on="分隔栏 6" class="Splitter"("Position"=w805) -> ()  [unwired: 2 in, 2 out]
                                }
                                frame #2 {
                                n562 = property on="分隔栏 4" class="Splitter"() -> ("Position"=w809:i32)  [unwired: 2 in, 2 out]
                                n563 = Add(x=w809, y=92 ("分隔栏位置")) -> (x+y=w808:i32)
                                n564 = property on="分隔栏 7" class="Splitter"("Position"=w808) -> ()  [unwired: 2 in, 2 out]
                                }
                                frame #3 {
                                n565 = property on="分隔栏 4" class="Splitter"() -> ("Position"=w812:i32)  [unwired: 2 in, 2 out]
                                n566 = Add(x=w812, y=122 ("分隔栏位置")) -> (x+y=w810:i32)
                                n567 = property on="分隔栏 8" class="Splitter"("Position"=w810) -> ()  [unwired: 2 in, 2 out]
                                }
                                }
                                }
                                frame #1 {
                                n568 = property on="1" class="Bool (严格)"("Value"=FALSE ("1")) -> ()  [unwired: 2 in, 2 out]
                                n569 = property on="2" class="Bool (严格)"("Value"=FALSE ("2")) -> ()  [unwired: 2 in, 2 out]
                                n570 = property on="3" class="Bool (严格)"("Value"=FALSE ("3")) -> ()  [unwired: 2 in, 2 out]
                                n571 = property on="4" class="Bool (严格)"("Value"=FALSE ("4")) -> ()  [unwired: 2 in, 2 out]
                                }
                                frame #2 {
                                n572 = control-ref of="窗格 8"() -> (w821:refnum<vi>)
                                n573 = control-ref of="窗格 7"() -> (w822:refnum<vi>)
                                n574 = control-ref of="窗格 6"() -> (w823:refnum<vi>)
                                n575 = control-ref of="窗格 9"() -> (w824:refnum<vi>)
                                n576 = property class="Pane"(reference=w821, "VertScrollbarVisibility"=T3."Always Off" ("垂直滚动条可见")) -> ()  [unwired: 1 in, 2 out]
                                n577 = property class="Pane"(reference=w822, "VertScrollbarVisibility"=T3."Always Off" ("垂直滚动条可见")) -> ()  [unwired: 1 in, 2 out]
                                n578 = property class="Pane"(reference=w823, "VertScrollbarVisibility"=T3."Always Off" ("垂直滚动条可见")) -> ()  [unwired: 1 in, 2 out]
                                n579 = property class="Pane"(reference=w824, "VertScrollbarVisibility"=T3."Always Off" ("垂直滚动条可见")) -> ()  [unwired: 1 in, 2 out]
                                }
                                }
                              }
                              frame #1 {
                                n580 = property on="分隔栏 2" class="Splitter"() -> ("Position"=w828:i32)  [unwired: 2 in, 2 out]
                                n581 = Equal?(x=w828, y=113) -> (x = y?=w827:bool)
                                n582 = case shown="假" w827 {
                                frame False {
                                n583 = while {
                                i -> [w853]
                                stop <- w846 stop-if-true
                                n584 = Multiply(x=10, y=w853) -> (x*y=w850:i32)
                                n585 = Subtract(x=448, y=w850) -> (x-y=w847:i32)
                                n586 = Less?(x=w847, y=163) -> (x < y?=w848:bool)
                                n587 = case shown="假" w848 {
                                tunnel: w847 -> [w854 _]
                                tunnel: [FALSE TRUE] -> w846
                                frame False {
                                n588 = property on="分隔栏 2" class="Splitter"("Position"=w854) -> ()  [unwired: 2 in, 2 out]
                                }
                                frame True {
                                n589 = property on="分隔栏 2" class="Splitter"("Position"=113 ("分隔栏位置")) -> ()  [unwired: 2 in, 2 out]
                                }
                                }
                                }
                                }
                                frame True {
                                }
                                }
                                n590 = property on="分隔栏 3" class="Splitter"() -> ("Position"=w829:i32)  [unwired: 2 in, 2 out]
                                n591 = Equal?(x=w829, y=116) -> (x = y?=w830:bool)
                                n592 = case shown="假" w830 {
                                frame False {
                                n593 = property on="分隔栏 3" class="Splitter"() -> ("Position"=w832:i32)  [unwired: 2 in, 2 out]
                                n594 = Greater?(x=w832, y=508) -> (0:w831:bool)
                                n595 = case shown="真" w831 {
                                frame False {
                                }
                                frame True {
                                n596 = while {
                                i -> [w841]
                                stop <- w834 stop-if-true
                                n597 = Multiply(x=10, y=w841) -> (x*y=w838:i32)
                                n598 = Subtract(x=509, y=w838) -> (x-y=w835:i32)
                                n599 = Less?(x=w835, y=166) -> (x < y?=w836:bool)
                                n600 = case shown="真" w836 {
                                tunnel: w835 -> [w842 _]
                                tunnel: [FALSE TRUE] -> w834
                                frame False {
                                n601 = property on="分隔栏 3" class="Splitter"("Position"=w842) -> ()  [unwired: 2 in, 2 out]
                                }
                                frame True {
                                n602 = property on="分隔栏 3" class="Splitter"("Position"=116 ("分隔栏位置")) -> ()  [unwired: 2 in, 2 out]
                                }
                                }
                                }
                                }
                                }
                                }
                                frame True {
                                }
                                }
                              }
                            }
                          }
                          frame #3 {
                            n603 = property on="数组 8" class="Arr (严格)"() -> ("Value"=w867:string[])  [unwired: 2 in, 2 out]
                            n604 = control-ref of="通道选择 2"() -> (w866:refnum<vi>)
                            n605 = register-events(w866) -> (reference out=w865:refnum<event-registration>)  [unwired: 2 in, 1 out]
                            n606 = for {
                              tunnel: w867 -> [w869] mode=indexing
                              tunnel: w865 -> [w868]
                              n607 = case shown="\"压力\"" w869 {
                                tunnel: w868 -> [w881 w903 w927 w964 _ w1000]
                                frame "温度", Default {
                                # "\\数据显示子程序\\温度.vi"
                                n608 = call <vilib>:"Application Directory.vi"() -> ("Application Directory"=w872:path)
                                n609 = Build Path(base path=w872, name or relative path="数据显示子程序\\温度.vi") -> (appended path=w870:path)
                                n610 = control-ref of="温度1"() -> (w886:refnum<vi>)
                                n611 = control-ref of="温度2"() -> (w887:refnum<vi>)
                                n612 = control-ref of="温度3"() -> (w888:refnum<vi>)
                                n613 = control-ref of="温度4"() -> (w889:refnum<vi>)
                                n614 = Bundle By Name(cluster=T8 {"温度1"=refnum, "温度2"=refnum, "温度3"=refnum, "温度4"=refnum}, "温度1"=w886, "温度2"=w887, "温度3"=w888, "温度4"=w889) -> (w885:T8)
                                n615 = Open VI Reference(type specifier VI Refnum (for type only)=refnum<vi> refnum ("类型说明符VI引用句柄（仅用于类型）"), vi path=w870, options=128 ("选项")) -> (vi reference=w891:refnum<vi>, error out=w890:errorcluster)  [unwired: 3 in]
                                n616 = control-ref of="字符串 4"() -> (w877:refnum<vi>)
                                n617 = control-ref of="字符串 7"() -> (w874:refnum<vi>)
                                n618 = control-ref of="字符串 6"() -> (w875:refnum<vi>)
                                n619 = control-ref of="字符串 5"() -> (w876:refnum<vi>)
                                n620 = control-ref of="新值"() -> (w878:refnum<vi>)
                                n621 = call-by-ref "开始异步调用"(reference=w891, error in=w890, "事件注册引用句柄 2"=w881, "簇"=w885, "Str引用句柄"=w877, "Str引用句柄 2"=w876, "Bool引用句柄 2"=w878, "Str引用句柄 3"=w875, "Str引用句柄 4"=w874) -> (reference out=w873:refnum<vi>)  [unwired: 13 in, 1 out]
                                n622 = property on="数组 3" class="Arr (严格)"() -> ("Value"=w879:refnum<vi>[])  [unwired: 2 in, 2 out]
                                n623 = Insert Into Array(array=w879, new element=w873) -> (w880:refnum<vi>[])  [unwired: 1 in]
                                n624 = property on="数组 3" class="Arr (严格)"("Value"=w880) -> ()  [unwired: 2 in, 2 out]
                                n625 = invoke on="子面板3" class="SubPnl" method="Insert VI"("VI Ref"=w873) -> ()  [unwired: 3 in, 4 out]
                                }
                                frame "水质" {
                                n626 = call <vilib>:"Application Directory.vi"() -> ("Application Directory"=w894:path)
                                n627 = Build Path(base path=w894, name or relative path="数据显示子程序\\水质.vi") -> (appended path=w892:path)
                                n628 = control-ref of="水质1"() -> (w909:refnum<vi>)
                                n629 = control-ref of="水质2"() -> (w910:refnum<vi>)
                                n630 = control-ref of="水质3"() -> (w911:refnum<vi>)
                                n631 = control-ref of="水质4"() -> (w912:refnum<vi>)
                                n632 = Bundle By Name(cluster=T9 {"水质1"=refnum, "水质2"=refnum, "水质3"=refnum, "水质4"=refnum}, "水质1"=w909, "水质2"=w910, "水质3"=w911, "水质4"=w912) -> (w908:T9)
                                n633 = control-ref of="字符串 7"() -> (w896:refnum<vi>)
                                n634 = control-ref of="字符串 6"() -> (w897:refnum<vi>)
                                n635 = control-ref of="字符串 5"() -> (w898:refnum<vi>)
                                n636 = Open VI Reference(type specifier VI Refnum (for type only)=refnum<vi> refnum ("类型说明符VI引用句柄（仅用于类型）"), vi path=w892, options=128 ("选项")) -> (vi reference=w907:refnum<vi>, error out=w913:errorcluster)  [unwired: 3 in]
                                n637 = control-ref of="字符串 4"() -> (w900:refnum<vi>)
                                n638 = control-ref of="新值"() -> (w899:refnum<vi>)
                                n639 = call-by-ref "开始异步调用"(reference=w907, error in=w913, "事件注册引用句柄"=w903, "簇"=w908, "Str引用句柄"=w900, "Str引用句柄 2"=w898, "Str引用句柄 4"=w896, "Str引用句柄 3"=w897, "Bool引用句柄 2"=w899) -> (reference out=w895:refnum<vi>)  [unwired: 13 in, 1 out]
                                n640 = property on="数组 3" class="Arr (严格)"() -> ("Value"=w901:refnum<vi>[])  [unwired: 2 in, 2 out]
                                n641 = Insert Into Array(array=w901, new element=w895) -> (w902:refnum<vi>[])  [unwired: 1 in]
                                n642 = property on="数组 3" class="Arr (严格)"("Value"=w902) -> ()  [unwired: 2 in, 2 out]
                                n643 = invoke on="子面板5" class="SubPnl" method="Insert VI"("VI Ref"=w895) -> ()  [unwired: 3 in, 4 out]
                                }
                                frame "极化曲线" {
                                n644 = control-ref of="电流4"() -> (w935:refnum<vi>)
                                n645 = control-ref of="电流3"() -> (w936:refnum<vi>)
                                n646 = control-ref of="电流2"() -> (w937:refnum<vi>)
                                n647 = control-ref of="电流1"() -> (w938:refnum<vi>)
                                n648 = Bundle By Name(cluster=T12 {"电流1"=refnum, "电流2"=refnum, "电流3"=refnum, "电流4"=refnum}, "电流1"=w938, "电流2"=w937, "电流3"=w936, "电流4"=w935) -> (w926:T12)
                                n649 = call <vilib>:"Application Directory.vi"() -> ("Application Directory"=w916:path)
                                n650 = control-ref of="电压3"() -> (w941:refnum<vi>)
                                n651 = control-ref of="电压4"() -> (w940:refnum<vi>)
                                n652 = control-ref of="电压1"() -> (w939:refnum<vi>)
                                n653 = control-ref of="电压2"() -> (w942:refnum<vi>)
                                n654 = Build Path(base path=w916, name or relative path="数据显示子程序\\极化曲线.vi") -> (appended path=w914:path)
                                n655 = Bundle By Name(cluster=T11 {"电压1"=refnum, "电压2"=refnum, "电压3"=refnum, "电压4"=refnum}, "电压1"=w939, "电压2"=w942, "电压3"=w941, "电压4"=w940) -> (w925:T11)
                                n656 = control-ref of="字符串 4"() -> (w923:refnum<vi>)
                                n657 = control-ref of="新值"() -> (w922:refnum<vi>)
                                n658 = Open VI Reference(type specifier VI Refnum (for type only)=refnum<vi> refnum ("类型说明符VI引用句柄（仅用于类型）"), vi path=w914, options=128 ("选项")) -> (vi reference=w928:refnum<vi>)  [unwired: 3 in, 1 out]
                                n659 = control-ref of="字符串 7"() -> (w918:refnum<vi>)
                                n660 = control-ref of="字符串 6"() -> (w919:refnum<vi>)
                                n661 = control-ref of="字符串 5"() -> (w920:refnum<vi>)
                                n662 = control-ref of="极化曲线3"() -> (w945:refnum<vi>)
                                n663 = control-ref of="极化曲线4"() -> (w946:refnum<vi>)
                                n664 = control-ref of="极化曲线1"() -> (w943:refnum<vi>)
                                n665 = control-ref of="极化曲线2"() -> (w944:refnum<vi>)
                                n666 = property on="数组 3" class="Arr (严格)"() -> ("Value"=w930:refnum<vi>[])  [unwired: 2 in, 2 out]
                                n667 = Bundle By Name(cluster=T10 {"极化曲线1"=refnum, "极化曲线2"=refnum, "极化曲线3"=refnum, "极化曲线4"=refnum}, "极化曲线1"=w943, "极化曲线2"=w944, "极化曲线3"=w945, "极化曲线4"=w946) -> (w924:T10)
                                n668 = call-by-ref "开始异步调用"(reference=w928, "事件注册引用句柄 2"=w927, "输出簇"=w926, "Str引用句柄"=w923, "Bool引用句柄 2"=w922, "输出簇 2"=w925, "输出簇 3"=w924, "Str引用句柄 2"=w920, "Str引用句柄 3"=w919, "Str引用句柄 4"=w918) -> (reference out=w917:refnum<vi>)  [unwired: 12 in, 1 out]
                                n669 = Insert Into Array(array=w930, new element=w917) -> (w931:refnum<vi>[])  [unwired: 1 in]
                                n670 = property on="数组 3" class="Arr (严格)"("Value"=w931) -> ()  [unwired: 2 in, 2 out]
                                n671 = invoke on="子面板2" class="SubPnl" method="Insert VI"("VI Ref"=w917) -> ()  [unwired: 3 in, 4 out]
                                }
                                frame "压力" {
                                n672 = call <vilib>:"Application Directory.vi"() -> ("Application Directory"=w948:path)
                                n673 = Build Path(base path=w948, name or relative path="数据显示子程序\\压力.vi") -> (appended path=w947:path)
                                n674 = control-ref of="压力1"() -> (w960:refnum<vi>)
                                n675 = control-ref of="压力2"() -> (w959:refnum<vi>)
                                n676 = control-ref of="压力3"() -> (w958:refnum<vi>)
                                n677 = control-ref of="压力4"() -> (w957:refnum<vi>)
                                n678 = Bundle By Name(cluster=T13 {"压力1"=refnum, "压力2"=refnum, "压力3"=refnum, "压力4"=refnum}, "压力1"=w960, "压力2"=w959, "压力3"=w958, "压力4"=w957) -> (w956:T13)
                                n679 = control-ref of="字符串 4"() -> (w955:refnum<vi>)
                                n680 = Open VI Reference(type specifier VI Refnum (for type only)=refnum<vi> refnum ("类型说明符VI引用句柄（仅用于类型）"), vi path=w947, options=128 ("选项")) -> (vi reference=w967:refnum<vi>, error out=w968:errorcluster)  [unwired: 3 in]
                                n681 = control-ref of="字符串 7"() -> (w951:refnum<vi>)
                                n682 = control-ref of="字符串 6"() -> (w952:refnum<vi>)
                                n683 = control-ref of="字符串 5"() -> (w953:refnum<vi>)
                                n684 = control-ref of="新值"() -> (w954:refnum<vi>)
                                n685 = call-by-ref "开始异步调用"(reference=w967, error in=w968, "事件注册引用句柄 2"=w964, "簇"=w956, "Str引用句柄"=w955, "Str引用句柄 2"=w953, "Str引用句柄 4"=w951, "Str引用句柄 3"=w952, "Bool引用句柄 2"=w954) -> (reference out=w950:refnum<vi>)  [unwired: 13 in, 1 out]
                                n686 = property on="数组 3" class="Arr (严格)"() -> ("Value"=w962:refnum<vi>[])  [unwired: 2 in, 2 out]
                                n687 = Insert Into Array(array=w962, new element=w950) -> (w963:refnum<vi>[])  [unwired: 1 in]
                                n688 = property on="数组 3" class="Arr (严格)"("Value"=w963) -> ()  [unwired: 2 in, 2 out]
                                n689 = invoke on="子面板4" class="SubPnl" method="Insert VI"("VI Ref"=w950) -> ()  [unwired: 3 in, 4 out]
                                }
                                frame "工步列表" {
                                # "数值 3"
                                n690 = property on="数组" class="Arr (严格)"() -> ("Value"=w976:string[][])  [unwired: 2 in, 2 out]
                                n691 = property on="数组 10" class="Arr (严格)"() -> ("Value"=w975:string[][])  [unwired: 2 in, 2 out]
                                n692 = property on="数组 12" class="Arr (严格)"() -> ("Value"=w973:string[][])  [unwired: 2 in, 2 out]
                                n693 = property on="数组 11" class="Arr (严格)"() -> ("Value"=w974:string[][])  [unwired: 2 in, 2 out]
                                n694 = control-ref of="数值"() -> (w987:refnum<vi>)
                                n695 = control-ref of="数值 2"() -> (w986:refnum<vi>)
                                n696 = control-ref of="数值 4"() -> (w984:refnum<vi>)
                                n697 = control-ref of="数值 3"() -> (w985:refnum<vi>)
                                n698 = call <vilib>:"Application Directory.vi"() -> ("Application Directory"=w971:path)
                                n699 = Build Array(w987, w986, w985, w984) -> (w983:refnum<vi>[])
                                n700 = Build Path(base path=w971, name or relative path="数据显示子程序\\工步列表.vi") -> (appended path=w969:path)
                                n701 = register-events(w983) -> (reference out=w981:refnum<event-registration>)  [unwired: 2 in, 1 out]
                                n702 = Build Array(w976, w975, w974, w973) -> (w982:string[][][])
                                n703 = Open VI Reference(type specifier VI Refnum (for type only)=refnum<vi> refnum ("类型说明符VI引用句柄（仅用于类型）"), vi path=w969, options=128 ("选项")) -> (vi reference=w989:refnum<vi>, error out=w988:errorcluster)  [unwired: 3 in]
                                n704 = call-by-ref "开始异步调用"(reference=w989, error in=w988, "事件注册引用句柄 3"=w981, "添加的数组 2"=w983, "添加的数组"=w982) -> (reference out=w972:refnum<vi>)  [unwired: 9 in, 1 out]
                                n705 = property on="数组 3" class="Arr (严格)"() -> ("Value"=w977:refnum<vi>[])  [unwired: 2 in, 2 out]
                                n706 = Insert Into Array(array=w977, new element=w972) -> (w978:refnum<vi>[])  [unwired: 1 in]
                                n707 = invoke on="子面板1" class="SubPnl" method="Insert VI"("VI Ref"=w972) -> ()  [unwired: 3 in, 4 out]
                                n708 = property on="数组 3" class="Arr (严格)"("Value"=w978) -> ()  [unwired: 2 in, 2 out]
                                }
                                frame "列表" {
                                n709 = call <vilib>:"Application Directory.vi"() -> ("Application Directory"=w992:path)
                                n710 = Build Path(base path=w992, name or relative path="数据显示子程序\\列表.vi") -> (appended path=w990:path)
                                n711 = Open VI Reference(type specifier VI Refnum (for type only)=refnum<vi> refnum ("类型说明符VI引用句柄（仅用于类型）"), vi path=w990, options=128 ("选项")) -> (vi reference=w1006:refnum<vi>, error out=w1005:errorcluster)  [unwired: 3 in]
                                n712 = control-ref of="所有数据4"() -> (w995:refnum<vi>)
                                n713 = control-ref of="所有数据3"() -> (w996:refnum<vi>)
                                n714 = control-ref of="所有数据2"() -> (w997:refnum<vi>)
                                n715 = control-ref of="所有数据"() -> (w998:refnum<vi>)
                                n716 = Bundle By Name(cluster=T14 {"所有数据"=refnum, "所有数据2"=refnum, "所有数据3"=refnum, "所有数据4"=refnum}, "所有数据"=w998, "所有数据2"=w997, "所有数据3"=w996, "所有数据4"=w995) -> (w994:T14)
                                n717 = call-by-ref "开始异步调用"(reference=w1006, error in=w1005, "簇"=w994, "事件注册引用句柄 2"=w1000) -> (reference out=w993:refnum<vi>)  [unwired: 10 in, 1 out]
                                n718 = property on="数组 3" class="Arr (严格)"() -> ("Value"=w1001:refnum<vi>[])  [unwired: 2 in, 2 out]
                                n719 = Insert Into Array(array=w1001, new element=w993) -> (w1002:refnum<vi>[])  [unwired: 1 in]
                                n720 = property on="数组 3" class="Arr (严格)"("Value"=w1002) -> ()  [unwired: 2 in, 2 out]
                                n721 = invoke on="子面板" class="SubPnl" method="Insert VI"("VI Ref"=w993) -> ()  [unwired: 3 in, 4 out]
                                }
                              }
                            }
                          }
                        }
                      }
                      frame #1 {
                        n722 = disable-structure shown="禁用" {
                          frame Disabled {
                            n723 = property on="数组 3" class="Arr (严格)"() -> ("Value"=w1007:refnum<vi>[])  [unwired: 2 in, 2 out]
                            n724 = for {
                              tunnel: w1007 -> [w1008] mode=indexing
                              n725 = property class="VI"(reference=w1008) -> ("Front Panel.Title"=w1019:string)  [unwired: 1 in, 2 out]
                              n726 = Wait (ms)(milliseconds to wait=u32 100 ("等待时间（毫秒）")) -> ()  [unwired: 1 out]
                              n727 = Compound Arithmetic op=OR ("复合运算")(1, 2 ("y"), 64 ("值")) -> (w1020:i32)
                              n728 = dll-call lib="PTH2Dabs CUsers526computerDesktop测试软件pemLABVIEW.dll" fn="findlabview"("lpcallsname"=0, "winname"=w1019, "layer"=-1, "x"=0, "y"=0, "cx"=0, "cy"=0, "flag"=w1020) -> ()  [unwired: 12 in, 2 out]
                            }
                          }
                          frame Enabled {
                          }
                        }
                      }
                    }
                  }
                  frame "耐久性曲线" {
                    n729 = flat-sequence {
                      frame #0 {
                        n730 = property on="数组 8" class="Arr (严格)"("Value"=string[] [] ("数组 8")) -> ()  [unwired: 2 in, 2 out]
                      }
                      frame #1 {
                        n731 = property on="数组 8" class="Arr (严格)"("Value"=string[] ["温度", "水质", "耐久性测试", "压力", "列表"]) -> ()  [unwired: 2 in, 2 out]
                      }
                      frame #2 {
                        n732 = property on="数组 3" class="Arr (严格)"() -> ("Value"=w1023:refnum<vi>[])  [unwired: 2 in, 2 out]
                        n733 = for {
                          tunnel: w1023 -> [w1030] mode=indexing
                          n734 = property class="VI"(reference=w1030) -> ("Name"=w1029:string)  [unwired: 1 in, 2 out]
                          n735 = Search/Split String(string=w1029, search string/char (-)=".") -> (substring before match=w1027:string)  [unwired: 1 in, 2 out]
                          n736 = property on="数组 8" class="Arr (严格)"() -> ("Value"=w1026:string[])  [unwired: 2 in, 2 out]
                          n737 = Search 1D Array(1D array=w1026, element=w1027) -> (index of element=w1025:i32)  [unwired: 1 in]
                          n738 = Delete From Array(array=w1026, index=w1025) -> (array with subset deleted=w1024:string[])  [unwired: 1 in, 1 out]
                          n739 = property on="数组 8" class="Arr (严格)"("Value"=w1024) -> ()  [unwired: 2 in, 2 out]
                        }
                      }
                      frame #3 {
                        n740 = stacked-sequence {
                          frame #0 {
                            n741 = flat-sequence {
                              frame #0 {
                                n742 = stacked-sequence {
                                frame #0 {
                                n743 = property on="分隔栏 4" class="Splitter"() -> ("Position"=w1031:i32)  [unwired: 2 in, 2 out]
                                n744 = Add(x=w1031, y=32 ("分隔栏位置")) -> (x+y=w1033:i32)
                                n745 = property on="分隔栏 5" class="Splitter"("Position"=w1033) -> ()  [unwired: 2 in, 2 out]
                                }
                                frame #1 {
                                n746 = property on="分隔栏 4" class="Splitter"() -> ("Position"=w1036:i32)  [unwired: 2 in, 2 out]
                                n747 = Add(x=w1036, y=62 ("分隔栏位置")) -> (x+y=w1035:i32)
                                n748 = property on="分隔栏 6" class="Splitter"("Position"=w1035) -> ()  [unwired: 2 in, 2 out]
                                }
                                frame #2 {
                                n749 = property on="分隔栏 4" class="Splitter"() -> ("Position"=w1039:i32)  [unwired: 2 in, 2 out]
                                n750 = Add(x=w1039, y=92 ("分隔栏位置")) -> (x+y=w1038:i32)
                                n751 = property on="分隔栏 7" class="Splitter"("Position"=w1038) -> ()  [unwired: 2 in, 2 out]
                                }
                                frame #3 {
                                n752 = property on="分隔栏 4" class="Splitter"() -> ("Position"=w1042:i32)  [unwired: 2 in, 2 out]
                                n753 = Add(x=w1042, y=122 ("分隔栏位置")) -> (x+y=w1040:i32)
                                n754 = property on="分隔栏 8" class="Splitter"("Position"=w1040) -> ()  [unwired: 2 in, 2 out]
                                }
                                }
                              }
                              frame #1 {
                                n755 = property on="1" class="Bool (严格)"("Value"=FALSE ("1")) -> ()  [unwired: 2 in, 2 out]
                                n756 = property on="2" class="Bool (严格)"("Value"=FALSE ("2")) -> ()  [unwired: 2 in, 2 out]
                                n757 = property on="3" class="Bool (严格)"("Value"=FALSE ("3")) -> ()  [unwired: 2 in, 2 out]
                                n758 = property on="4" class="Bool (严格)"("Value"=FALSE ("4")) -> ()  [unwired: 2 in, 2 out]
                              }
                              frame #2 {
                                n759 = control-ref of="窗格 8"() -> (w1051:refnum<vi>)
                                n760 = control-ref of="窗格 7"() -> (w1052:refnum<vi>)
                                n761 = control-ref of="窗格 6"() -> (w1053:refnum<vi>)
                                n762 = control-ref of="窗格 9"() -> (w1054:refnum<vi>)
                                n763 = property class="Pane"(reference=w1051, "VertScrollbarVisibility"=T3."Always Off" ("垂直滚动条可见")) -> ()  [unwired: 1 in, 2 out]
                                n764 = property class="Pane"(reference=w1052, "VertScrollbarVisibility"=T3."Always Off" ("垂直滚动条可见")) -> ()  [unwired: 1 in, 2 out]
                                n765 = property class="Pane"(reference=w1053, "VertScrollbarVisibility"=T3."Always Off" ("垂直滚动条可见")) -> ()  [unwired: 1 in, 2 out]
                                n766 = property class="Pane"(reference=w1054, "VertScrollbarVisibility"=T3."Always Off" ("垂直滚动条可见")) -> ()  [unwired: 1 in, 2 out]
                              }
                            }
                          }
                          frame #1 {
                            n767 = property on="分隔栏 2" class="Splitter"() -> ("Position"=w1058:i32)  [unwired: 2 in, 2 out]
                            n768 = Equal?(x=w1058, y=113) -> (x = y?=w1057:bool)
                            n769 = case shown="假" w1057 {
                              frame False {
                                n770 = while {
                                i -> [w1083]
                                stop <- w1076 stop-if-true
                                n771 = Multiply(x=10, y=w1083) -> (x*y=w1080:i32)
                                n772 = Subtract(x=448, y=w1080) -> (x-y=w1077:i32)
                                n773 = Less?(x=w1077, y=163) -> (x < y?=w1078:bool)
                                n774 = case shown="假" w1078 {
                                tunnel: w1077 -> [w1084 _]
                                tunnel: [FALSE TRUE] -> w1076
                                frame False {
                                n775 = property on="分隔栏 2" class="Splitter"("Position"=w1084) -> ()  [unwired: 2 in, 2 out]
                                }
                                frame True {
                                n776 = property on="分隔栏 2" class="Splitter"("Position"=113 ("分隔栏位置")) -> ()  [unwired: 2 in, 2 out]
                                }
                                }
                                }
                              }
                              frame True {
                              }
                            }
                            n777 = property on="分隔栏 3" class="Splitter"() -> ("Position"=w1059:i32)  [unwired: 2 in, 2 out]
                            n778 = Equal?(x=w1059, y=116) -> (x = y?=w1060:bool)
                            n779 = case shown="假" w1060 {
                              frame False {
                                n780 = property on="分隔栏 3" class="Splitter"() -> ("Position"=w1062:i32)  [unwired: 2 in, 2 out]
                                n781 = Greater?(x=w1062, y=508) -> (0:w1061:bool)
                                n782 = case shown="真" w1061 {
                                frame False {
                                }
                                frame True {
                                n783 = while {
                                i -> [w1071]
                                stop <- w1064 stop-if-true
                                n784 = Multiply(x=10, y=w1071) -> (x*y=w1068:i32)
                                n785 = Subtract(x=509, y=w1068) -> (x-y=w1065:i32)
                                n786 = Less?(x=w1065, y=166) -> (x < y?=w1066:bool)
                                n787 = case shown="真" w1066 {
                                tunnel: w1065 -> [w1072 _]
                                tunnel: [FALSE TRUE] -> w1064
                                frame False {
                                n788 = property on="分隔栏 3" class="Splitter"("Position"=w1072) -> ()  [unwired: 2 in, 2 out]
                                }
                                frame True {
                                n789 = property on="分隔栏 3" class="Splitter"("Position"=116 ("分隔栏位置")) -> ()  [unwired: 2 in, 2 out]
                                }
                                }
                                }
                                }
                                }
                              }
                              frame True {
                              }
                            }
                          }
                        }
                      }
                      frame #4 {
                        n790 = property on="数组 8" class="Arr (严格)"() -> ("Value"=w1089:string[])  [unwired: 2 in, 2 out]
                        n791 = for {
                          tunnel: w1089 -> [w1091] mode=indexing
                          tunnel: refnum<event-registration> refnum ("事件注册引用句柄") -> [w1090]
                          n792 = case shown="\"耐久性测试\"" w1091 {
                            tunnel: w1090 -> [w1095 w1110 w1125 w1153 w1159]
                            frame "温度", Default {
                              n793 = control-ref of="温度1"() -> (w1101:refnum<vi>)
                              n794 = control-ref of="温度2"() -> (w1102:refnum<vi>)
                              n795 = control-ref of="温度3"() -> (w1103:refnum<vi>)
                              n796 = control-ref of="温度4"() -> (w1104:refnum<vi>)
                              n797 = Bundle By Name(cluster=T8 {"温度1"=refnum, "温度2"=refnum, "温度3"=refnum, "温度4"=refnum}, "温度1"=w1101, "温度2"=w1102, "温度3"=w1103, "温度4"=w1104) -> (w1100:T8)
                              n798 = Open VI Reference(type specifier VI Refnum (for type only)=refnum<vi> refnum ("类型说明符VI引用句柄（仅用于类型）"), vi path=path "C:/Users/526computer/Desktop/数据显示子程序/温度.vi", options=128 ("选项")) -> (vi reference=w1106:refnum<vi>, error out=w1105:errorcluster)  [unwired: 3 in]
                              n799 = call-by-ref "开始异步调用"(reference=w1106, error in=w1105, "簇"=w1100, "事件注册引用句柄 2"=w1095) -> (reference out=w1092:refnum<vi>)  [unwired: 10 in, 1 out]
                              n800 = property on="数组 3" class="Arr (严格)"() -> ("Value"=w1093:refnum<vi>[])  [unwired: 2 in, 2 out]
                              n801 = Insert Into Array(array=w1093, new element=w1092) -> (w1094:refnum<vi>[])  [unwired: 1 in]
                              n802 = property on="数组 3" class="Arr (严格)"("Value"=w1094) -> ()  [unwired: 2 in, 2 out]
                            }
                            frame "水质" {
                              n803 = control-ref of="水质1"() -> (w1117:refnum<vi>)
                              n804 = control-ref of="水质2"() -> (w1118:refnum<vi>)
                              n805 = control-ref of="水质3"() -> (w1119:refnum<vi>)
                              n806 = control-ref of="水质4"() -> (w1120:refnum<vi>)
                              n807 = Bundle By Name(cluster=T9 {"水质1"=refnum, "水质2"=refnum, "水质3"=refnum, "水质4"=refnum}, "水质1"=w1117, "水质2"=w1118, "水质3"=w1119, "水质4"=w1120) -> (w1116:T9)
                              n808 = Open VI Reference(type specifier VI Refnum (for type only)=refnum<vi> refnum ("类型说明符VI引用句柄（仅用于类型）"), vi path=path "C:/Users/526computer/Desktop/数据显示子程序/水质.vi", options=128 ("选项")) -> (vi reference=w1115:refnum<vi>, error out=w1121:errorcluster)  [unwired: 3 in]
                              n809 = call-by-ref "开始异步调用"(reference=w1115, error in=w1121, "簇"=w1116, "事件注册引用句柄"=w1110) -> (reference out=w1107:refnum<vi>)  [unwired: 10 in, 1 out]
                              n810 = property on="数组 3" class="Arr (严格)"() -> ("Value"=w1108:refnum<vi>[])  [unwired: 2 in, 2 out]
                              n811 = Insert Into Array(array=w1108, new element=w1107) -> (w1109:refnum<vi>[])  [unwired: 1 in]
                              n812 = property on="数组 3" class="Arr (严格)"("Value"=w1109) -> ()  [unwired: 2 in, 2 out]
                            }
                            frame "耐久性测试" {
                              n813 = control-ref of="电流1"() -> (w1136:refnum<vi>)
                              n814 = control-ref of="电流2"() -> (w1135:refnum<vi>)
                              n815 = control-ref of="电流3"() -> (w1134:refnum<vi>)
                              n816 = control-ref of="电流4"() -> (w1133:refnum<vi>)
                              n817 = control-ref of="电压1"() -> (w1137:refnum<vi>)
                              n818 = control-ref of="电压2"() -> (w1140:refnum<vi>)
                              n819 = control-ref of="电压3"() -> (w1139:refnum<vi>)
                              n820 = control-ref of="电压4"() -> (w1138:refnum<vi>)
                              n821 = Bundle By Name(cluster=T12 {"电流1"=refnum, "电流2"=refnum, "电流3"=refnum, "电流4"=refnum}, "电流1"=w1136, "电流2"=w1135, "电流3"=w1134, "电流4"=w1133) -> (w1132:T12)
                              n822 = Bundle By Name(cluster=T11 {"电压1"=refnum, "电压2"=refnum, "电压3"=refnum, "电压4"=refnum}, "电压1"=w1137, "电压2"=w1140, "电压3"=w1139, "电压4"=w1138) -> (w1131:T11)
                              n823 = Open VI Reference(type specifier VI Refnum (for type only)=refnum<vi> refnum ("类型说明符VI引用句柄（仅用于类型）"), vi path=path "C:/Users/526computer/Desktop/数据显示子程序/耐久性测试.vi" ("VI路径"), options=128 ("选项")) -> (vi reference=w1141:refnum<vi>)  [unwired: 3 in, 1 out]
                              n824 = call-by-ref "开始异步调用"(reference=w1141, "输出簇 2"=w1131, "输出簇"=w1132, "事件注册引用句柄 2"=w1125) -> (reference out=w1122:refnum<vi>)  [unwired: 10 in, 1 out]
                              n825 = property on="数组 3" class="Arr (严格)"() -> ("Value"=w1123:refnum<vi>[])  [unwired: 2 in, 2 out]
                              n826 = Insert Into Array(array=w1123, new element=w1122) -> (w1124:refnum<vi>[])  [unwired: 1 in]
                              n827 = property on="数组 3" class="Arr (严格)"("Value"=w1124) -> ()  [unwired: 2 in, 2 out]
                            }
                            frame "压力" {
                              n828 = control-ref of="压力1"() -> (w1148:refnum<vi>)
                              n829 = control-ref of="压力2"() -> (w1147:refnum<vi>)
                              n830 = control-ref of="压力3"() -> (w1146:refnum<vi>)
                              n831 = control-ref of="压力4"() -> (w1145:refnum<vi>)
                              n832 = Bundle By Name(cluster=T13 {"压力1"=refnum, "压力2"=refnum, "压力3"=refnum, "压力4"=refnum}, "压力1"=w1148, "压力2"=w1147, "压力3"=w1146, "压力4"=w1145) -> (w1144:T13)
                              n833 = property on="字符串 4" class="Str"() -> ("Value"=w1143:string)  [unwired: 2 in, 2 out]
                              n834 = Open VI Reference(type specifier VI Refnum (for type only)=refnum<vi> refnum ("类型说明符VI引用句柄（仅用于类型）"), vi path=path "C:/Users/526computer/Desktop/数据显示子程序/压力.vi", options=128 ("选项")) -> (vi reference=w1157:refnum<vi>, error out=w1158:errorcluster)  [unwired: 3 in]
                              n835 = property on="新值" class="Bool (严格)"() -> ("Value"=w1142:bool)  [unwired: 2 in, 2 out]
                              n836 = call-by-ref "开始异步调用"(reference=w1157, error in=w1158, "确定按钮"=w1142, "字符串"=w1143, "簇"=w1144, "事件注册引用句柄 2"=w1153) -> (reference out=w1150:refnum<vi>)  [unwired: 8 in, 1 out]
                              n837 = property on="数组 3" class="Arr (严格)"() -> ("Value"=w1151:refnum<vi>[])  [unwired: 2 in, 2 out]
                              n838 = Insert Into Array(array=w1151, new element=w1150) -> (w1152:refnum<vi>[])  [unwired: 1 in]
                              n839 = property on="数组 3" class="Arr (严格)"("Value"=w1152) -> ()  [unwired: 2 in, 2 out]
                            }
                            frame "列表" {
                              n840 = Open VI Reference(type specifier VI Refnum (for type only)=refnum<vi> refnum ("类型说明符VI引用句柄（仅用于类型）"), vi path=path "C:/Users/526computer/Desktop/数据显示子程序/列表.vi" ("VI路径"), options=128 ("选项")) -> (vi reference=w1173:refnum<vi>, error out=w1172:errorcluster)  [unwired: 3 in]
                              n841 = control-ref of="所有数据4"() -> (w1165:refnum<vi>)
                              n842 = control-ref of="所有数据3"() -> (w1166:refnum<vi>)
                              n843 = control-ref of="所有数据2"() -> (w1167:refnum<vi>)
                              n844 = control-ref of="所有数据"() -> (w1168:refnum<vi>)
                              n845 = Bundle By Name(cluster=T14 {"所有数据"=refnum, "所有数据2"=refnum, "所有数据3"=refnum, "所有数据4"=refnum}, "所有数据"=w1168, "所有数据2"=w1167, "所有数据3"=w1166, "所有数据4"=w1165) -> (w1164:T14)
                              n846 = call-by-ref "开始异步调用"(reference=w1173, error in=w1172, "簇"=w1164, "事件注册引用句柄 2"=w1159) -> (reference out=w1169:refnum<vi>)  [unwired: 10 in, 1 out]
                              n847 = property on="数组 3" class="Arr (严格)"() -> ("Value"=w1170:refnum<vi>[])  [unwired: 2 in, 2 out]
                              n848 = Insert Into Array(array=w1170, new element=w1169) -> (w1171:refnum<vi>[])  [unwired: 1 in]
                              n849 = property on="数组 3" class="Arr (严格)"("Value"=w1171) -> ()  [unwired: 2 in, 2 out]
                            }
                          }
                        }
                      }
                      frame #5 {
                        n850 = property on="数组 3" class="Arr (严格)"() -> ("Value"=w1174:refnum<vi>[])  [unwired: 2 in, 2 out]
                        n851 = for {
                          tunnel: w1174 -> [w1176] mode=indexing
                          n852 = property class="VI"(reference=w1176) -> ("Front Panel.Title"=w1175:string)  [unwired: 1 in, 2 out]
                          n853 = Wait (ms)(milliseconds to wait=u32 100 ("等待时间（毫秒）")) -> ()  [unwired: 1 out]
                          n854 = Compound Arithmetic op=OR ("复合运算")(1, 2 ("y"), 64 ("值")) -> (w1187:i32)
                          n855 = dll-call lib="PTH2Dabs CUsers526computerDesktop测试软件pemLABVIEW.dll" fn="findlabview"("lpcallsname"=0, "winname"=w1175, "layer"=-1, "x"=0, "y"=0, "cx"=0, "cy"=0, "flag"=w1187) -> ()  [unwired: 12 in, 2 out]
                        }
                      }
                    }
                  }
                  frame "线性扫描" {
                  }
                }
              }
            }
          }
          frame #2 {
          }
        }
      }
      event "XY图", "波形图", "波形图 2", "波形图 3": Mouse Down {
        n856 = event-data() -> ("CtlRef"=w1189:refnum<vi>)  [unwired: 1 in, 7 out]
        n857 = property class="WFGraph"(reference=w1189) -> ("Label.Text"=w1188:string)  [unwired: 1 in, 2 out]
        n858 = case shown="\"波形图\"" w1188 {
          frame "XY图", Default {
            n859 = property on="XY图" class="XYGraph (严格)"() -> ("ActPaletteTool"=w1192:i32)  [unwired: 2 in, 2 out]
            n860 = Equal?(x=w1192, y=0) -> (x = y?=w1191:bool)
            n861 = case shown="真" w1191 {
              frame False {
              }
              frame True {
                n862 = property on="极化坐标" class="Str"("Visible"=TRUE ("可见")) -> ()  [unwired: 2 in, 2 out]
                n863 = property on="XY图" class="XYGraph (严格)"("Cursor.Cursor Index"=0 ("游标.游标索引"), "Cursor.Visible"=TRUE ("游标.可见")) -> ()  [unwired: 2 in, 2 out]
              }
            }
          }
          frame "波形图" {
            n864 = property on="波形图" class="WFGraph (严格)"() -> ("ActPaletteTool"=w1197:i32)  [unwired: 2 in, 2 out]
            n865 = Equal?(x=w1197, y=0) -> (x = y?=w1196:bool)
            n866 = case shown="真" w1196 {
              frame False {
              }
              frame True {
                n867 = property on="温度坐标" class="Str"("Visible"=TRUE ("可见")) -> ()  [unwired: 2 in, 2 out]
                n868 = property on="波形图" class="WFGraph (严格)"("Cursor.Cursor Index"=0 ("游标.游标索引"), "Cursor.Visible"=TRUE ("游标.可见")) -> ()  [unwired: 2 in, 2 out]
              }
            }
          }
          frame "波形图 2" {
            n869 = property on="波形图 2" class="WFGraph (严格)"() -> ("ActPaletteTool"=w1203:i32)  [unwired: 2 in, 2 out]
            n870 = Equal?(x=w1203, y=0) -> (x = y?=w1204:bool)
            n871 = case shown="真" w1204 {
              frame False {
              }
              frame True {
                n872 = property on="压力坐标" class="Str"("Visible"=TRUE ("可见")) -> ()  [unwired: 2 in, 2 out]
                n873 = property on="波形图 2" class="WFGraph (严格)"("Cursor.Cursor Index"=0 ("游标.游标索引"), "Cursor.Visible"=TRUE ("游标.可见")) -> ()  [unwired: 2 in, 2 out]
              }
            }
          }
          frame "波形图 3" {
            n874 = property on="波形图 3" class="WFGraph (严格)"() -> ("ActPaletteTool"=w1208:i32)  [unwired: 2 in, 2 out]
            n875 = Equal?(x=w1208, y=0) -> (x = y?=w1210:bool)
            n876 = case shown="真" w1210 {
              frame False {
              }
              frame True {
                n877 = property on="水质坐标" class="Str"("Visible"=TRUE ("可见")) -> ()  [unwired: 2 in, 2 out]
                n878 = property on="波形图 3" class="WFGraph (严格)"("Cursor.Cursor Index"=0 ("游标.游标索引"), "Cursor.Visible"=TRUE ("游标.可见")) -> ()  [unwired: 2 in, 2 out]
              }
            }
          }
        }
      }
      event "XY图", "波形图", "波形图 2", "波形图 3": Mouse Up {
        n879 = event-data() -> ("CtlRef"=w1215:refnum<vi>)  [unwired: 1 in, 7 out]
        n880 = property class="WFGraph"(reference=w1215) -> ("Label.Text"=w1214:string)  [unwired: 1 in, 2 out]
        n881 = case shown="\"波形图\"" w1214 {
          frame "XY图", Default {
            n882 = property on="XY图" class="XYGraph (严格)"() -> ("ActPaletteTool"=w1218:i32)  [unwired: 2 in, 2 out]
            n883 = Equal?(x=w1218, y=0) -> (x = y?=w1216:bool)
            n884 = case shown="真" w1216 {
              frame False {
              }
              frame True {
                n885 = property on="极化坐标" class="Str"("Visible"=FALSE ("可见")) -> ()  [unwired: 2 in, 2 out]
                n886 = property on="XY图" class="XYGraph (严格)"("Cursor.Cursor Index"=0 ("游标.游标索引"), "Cursor.Visible"=FALSE ("游标.可见")) -> ()  [unwired: 2 in, 2 out]
              }
            }
          }
          frame "波形图" {
            n887 = property on="波形图" class="WFGraph (严格)"() -> ("ActPaletteTool"=w1223:i32)  [unwired: 2 in, 2 out]
            n888 = Equal?(x=w1223, y=0) -> (x = y?=w1224:bool)
            n889 = case shown="真" w1224 {
              frame False {
              }
              frame True {
                n890 = property on="温度坐标" class="Str"("Visible"=FALSE ("可见")) -> ()  [unwired: 2 in, 2 out]
                n891 = property on="波形图" class="WFGraph (严格)"("Cursor.Cursor Index"=0 ("游标.游标索引"), "Cursor.Visible"=FALSE ("游标.可见")) -> ()  [unwired: 2 in, 2 out]
              }
            }
          }
          frame "波形图 2" {
            n892 = property on="波形图 2" class="WFGraph (严格)"() -> ("ActPaletteTool"=w1229:i32)  [unwired: 2 in, 2 out]
            n893 = Equal?(x=w1229, y=0) -> (x = y?=w1230:bool)
            n894 = case shown="真" w1230 {
              frame False {
              }
              frame True {
                n895 = property on="压力坐标" class="Str"("Visible"=FALSE ("可见")) -> ()  [unwired: 2 in, 2 out]
                n896 = property on="波形图 2" class="WFGraph (严格)"("Cursor.Cursor Index"=0 ("游标.游标索引"), "Cursor.Visible"=FALSE ("游标.可见")) -> ()  [unwired: 2 in, 2 out]
              }
            }
          }
          frame "波形图 3" {
            n897 = property on="波形图 3" class="WFGraph (严格)"() -> ("ActPaletteTool"=w1234:i32)  [unwired: 2 in, 2 out]
            n898 = Equal?(x=w1234, y=0) -> (x = y?=w1236:bool)
            n899 = case shown="真" w1236 {
              frame False {
              }
              frame True {
                n900 = property on="水质坐标" class="Str"("Visible"=FALSE ("可见")) -> ()  [unwired: 2 in, 2 out]
                n901 = property on="波形图 3" class="WFGraph (严格)"("Cursor.Cursor Index"=0 ("游标.游标索引"), "Cursor.Visible"=FALSE ("游标.可见")) -> ()  [unwired: 2 in, 2 out]
              }
            }
          }
        }
      }
      event "XY图", "波形图", "波形图 2", "波形图 3": Mouse Move {
        n902 = event-data() -> ("CtlRef"=w1241:refnum<vi>, "Coords"=w1242:T22)  [unwired: 1 in, 3 out]
        n903 = property class="WFGraph"(reference=w1241) -> ("Label.Text"=w1240:string)  [unwired: 1 in, 2 out]
        n904 = case shown="\"波形图 2\"" w1240 {
          tunnel: w1242 -> [w1246 w1260 w1277 w1294]
          frame "XY图", Default {
            n905 = property on="XY图" class="XYGraph (严格)"() -> ("ActPaletteTool"=w1245:i32)  [unwired: 2 in, 2 out]
            n906 = Equal?(x=w1245, y=0) -> (x = y?=w1243:bool)
            n907 = case shown="真" w1243 {
              tunnel: w1246 -> [_ w1258]
              frame False {
              }
              frame True {
                n908 = Unbundle(w1258) -> ("Horizontal"=w1257:i32, "Vertical"=w1256:i32)
                n909 = Add(x=w1256, y=5) -> (x+y=w1252:i32)
                n910 = invoke on="XY图" class="XYGraph (严格)" method="Map Coords To XY"("Coords"=w1258) -> ("XY"=w1259:cluster{"X":dbl, "Y":dbl})  [unwired: 6 in, 6 out]
                n911 = Add(x=w1257, y=10) -> (x+y=w1253:i32)
                n912 = Bundle(w1253, w1252) -> (w1251:cluster{i32, i32})  [unwired: 1 in]
                n913 = property on="极化坐标" class="Str"("Position"=w1251) -> ()  [unwired: 2 in, 2 out]
                n914 = Unbundle(w1259) -> ("X"=w1250:dbl, "Y"=w1249:dbl)
                n915 = property on="XY图" class="XYGraph (严格)"("Cursor.Cursor X"=w1250, "Cursor.Cursor Y"=w1249) -> ()  [unwired: 2 in, 2 out]
                n916 = Format Into String(format string="X:%.3f,Y:%.3f" ("格式字符串"), w1250, w1249) -> (resulting string=w1247:string)  [unwired: 2 in, 1 out]
                n917 = property on="极化坐标" class="Str"("Value"=w1247) -> ()  [unwired: 2 in, 2 out]
              }
            }
          }
          frame "波形图" {
            n918 = property on="波形图" class="WFGraph (严格)"() -> ("ActPaletteTool"=w1262:i32)  [unwired: 2 in, 2 out]
            n919 = Equal?(x=w1262, y=0) -> (x = y?=w1263:bool)
            n920 = case shown="真" w1263 {
              tunnel: w1260 -> [_ w1264]
              frame False {
              }
              frame True {
                n921 = Unbundle(w1264) -> ("Horizontal"=w1271:i32, "Vertical"=w1272:i32)
                n922 = invoke on="波形图" class="WFGraph (严格)" method="Map Coords To XY"("Coords"=w1264) -> ("XY"=w1269:cluster{"X":dbl, "Y":dbl})  [unwired: 6 in, 6 out]
                n923 = Add(x=w1272, y=5) -> (x+y=w1276:i32)
                n924 = Add(x=w1271, y=10) -> (x+y=w1275:i32)
                n925 = Bundle(w1275, w1276) -> (w1270:cluster{i32, i32})  [unwired: 1 in]
                n926 = Unbundle(w1269) -> ("X"=w1268:dbl, "Y"=w1267:dbl)
                n927 = property on="温度坐标" class="Str"("Position"=w1270) -> ()  [unwired: 2 in, 2 out]
                n928 = Format Into String(format string="X:%.3f,Y:%.3f" ("格式字符串"), w1268, w1267) -> (resulting string=w1266:string)  [unwired: 2 in, 1 out]
                n929 = property on="波形图" class="WFGraph (严格)"("Cursor.Cursor X"=w1268, "Cursor.Cursor Y"=w1267) -> ()  [unwired: 2 in, 2 out]
                n930 = property on="温度坐标" class="Str"("Value"=w1266) -> ()  [unwired: 2 in, 2 out]
              }
            }
          }
          frame "波形图 2" {
            n931 = property on="波形图 2" class="WFGraph (严格)"() -> ("ActPaletteTool"=w1279:i32)  [unwired: 2 in, 2 out]
            n932 = Equal?(x=w1279, y=0) -> (x = y?=w1280:bool)
            n933 = case shown="真" w1280 {
              tunnel: w1277 -> [_ w1282]
              frame False {
              }
              frame True {
                n934 = Unbundle(w1282) -> ("Horizontal"=w1291:i32, "Vertical"=w1290:i32)
                n935 = invoke on="波形图 2" class="WFGraph (严格)" method="Map Coords To XY"("Coords"=w1282) -> ("XY"=w1285:cluster{"X":dbl, "Y":dbl})  [unwired: 6 in, 6 out]
                n936 = Add(x=w1290, y=5) -> (x+y=w1286:i32)
                n937 = Add(x=w1291, y=10) -> (x+y=w1287:i32)
                n938 = Bundle(w1287, w1286) -> (w1281:cluster{i32, i32})  [unwired: 1 in]
                n939 = Unbundle(w1285) -> ("X"=w1284:dbl, "Y"=w1283:dbl)
                n940 = Format Into String(format string="X:%.3f,Y:%.3f" ("格式字符串"), w1284, w1283) -> (resulting string=w1292:string)  [unwired: 2 in, 1 out]
                n941 = property on="压力坐标" class="Str"("Position"=w1281) -> ()  [unwired: 2 in, 2 out]
                n942 = property on="波形图 2" class="WFGraph (严格)"("Cursor.Cursor X"=w1284, "Cursor.Cursor Y"=w1283) -> ()  [unwired: 2 in, 2 out]
                n943 = property on="压力坐标" class="Str"("Value"=w1292) -> ()  [unwired: 2 in, 2 out]
              }
            }
          }
          frame "波形图 3" {
            n944 = property on="波形图 3" class="WFGraph (严格)"() -> ("ActPaletteTool"=w1297:i32)  [unwired: 2 in, 2 out]
            n945 = Equal?(x=w1297, y=0) -> (x = y?=w1296:bool)
            n946 = case shown="真" w1296 {
              tunnel: w1294 -> [_ w1299]
              frame False {
              }
              frame True {
                n947 = invoke on="波形图 3" class="WFGraph (严格)" method="Map Coords To XY"("Coords"=w1299) -> ("XY"=w1304:cluster{"X":dbl, "Y":dbl})  [unwired: 6 in, 6 out]
                n948 = Unbundle(w1299) -> ("Horizontal"=w1305:i32, "Vertical"=w1306:i32)
                n949 = Add(x=w1306, y=5) -> (x+y=w1310:i32)
                n950 = Add(x=w1305, y=10) -> (x+y=w1309:i32)
                n951 = Bundle(w1309, w1310) -> (w1298:cluster{i32, i32})  [unwired: 1 in]
                n952 = Unbundle(w1304) -> ("X"=w1303:dbl, "Y"=w1302:dbl)
                n953 = property on="水质坐标" class="Str"("Position"=w1298) -> ()  [unwired: 2 in, 2 out]
                n954 = Format Into String(format string="X:%.3f,Y:%.3f" ("格式字符串"), w1303, w1302) -> (resulting string=w1300:string)  [unwired: 2 in, 1 out]
                n955 = property on="波形图 3" class="WFGraph (严格)"("Cursor.Cursor X"=w1303, "Cursor.Cursor Y"=w1302) -> ()  [unwired: 2 in, 2 out]
                n956 = property on="水质坐标" class="Str"("Value"=w1300) -> ()  [unwired: 2 in, 2 out]
              }
            }
          }
        }
      }
      event "文本下拉列表 3", "文本下拉列表 4", "文本下拉列表 5", "文本下拉列表 6", "文本下拉列表 7": Value Change {
        n957 = event-data() -> ("CtlRef"=w1312:refnum<vi>)  [unwired: 1 in, 5 out]
        n958 = property class="Ring (严格)"(reference=w1312) -> ("Label.Text"=w1311:string)  [unwired: 1 in, 2 out]
        n959 = case shown="\"文本下拉列表 3,文本下拉列表 4\", 默认" w1311 {
          frame "文本下拉列表 3,文本下拉列表 4", Default {
            n960 = case shown="0, 默认" "文本下拉列表 3" {
              tunnel: [u32 4 ("活动曲线") u32 5 ("活动曲线")] -> w1313
              frame 0, Default {
              }
              frame 1 {
              }
            }
            n961 = case shown="1" "文本下拉列表 4" {
              tunnel: [u8 2 ("曲线.曲线插值") u32 0 ("活动曲线") u32 1 ("活动曲线") u32 3 ("活动曲线")] -> w1314
              frame 0, Default {
              }
              frame 1 {
              }
              frame 2 {
              }
              frame 3 {
              }
            }
            n962 = property on="XY图" class="XYGraph (严格)"("Active Plot"=w1313, "Plot.Plot Interpolation"=w1314) -> ()  [unwired: 2 in, 2 out]
          }
          frame "文本下拉列表 5" {
            n963 = case shown="1" "文本下拉列表 5" {
              tunnel: [u8 2 ("曲线.曲线插值") u32 0 ("活动曲线") u32 1 ("活动曲线") u32 3 ("活动曲线")] -> w1323
              frame 0, Default {
              }
              frame 1 {
              }
              frame 2 {
              }
              frame 3 {
              }
            }
            n964 = property on="波形图" class="WFGraph (严格)"("Active Plot"=u32 0 ("活动曲线"), "Plot.Plot Interpolation"=w1323) -> ()  [unwired: 2 in, 2 out]
          }
          frame "文本下拉列表 6" {
            n965 = case shown="1" "文本下拉列表 6" {
              tunnel: [u8 2 ("曲线.曲线插值") u32 0 ("活动曲线") u32 1 ("活动曲线") u32 3 ("活动曲线")] -> w1330
              frame 0, Default {
              }
              frame 1 {
              }
              frame 2 {
              }
              frame 3 {
              }
            }
            n966 = property on="波形图 2" class="WFGraph (严格)"("Active Plot"=u32 0 ("活动曲线"), "Plot.Plot Interpolation"=w1330) -> ()  [unwired: 2 in, 2 out]
          }
          frame "文本下拉列表 7" {
            n967 = case shown="1" "文本下拉列表 7" {
              tunnel: [u8 2 ("曲线.曲线插值") u32 0 ("活动曲线") u32 1 ("活动曲线") u32 3 ("活动曲线")] -> w1337
              frame 0, Default {
              }
              frame 1 {
              }
              frame 2 {
              }
              frame 3 {
              }
            }
            n968 = property on="波形图 3" class="WFGraph (严格)"("Active Plot"=u32 0 ("活动曲线"), "Plot.Plot Interpolation"=w1337) -> ()  [unwired: 2 in, 2 out]
          }
        }
      }
      event "文本下拉列表 2", "文本下拉列表 8", "文本下拉列表 9", "文本下拉列表 10": Value Change {
        n969 = event-data() -> ("CtlRef"=w1345:refnum<vi>)  [unwired: 1 in, 5 out]
        n970 = property class="Ring (严格)"(reference=w1345) -> ("Label.Text"=w1344:string)  [unwired: 1 in, 2 out]
        n971 = case shown="\"文本下拉列表 10\"" w1344 {
          frame "文本下拉列表 2", Default {
            n972 = case shown="2" "文本下拉列表 2" {
              frame 0, Default {
                n973 = invoke on="XY图" class="XYGraph (严格)" method="Export Data to Excel"() -> ()  [unwired: 3 in, 3 out]
              }
              frame 1 {
                n974 = invoke on="XY图" class="XYGraph (严格)" method="Export Data to Clipboard"() -> ()  [unwired: 3 in, 3 out]
              }
              frame 2 {
                n975 = invoke on="XY图" class="XYGraph (严格)" method="Export Image"("FileType"=enum32{"BMP", "EPS", "EMF", "PICT"}."BMP" ("文件类型"), "Target"=enum32{"File", "Clipboard"}."File" ("目标"), "Path"=path "C:/Users/526computer/Desktop" ("路径"), "HideGrid"=FALSE ("隐藏网格")) -> ()  [unwired: 4 in, 8 out]
              }
            }
          }
          frame "文本下拉列表 8" {
            n976 = case shown="2" "文本下拉列表 8" {
              frame 0, Default {
                n977 = invoke on="波形图" class="WFGraph (严格)" method="Export Data to Excel"() -> ()  [unwired: 3 in, 3 out]
              }
              frame 1 {
                n978 = invoke on="波形图" class="WFGraph (严格)" method="Export Data to Clipboard"() -> ()  [unwired: 3 in, 3 out]
              }
              frame 2 {
                n979 = invoke on="波形图" class="WFGraph (严格)" method="Export Image"("FileType"=enum32{"BMP", "EPS", "EMF", "PICT"}."BMP" ("文件类型"), "Target"=enum32{"File", "Clipboard"}."File" ("目标"), "Path"=path "C:/Users/526computer/Desktop" ("路径"), "HideGrid"=FALSE ("隐藏网格"), "Overwrite"=FALSE ("始终覆盖")) -> ()  [unwired: 3 in, 8 out]
              }
            }
          }
          frame "文本下拉列表 9" {
            n980 = case shown="2" "文本下拉列表 9" {
              frame 0, Default {
                n981 = invoke on="波形图 2" class="WFGraph (严格)" method="Export Data to Excel"() -> ()  [unwired: 3 in, 3 out]
              }
              frame 1 {
                n982 = invoke on="波形图 2" class="WFGraph (严格)" method="Export Data to Clipboard"() -> ()  [unwired: 3 in, 3 out]
              }
              frame 2 {
                n983 = invoke on="波形图 2" class="WFGraph (严格)" method="Export Image"("FileType"=enum32{"BMP", "EPS", "EMF", "PICT"}."BMP" ("文件类型"), "Target"=enum32{"File", "Clipboard"}."File" ("目标"), "Path"=path "C:/Users/526computer/Desktop" ("路径"), "HideGrid"=FALSE ("隐藏网格"), "Overwrite"=FALSE ("始终覆盖")) -> ()  [unwired: 3 in, 8 out]
              }
            }
          }
          frame "文本下拉列表 10" {
            n984 = case shown="2" "文本下拉列表 10" {
              frame 0, Default {
                n985 = invoke on="波形图 3" class="WFGraph (严格)" method="Export Data to Excel"() -> ()  [unwired: 3 in, 3 out]
              }
              frame 1 {
                n986 = invoke on="波形图 3" class="WFGraph (严格)" method="Export Data to Clipboard"() -> ()  [unwired: 3 in, 3 out]
              }
              frame 2 {
                n987 = invoke on="波形图 3" class="WFGraph (严格)" method="Export Image"("FileType"=enum32{"BMP", "EPS", "EMF", "PICT"}."BMP" ("文件类型"), "Target"=enum32{"File", "Clipboard"}."File" ("目标"), "Path"=path "C:/Users/526computer/Desktop" ("路径"), "HideGrid"=FALSE ("隐藏网格"), "Overwrite"=FALSE ("始终覆盖")) -> ()  [unwired: 3 in, 8 out]
              }
            }
          }
        }
      }
      event "实时数据": Value Change {
        n988 = event-data() -> ()  [unwired: 1 in, 6 out]
        n989 = control-ref of="冷凝器液位 2"() -> (w1384:refnum<vi>)
        n990 = control-ref of="露点仪 2"() -> (w1383:refnum<vi>)
        n991 = control-ref of="微量氧 2"() -> (w1382:refnum<vi>)
        n992 = control-ref of="纯度仪 2"() -> (w1381:refnum<vi>)
        n993 = control-ref of="气分液位 2"() -> (w1380:refnum<vi>)
        n994 = control-ref of="电解电压 2"() -> (w1379:refnum<vi>)
        n995 = control-ref of="电解电流 2"() -> (w1378:refnum<vi>)
        n996 = control-ref of="水质电导率 2"() -> (w1377:refnum<vi>)
        n997 = control-ref of="循环水压 2"() -> (w1376:refnum<vi>)
        n998 = control-ref of="冷却水水压 2"() -> (w1375:refnum<vi>)
        n999 = control-ref of="氢渗 2"() -> (w1374:refnum<vi>)
        n1000 = control-ref of="氢中氧 2"() -> (w1373:refnum<vi>)
        n1001 = control-ref of="水箱温度 2"() -> (w1372:refnum<vi>)
        n1002 = control-ref of="水箱液位 2"() -> (w1371:refnum<vi>)
        n1003 = property on="选项卡控件 2" class="TabCtl (严格)"("Value"=T2."实时数据" ("选项卡控件 2")) -> ()  [unwired: 2 in, 2 out]
        n1004 = property on="new picture" class="Pict"("ZoomFactor"=sgl 0.92 ("缩放因子")) -> ()  [unwired: 2 in, 2 out]
        n1005 = Build Array(w1384, w1383, w1382, w1381, w1380, w1379, w1378, w1377, w1376, w1375, w1374, w1373, w1372, w1371) -> (w1370:refnum<vi>[])
        n1006 = property on="分隔栏 2" class="Splitter"() -> ("Position"=w1405:i32)  [unwired: 2 in, 2 out]
        n1007 = property on="分隔栏 3" class="Splitter"() -> ("Position"=w1401:i32)  [unwired: 2 in, 2 out]
        n1008 = Equal?(x=w1405, y=113) -> (x = y?=w1404:bool)
        n1009 = control-ref of="冷凝器液位"() -> (w1399:refnum<vi>)
        n1010 = control-ref of="露点仪"() -> (w1398:refnum<vi>)
        n1011 = control-ref of="微量氧"() -> (w1397:refnum<vi>)
        n1012 = control-ref of="纯度仪"() -> (w1396:refnum<vi>)
        n1013 = control-ref of="气分液位"() -> (w1395:refnum<vi>)
        n1014 = control-ref of="电解电压"() -> (w1394:refnum<vi>)
        n1015 = control-ref of="电解电流"() -> (w1393:refnum<vi>)
        n1016 = control-ref of="水质电导率"() -> (w1392:refnum<vi>)
        n1017 = control-ref of="循环水压"() -> (w1391:refnum<vi>)
        n1018 = control-ref of="冷却水水压"() -> (w1390:refnum<vi>)
        n1019 = control-ref of="氢渗"() -> (w1389:refnum<vi>)
        n1020 = control-ref of="氢中氧"() -> (w1388:refnum<vi>)
        n1021 = control-ref of="水箱温度"() -> (w1387:refnum<vi>)
        n1022 = control-ref of="水箱液位"() -> (w1386:refnum<vi>)
        n1023 = Equal?(x=w1401, y=116) -> (x = y?=w1402:bool)
        n1024 = case shown="假" w1404 {
          frame False {
            n1025 = while {
              i -> [w1418]
              stop <- w1411 stop-if-true
              n1026 = Multiply(x=50, y=w1418) -> (x*y=w1415:i32)
              n1027 = Subtract(x=448, y=w1415) -> (x-y=w1412:i32)
              n1028 = Less?(x=w1412, y=163) -> (x < y?=w1413:bool)
              n1029 = case shown="真" w1413 {
                tunnel: w1412 -> [w1419 _]
                tunnel: [FALSE TRUE] -> w1411
                frame False {
                  n1030 = property on="分隔栏 2" class="Splitter"("Position"=w1419) -> ()  [unwired: 2 in, 2 out]
                }
                frame True {
                  n1031 = property on="分隔栏 2" class="Splitter"("Position"=113 ("分隔栏位置")) -> ()  [unwired: 2 in, 2 out]
                }
              }
            }
          }
          frame True {
          }
        }
        n1032 = case shown="假" w1402 {
          frame False {
            n1033 = property on="分隔栏 3" class="Splitter"() -> ("Position"=w1424:i32)  [unwired: 2 in, 2 out]
            n1034 = Greater?(x=w1424, y=508) -> (0:w1423:bool)
            n1035 = case shown="真" w1423 {
              frame False {
              }
              frame True {
                n1036 = while {
                  i -> [w1433]
                  stop <- w1426 stop-if-true
                  n1037 = Multiply(x=50, y=w1433) -> (x*y=w1430:i32)
                  n1038 = Subtract(x=509, y=w1430) -> (x-y=w1427:i32)
                  n1039 = Less?(x=w1427, y=166) -> (x < y?=w1428:bool)
                  n1040 = case shown="假" w1428 {
                    tunnel: w1427 -> [w1434 _]
                    tunnel: [FALSE TRUE] -> w1426
                    frame False {
                      n1041 = property on="分隔栏 3" class="Splitter"("Position"=w1434) -> ()  [unwired: 2 in, 2 out]
                    }
                    frame True {
                      n1042 = property on="分隔栏 3" class="Splitter"("Position"=116 ("分隔栏位置")) -> ()  [unwired: 2 in, 2 out]
                    }
                  }
                }
              }
            }
          }
          frame True {
          }
        }
        n1043 = Build Array(w1399, w1398, w1397, w1396, w1395, w1394, w1393, w1392, w1391, w1390, w1389, w1388, w1387, w1386) -> (w1385:refnum<vi>[])
        n1044 = for {
          tunnel: w1385 -> [w1410] mode=indexing
          tunnel: w1370 -> [w1408] mode=indexing
          n1045 = property class="Str"(reference=w1408, "Visible"=FALSE ("可见")) -> ()  [unwired: 1 in, 2 out]
          n1046 = property class="Str"(reference=w1410, "Visible"=TRUE ("可见")) -> ()  [unwired: 1 in, 2 out]
        }
      }
      event "电流/电压", "温度", "压强", "工步", "水质 2": Value Change {
        n1047 = event-data() -> ("CtlRef"=w1439:refnum<vi>)  [unwired: 1 in, 5 out]
        n1048 = property class="Bool (严格)"(reference=w1439) -> ("Label.Text"=w1438:string)  [unwired: 1 in, 2 out]
        n1049 = case shown="\"电流/电压\", 默认" w1438 {
          frame "电流/电压", Default {
            n1050 = property on="选项卡控件 2" class="TabCtl (严格)"("Value"=T2."极化曲线" ("选项卡控件 2")) -> ()  [unwired: 2 in, 2 out]
            n1051 = flat-sequence {
              frame #0 {
                n1052 = invoke on="子面板2" class="SubPnl" method="Remove VI"() -> ()  [unwired: 3 in, 3 out]
              }
              frame #1 {
                n1053 = property on="数组 3" class="Arr (严格)"() -> ("Value"=w1441:refnum<vi>[])  [unwired: 2 in, 2 out]
                n1054 = for {
                  tunnel: w1441 -> [w1442] mode=indexing
                  n1055 = property class="VI"(reference=w1442) -> ("Name"=w1445:string)  [unwired: 1 in, 2 out]
                  n1056 = Equal?(x=w1445, y="极化曲线.vi") -> (x = y?=w1443:bool)
                  n1057 = case shown="真" w1443 {
                    tunnel: w1442 -> [_ w1446]
                    frame False {
                    }
                    frame True {
                      n1058 = property class="VI"(reference=w1446) -> ("Exec.State"=w1447:T23)  [unwired: 1 in, 2 out]
                      n1059 = case shown="\"Run top level\"" w1447 {
                        tunnel: w1446 -> [_ w1452 w1457 w1458]
                        frame "Bad", Default {
                          # "VI包含错误并且无法执行。"
                        }
                        frame "Idle" {
                          # "VI位于内存中但没有运行"
                          n1060 = invoke class="VI" method="Run VI"(reference=w1452, "Wait until done"=FALSE ("结束前等待"), "Auto Dispose Ref"=FALSE ("自动销毁引用")) -> (reference out=w1449:refnum<vi>, error out=w1448:errorcluster)  [unwired: 2 in, 3 out]
                          n1061 = invoke on="子面板6" class="SubPnl" method="Insert VI"(error in=w1448, "VI Ref"=w1449) -> ()  [unwired: 2 in, 4 out]
                        }
                        frame "Run top level" {
                          # "VI是活动层次结构中的顶层VI"
                          n1062 = property class="VI"(reference=w1457, "FP.State"=T15."Closed" ("前面板窗口:状态")) -> (reference out=w1454:refnum<vi>, error out=w1455:errorcluster)  [unwired: 1 in]
                          n1063 = call <vilib>:"Clear Errors.vi"("error in (no error)"=w1455) -> ("error out"=w1453:errorcluster)  [unwired: 5 in, 1 out]
                          n1064 = invoke on="子面板6" class="SubPnl" method="Insert VI"(error in=w1453, "VI Ref"=w1454) -> ()  [unwired: 2 in, 4 out]
                        }
                        frame "Running" {
                          # "VI已由一个或多个处于活动状态的顶层VI保留为执行"
                          n1065 = invoke on="子面板6" class="SubPnl" method="Insert VI"("VI Ref"=w1458) -> ()  [unwired: 3 in, 4 out]
                        }
                      }
                    }
                  }
                }
              }
              frame #2 {
                n1066 = property on="电流/电压" class="Bool (严格)"("Value"=FALSE ("电流/电压")) -> ()  [unwired: 2 in, 2 out]
              }
              frame #3 {
              }
            }
          }
        }
      }
      event "数据分析": Value Change {
        n1067 = event-data() -> ()  [unwired: 1 in, 6 out]
        n1068 = property on="分隔栏 3" class="Splitter"() -> ("Position"=w1464:i32)  [unwired: 2 in, 2 out]
        n1069 = Equal?(x=w1464, y=116) -> (x = y?=w1465:bool)
        n1070 = case shown="假" w1465 {
          frame False {
            n1071 = property on="分隔栏 3" class="Splitter"() -> ("Position"=w1582:i32)  [unwired: 2 in, 2 out]
            n1072 = Greater?(x=w1582, y=508) -> (0:w1581:bool)
            n1073 = case shown="真" w1581 {
              frame False {
              }
              frame True {
                n1074 = while {
                  i -> [w1591]
                  stop <- w1584 stop-if-true
                  n1075 = Multiply(x=50, y=w1591) -> (x*y=w1588:i32)
                  n1076 = Subtract(x=509, y=w1588) -> (x-y=w1585:i32)
                  n1077 = Less?(x=w1585, y=166) -> (x < y?=w1586:bool)
                  n1078 = case shown="假" w1586 {
                    tunnel: w1585 -> [w1592 _]
                    tunnel: [FALSE TRUE] -> w1584
                    frame False {
                      n1079 = property on="分隔栏 3" class="Splitter"("Position"=w1592) -> ()  [unwired: 2 in, 2 out]
                    }
                    frame True {
                      n1080 = property on="分隔栏 3" class="Splitter"("Position"=116 ("分隔栏位置")) -> ()  [unwired: 2 in, 2 out]
                    }
                  }
                }
              }
            }
          }
          frame True {
          }
        }
        n1081 = property on="选项卡控件 2" class="TabCtl (严格)"("Value"=T2."    设置界面" ("选项卡控件 2")) -> ()  [unwired: 2 in, 2 out]
        n1082 = property on="选项卡控件 4" class="TabCtl (严格)"("Value"=enum32{"极化曲线", "温度", "压力", "水质"}."极化曲线" ("选项卡控件 4")) -> ()  [unwired: 2 in, 2 out]
        n1083 = property on="分隔栏 2" class="Splitter"() -> ("Position"=w1467:i32)  [unwired: 2 in, 2 out]
        n1084 = Equal?(x=w1467, y=113) -> (x = y?=w1466:bool)
        n1085 = case shown="假" w1466 {
          frame False {
            n1086 = while {
              i -> [w1576]
              stop <- w1569 stop-if-true
              n1087 = Multiply(x=50, y=w1576) -> (x*y=w1573:i32)
              n1088 = Subtract(x=448, y=w1573) -> (x-y=w1570:i32)
              n1089 = Less?(x=w1570, y=163) -> (x < y?=w1571:bool)
              n1090 = case shown="真" w1571 {
                tunnel: w1570 -> [w1577 _]
                tunnel: [FALSE TRUE] -> w1569
                frame False {
                  n1091 = property on="分隔栏 2" class="Splitter"("Position"=w1577) -> ()  [unwired: 2 in, 2 out]
                }
                frame True {
                  n1092 = property on="分隔栏 2" class="Splitter"("Position"=113 ("分隔栏位置")) -> ()  [unwired: 2 in, 2 out]
                }
              }
            }
          }
          frame True {
          }
        }
        n1093 = stacked-sequence {
          seq-local: [w1469 _ _ _ _ _ _ _] -> [_ _ w1503 w1522 _ _ _ _]
          seq-local: [_ _ _ w1517 _ _ _ _] -> [_ _ _ _ w1542 _ _ _]
          frame #0 {
            w1482 = dbl[][] [[0.097818, 0.19644, 0.296487, 0.397425, 0.596183, 0.796366, 0.997293, 1.99632, 2.9953, 3.99593, 5.99668, 7.99436, 9.99492, 11.9958, 13.9951, 15.9998, 17.9991, 19.996, 22.9956, 25.9966], [0.568902, 0.952928, 1.22253, 1.42729, 1.81761, 2.11464, 2.38471, 3.58397, 4.36939, 5.05862, 5.89205, 6.46973, 6.93328, 7.23058, 7.4567, 7.62404, 7.75156, 7.85895, 8.01179, 8.16011]] ("添加的数组")
            w1478 = dbl[][] [[0.10353, 0.20285, 0.30402, 0.403475, 0.603921, 0.802667, 1.00272, 2.00307, 3.00286, 4.0031, 6.00107, 8.00206, 10.0002, 12.0013, 14.0, 16.0008, 17.999, 19.9997, 22.9991, 25.9999], [0.738465, 1.47064, 2.39299, 2.94065, 3.60823, 4.06492, 4.35973, 4.94926, 5.33625, 5.7216, 6.1826, 6.52756, 6.74406, 6.92562, 7.09031, 7.25126, 7.4079, 7.54541, 7.74854, 7.93824]] ("添加的数组")
            n1094 = Index Array(array=w1482, index (row)=0 ("索引 (行)")) -> (element=w1473:dbl[])  [unwired: 1 in]
            n1095 = Index Array(array=w1482, index (row)=1 ("索引 (行)")) -> (element=w1472:dbl[])  [unwired: 1 in]
            n1096 = Index Array(array=w1482, index (row)=0 ("索引 (行)")) -> (element=w1485:dbl[])  [unwired: 1 in]
            n1097 = Index Array(array=w1478, index (row)=0 ("索引 (行)")) -> (element=w1471:dbl[])  [unwired: 1 in]
            n1098 = Index Array(array=w1478, index (row)=1 ("索引 (行)")) -> (element=w1470:dbl[])  [unwired: 1 in]
            n1099 = Index Array(array=w1478, index (row)=0 ("索引 (行)")) -> (element=w1484:dbl[])  [unwired: 1 in]
            n1100 = Array Max & Min(array=w1485) -> (max value=w1477:dbl)  [unwired: 3 out]
            n1101 = Array Max & Min(array=w1484) -> (max value=w1476:dbl)  [unwired: 3 out]
            n1102 = Max & Min(x=w1477, y=w1476) -> (max(x,y)=w1475:dbl)  [unwired: 1 out]
            n1103 = Add(x=w1475, y=24.0) -> (x+y=w1468:dbl)
            n1104 = property on="XY图" class="XYGraph (严格)"("XScale.Maximum"=w1468) -> ()  [unwired: 2 in, 2 out]
            n1105 = Bundle("添加的数组"=w1473, "添加的数组"=w1472, "添加的数组"=w1471, "添加的数组"=w1470, w1468) -> (w1469:T24)  [unwired: 1 in]
          }
          frame #1 {
            n1106 = for {
              N: 4 -> [_]
              i -> [w1493]
              n1107 = property on="XY图" class="XYGraph (严格)"("Active Plot"=w1493, "Plot.Plot Color"=u32 16711680 ("曲线.曲线颜色"), "Plot.Point Style"=u8 0 ("曲线.点样式"), "Plot.Line Style"=u8 2 ("曲线.线条样式"), "Plot.Plot Interpolation"=u8 1 ("曲线.曲线插值")) -> ()  [unwired: 2 in, 2 out]
            }
          }
          frame #2 {
            n1108 = Unbundle(w1503) -> ("添加的数组"=w1500:dbl[], "添加的数组"=w1499:dbl[], "添加的数组"=w1498:dbl[], "添加的数组"=w1497:dbl[], w1502:dbl)
            n1109 = for {
              N: 4 -> [_]
              shift-right: [w1508] -> _
              shift-left: w1502 -> [w1508]
              tunnel: [w1505] -> w1501 mode=indexing
              i -> [w1513]
              n1110 = Multiply(x=0.1, y=w1513) -> (x*y=w1512:dbl)
              n1111 = Subtract(x=0.9, y=w1512) -> (x-y=w1511:dbl)
              n1112 = Divide(x=4.44, y=w1511) -> (x/y=w1510:dbl)
              n1113 = Build Array(w1510, w1510) -> (w1506:dbl[])
              n1114 = Build Array(0.0, w1508) -> (w1507:dbl[])
              n1115 = Bundle(w1507, w1506) -> (w1505:cluster{dbl[], dbl[]})  [unwired: 1 in]
            }
            n1116 = Bundle("添加的数组"=w1500, "添加的数组"=w1499) -> (w1496:cluster{"添加的数组":dbl[], "添加的数组":dbl[]})  [unwired: 1 in]
            n1117 = Bundle("添加的数组"=w1498, "添加的数组"=w1497) -> (w1495:cluster{"添加的数组":dbl[], "添加的数组":dbl[]})  [unwired: 1 in]
            n1118 = Build Array (concatenate)(w1501, w1496, w1495) -> (→"XY图":cluster{"添加的数组":dbl[], "添加的数组":dbl[]}[])
          }
          frame #3 {
            n1119 = Unbundle(w1522) -> (w1521:dbl)  [unwired: 4 out]
            n1120 = Subtract(x=w1521, y=3.0) -> (x-y=w1519:dbl)
            n1121 = for {
              N: 4 -> [_]
              tunnel: w1519 -> [w1532]
              tunnel: [w1525] -> w1517 mode=indexing
              i -> [w1534]
              n1122 = Multiply(x=0.1, y=w1534) -> (x*y=w1533:dbl)
              n1123 = Subtract(x=0.9, y=w1533) -> (x-y=w1531:dbl)
              n1124 = Divide(x=4.44, y=w1531) -> (x/y=w1530:dbl)
              n1125 = Bundle(w1532, w1530) -> (w1523:cluster{dbl, dbl})  [unwired: 1 in]
              n1126 = invoke on="XY图" class="XYGraph (严格)" method="Map XY To Coords"("XY"=w1523) -> ("Coords"=w1524:T22)  [unwired: 6 in, 6 out]
              n1127 = Unbundle(w1524) -> ("Horizontal"=w1528:i32, "Vertical"=w1529:i32)
              n1128 = Subtract(x=w1529, y=25) -> (x-y=w1527:i32)
              n1129 = Bundle("Horizontal"=w1528, w1527) -> (w1525:cluster{"Horizontal":i32, i32})  [unwired: 1 in]
            }
          }
          frame #4 {
            n1130 = control-ref of="字符串 11"() -> (w1541:refnum<vi>)
            n1131 = control-ref of="字符串 10"() -> (w1540:refnum<vi>)
            n1132 = control-ref of="字符串 9"() -> (w1539:refnum<vi>)
            n1133 = control-ref of="字符串 8"() -> (w1538:refnum<vi>)
            n1134 = Build Array(w1541, w1540, w1539, w1538) -> (w1543:refnum<vi>[])
            n1135 = for {
              tunnel: w1543 -> [w1549] mode=indexing
              tunnel: w1542 -> [w1544] mode=indexing
              i -> [w1555]
              n1136 = Multiply(x=w1555, y=10) -> (x*y=w1553:i32)
              n1137 = Subtract(x=90, y=w1553) -> (x-y=w1552:i32)
              n1138 = Format Into String(w1552) -> (resulting string=w1551:string)  [unwired: 3 in, 1 out]
              n1139 = Concatenate Strings(w1551, "%" ("字符串")) -> (w1548:string)
              n1140 = property class="Str"(reference=w1549, "Value"=w1548) -> (reference out=w1547:refnum<vi>)  [unwired: 1 in, 1 out]
              n1141 = property class="Str"(reference=w1547, "Text.TextColor"=u32 16711680 ("文本.文本颜色:文本颜色")) -> (reference out=w1545:refnum<vi>)  [unwired: 1 in, 1 out]
              n1142 = property class="Str"(reference=w1545, "Position"=w1544) -> ()  [unwired: 1 in, 2 out]
            }
          }
          frame #5 {
            n1143 = for {
              tunnel: string[] ["21.43", "21.43", "21.43", "21.43", "21.43", "21.45", "21.45", "21.5", "21.5", "21.48", "21.48", "21.49", "21.49", "21.52", "21.52", "21.54", "21.54", "21.56", "21.56", "21.55", "21.55", "21.52", "21.52", "21.52", "21.52", "21.55", "21.55", "21.57", "21.57", "21.55", "21.55", "21.52", "21.52", "21.58", "21.58", "21.58", "21.58", "21.56", "21.56", "21.6", "21.6", "21.53", "21.53", "21.57", "21.57", "21.53", "21.53", "21.61", "21.61", "21.61", "21.6", "21.6", "21.59", "21.59", "21.61", "21.61", "21.61", "21.61", "21.58", "21.58", "21.62", "21.62", "21.63", "21.63", "21.62", "21.62", "21.63", "21.63", "21.62", "21.62", "21.66", "21.66", "21.66", "21.66", "21.67", "21.67", "21.64", "21.64", "21.66", "21.66", "21.67", "21.67", "21.68", "21.68", "21.67", "21.67", "21.69", "21.69", "21.71", "21.71", "21.72", "21.72", "21.71", "21.71", "21.71", "21.71", "21.74", "21.74", "21.69", "21.69", "21.67", "21.67", "21.71", "21.71", "21.72", "21.72", "21.76", "21.76", "21.73", "21.73", "21.78", "21.78", "21.74", "21.74", "21.75", "21.75", "21.75", "21.75", "21.76", "21.76", "21.71", "21.71", "21.73", "21.73", "21.76", "21.76", "21.75", "21.75", "21.75", "21.75", "21.8", "21.8", "21.79", "21.79", "21.8", "21.8", "21.82", "21.82", "21.82", "21.82", "21.84", "21.84", "21.82", "21.82", "21.8", "21.8", "21.83", "21.83", "21.85", "21.85", "21.81", "21.81", "21.81", "21.81", "21.84", "21.84", "21.84", "21.83", "21.83", "21.84", "21.84", "21.85", "21.85", "21.83", "21.83", "21.83", "21.83", "21.86", "21.86", "21.88", "21.88", "21.86", "21.86", "21.87", "21.87", "21.86", "21.86", "21.88", "21.88", "21.87", "21.87", "21.91", "21.91", "21.92", "21.92", "21.92", "21.92", "21.94", "21.94", "21.94", "21.94", "21.94", "21.94", "21.94", "21.94", "21.9", "21.9", "21.92", "21.92", "21.91", "21.91", "21.93", "21.93", "21.91", "21.91", "21.92", "21.92", "21.96", "21.96", "21.95", "21.95", "21.96", "21.96", "21.96", "21.96", "21.97", "21.97", "21.96", "21.96", "21.98", "21.98", "21.99", "21.99", "21.99", "21.99", "21.95", "21.95", "21.95", "21.95", "21.99", "21.99", "21.97", "21.97", "21.97", "21.97", "21.98", "21.98", "22", "22", "22", "22", "21.97", "21.97", "21.97", "21.97", "22.01", "22.01", "22.02", "22.02", "22", "22", "22.02", "22.02", "22.02", "22.02", "22.01", "22.01", "22.02", "22.02", "22.02", "22.02", "22.04", "22.04", "21.98", "21.98", "21.99", "21.99", "22.05", "22.05", "22.06", "22.06", "22.04", "22.04", "22.04", "22.04", "22.06", "22.06", "22.04", "22.04", "22.08", "22.08", "22.02", "22.02", "22.06", "22.06", "22.07", "22.07", "22.05", "22.05", "22.04", "22.04", "22.05", "22.05", "22.08", "22.08", "22.06", "22.06", "22.05", "22.05", "22.06", "22.06", "22.08", "22.08", "22.05", "22.05", "22.06", "22.06", "22.05", "22.05", "22.08", "22.08", "22.07", "22.07", "22.07", "22.07", "22.09", "22.09", "22.11", "22.11", "22.08", "22.08", "22.09", "22.09", "22.09", "22.09", "22.08", "22.08", "22.1", "22.1", "22.1", "22.1", "22.1", "22.1", "22.1", "22.09", "22.09", "22.12", "22.12", "22.11", "22.11", "22.13", "22.13", "22.11", "22.11", "22.13", "22.13", "22.11", "22.11", "22.11", "22.11", "22.1", "22.1", "22.09", "22.09", "22.15", "22.15", "22.12", "22.12", "22.12", "22.12", "22.14", "22.14", "22.17", "22.17", "22.19", "22.19", "22.15", "22.15", "22.18", "22.18", "22.13", "22.13", "22.16", "22.16", "22.15", "22.15", "22.19", "22.19", "22.18", "22.18", "22.15", "22.15", "22.17", "22.17", "22.17", "22.17", "22.17", "22.17", "22.2", "22.2", "22.18", "22.18", "22.17", "22.17", "22.21", "22.21", "22.22", "22.22", "22.21", "22.21", "22.19", "22.19", "22.21", "22.21", "22.21", "22.21", "22.23", "22.23", "22.23", "22.23", "22.2", "22.2", "22.23", "22.23", "22.23", "22.23", "22.24", "22.24", "22.24", "22.24", "22.22", "22.22", "22.28", "22.28", "22.19", "22.19", "22.21", "22.21", "22.25", "22.25", "22.21", "22.21"] ("文本") -> [w1560] mode=indexing
              tunnel: [w1559] -> w1557 mode=indexing
              n1144 = Scan From String(input string=w1560) -> (output 1=w1559:dbl)  [unwired: 4 in, 3 out]
            }
            n1145 = property on="波形图" class="WFGraph (严格)"("Value"=w1557) -> ()  [unwired: 2 in, 2 out]
          }
          frame #6 {
            n1146 = for {
              tunnel: string[] ["0.6", "0.6", "0.6", "0.6", "0.6", "0.6", "0.6", "0.6", "0.6", "0.6", "0.6", "0.6", "0.6", "0.6", "0.6", "0.6", "0.6", "0.6", "0.6", "0.6", "0.6", "0.6", "0.6", "0.6", "0.6", "0.6", "0.6", "0.6", "0.6", "0.6", "0.6", "0.6", "0.6", "0.6", "0.6", "0.6", "0.6", "0.6", "0.6", "0.6", "0.6", "0.6", "0.6", "0.6", "0.6", "0.6", "0.6", "0.6", "0.6", "0.6", "0.6", "0.6", "0.6", "0.6", "0.6", "0.6", "0.6", "0.6", "0.6", "0.6", "0.6", "0.6", "0.6", "0.6", "0.6", "0.6", "0.6", "0.6", "0.6", "0.61", "0.61", "0.6", "0.6", "0.61", "0.61", "0.61", "0.61", "0.61", "0.61", "0.6", "0.6", "0.61", "0.61", "0.61", "0.61", "0.6", "0.6", "0.61", "0.61", "0.6", "0.6", "0.61", "0.61", "0.61", "0.61", "0.61", "0.61", "0.6", "0.6", "0.61", "0.61", "0.61", "0.61", "0.61", "0.61", "0.61", "0.61", "0.6", "0.6", "0.61", "0.61", "0.61", "0.61", "0.61", "0.61", "0.61", "0.61", "0.61", "0.61", "0.61", "0.6", "0.6", "0.61", "0.61", "0.6", "0.6", "0.61", "0.61", "0.61", "0.61", "0.61", "0.61", "0.61", "0.61", "0.61", "0.61", "0.61", "0.61", "0.6", "0.6", "0.61", "0.61", "0.61", "0.61", "0.61", "0.61", "0.61", "0.61", "0.61", "0.61", "0.61", "0.61", "0.61", "0.61", "0.61", "0.61", "0.61", "0.61", "0.61", "0.61", "0.61", "0.61", "0.61", "0.61", "0.61", "0.61", "0.61", "0.61", "0.61", "0.61", "0.61", "0.61", "0.61", "0.61", "0.61", "0.61", "0.61", "0.61", "0.61", "0.61", "0.61", "0.61", "0.61", "0.61", "0.61", "0.61", "0.61", "0.61", "0.61", "0.61", "0.61", "0.61", "0.61", "0.61", "0.61", "0.61", "0.61", "0.61", "0.61", "0.61", "0.61", "0.61", "0.61", "0.61", "0.61", "0.61", "0.61", "0.61", "0.61", "0.61", "0.61", "0.61", "0.61", "0.61", "0.61", "0.61", "0.61", "0.61", "0.61", "0.61", "0.61", "0.61", "0.61", "0.61", "0.61", "0.61", "0.61", "0.61", "0.61", "0.61", "0.61", "0.61", "0.61", "0.61", "0.61", "0.61", "0.61", "0.61", "0.61", "0.61", "0.61", "0.61", "0.61", "0.61", "0.61", "0.61", "0.61", "0.61", "0.61", "0.61", "0.61", "0.61", "0.61", "0.61", "0.61", "0.61", "0.61", "0.61", "0.61", "0.61", "0.61", "0.61", "0.61", "0.61", "0.61", "0.61", "0.61", "0.61", "0.61", "0.61", "0.61", "0.61", "0.61", "0.61", "0.61", "0.61", "0.61", "0.61", "0.61", "0.61", "0.61", "0.61", "0.61", "0.61", "0.61", "0.61", "0.61", "0.61", "0.61", "0.61", "0.61", "0.61", "0.61", "0.61", "0.61", "0.61", "0.61", "0.61", "0.61", "0.61", "0.61", "0.61", "0.61", "0.61", "0.61", "0.61", "0.61", "0.61", "0.61", "0.61", "0.61", "0.61", "0.61", "0.61", "0.61", "0.61", "0.61", "0.61", "0.61", "0.61", "0.61", "0.61", "0.61", "0.61", "0.61", "0.61", "0.61", "0.61", "0.61", "0.61", "0.61", "0.61", "0.61", "0.61", "0.61", "0.61", "0.61", "0.61", "0.61", "0.61", "0.61", "0.61", "0.61", "0.61", "0.61", "0.61", "0.61", "0.61", "0.61", "0.61", "0.61", "0.61", "0.61", "0.61", "0.61", "0.61", "0.61", "0.61", "0.61", "0.61", "0.61", "0.61", "0.61", "0.61", "0.61", "0.61", "0.61", "0.61", "0.61", "0.61", "0.61", "0.62", "0.62", "0.61", "0.61", "0.62", "0.62", "0.62", "0.62", "0.61", "0.61", "0.62", "0.62", "0.62", "0.62", "0.62", "0.62", "0.61", "0.61", "0.62", "0.62", "0.62", "0.62", "0.62", "0.62", "0.62", "0.62", "0.62", "0.62", "0.62", "0.62", "0.62", "0.62", "0.62", "0.62", "0.62", "0.62", "0.62", "0.62", "0.62", "0.62", "0.62", "0.62", "0.62", "0.62", "0.62", "0.62", "0.62", "0.62", "0.62", "0.63", "0.63", "0.63", "0.63", "0.63", "0.63", "0.63", "0.63", "0.63", "0.63", "0.63", "0.63", "0.63", "0.63", "0.63", "0.63", "0.63", "0.63", "0.63", "0.63", "0.63", "0.63", "0.63", "0.63", "0.63", "0.63", "0.63", "0.63", "0.63", "0.63", "0.63", "0.63", "0.64", "0.64", "0.64", "0.64", "0.64", "0.64", "0.64", "0.64", "0.64", "0.64", "0.64", "0.64", "0.64", "0.64", "0.64", "0.64", "0.64", "0.64", "0.64", "0.64", "0.64", "0.64", "0.64", "0.64", "0.64", "0.64", "0.64", "0.64", "0.64", "0.64", "0.64", "0.64", "0.64", "0.64", "0.64", "0.64", "0.64", "0.64", "0.64", "0.64", "0.64", "0.64", "0.64", "0.64", "0.64", "0.64", "0.64", "0.64", "0.64", "0.64", "0.64", "0.64", "0.64", "0.64", "0.64", "0.64", "0.64", "0.64", "0.64", "0.64", "0.64", "0.64", "0.64", "0.64", "0.64", "0.64", "0.64", "0.64", "0.64", "0.64", "0.64", "0.64", "0.64", "0.64", "0.65", "0.65", "0.64", "0.64", "0.64", "0.64", "0.64", "0.64", "0.64", "0.64", "0.64", "0.64", "0.64", "0.64", "0.65", "0.65", "0.65", "0.65", "0.65", "0.65", "0.65", "0.65", "0.65", "0.65", "0.65", "0.65", "0.65", "0.65", "0.65", "0.65", "0.65", "0.65", "0.65", "0.65", "0.65", "0.65", "0.65", "0.64", "0.64", "0.64", "0.64", "0.64", "0.64", "0.64", "0.64", "0.65", "0.65", "0.65", "0.65", "0.65", "0.65", "0.65", "0.65", "0.65", "0.65", "0.65", "0.65", "0.65", "0.65", "0.65", "0.65", "0.65", "0.65", "0.65", "0.65", "0.65", "0.65", "0.65", "0.65", "0.65", "0.65", "0.65", "0.65", "0.65", "0.65", "0.65", "0.65", "0.65", "0.65", "0.65", "0.65", "0.65", "0.65", "0.65", "0.65", "0.65", "0.65", "0.65", "0.65", "0.65", "0.65", "0.65", "0.65", "0.65", "0.65", "0.65", "0.65", "0.65", "0.65", "0.65", "0.65", "0.65", "0.65", "0.65", "0.65", "0.65", "0.65", "0.65", "0.65", "0.65", "0.65", "0.65", "0.65", "0.65", "0.65", "0.65", "0.65", "0.65", "0.65", "0.65", "0.65", "0.65", "0.65", "0.65", "0.65", "0.65", "0.65", "0.66", "0.66", "0.66", "0.66", "0.65", "0.65", "0.65", "0.65", "0.65", "0.65", "0.65", "0.65", "0.65", "0.65", "0.65", "0.65", "0.65", "0.65", "0.65", "0.65", "0.65", "0.65", "0.65", "0.65", "0.65", "0.65", "0.65", "0.65", "0.65", "0.65", "0.65", "0.65", "0.65", "0.65", "0.65", "0.65", "0.66", "0.66", "0.66", "0.66", "0.66", "0.66", "0.66", "0.66", "0.66", "0.66", "0.66", "0.66", "0.66", "0.66", "0.66", "0.66", "0.66", "0.66", "0.66", "0.66", "0.66", "0.65", "0.65", "0.65", "0.65", "0.66", "0.66", "0.66", "0.66", "0.66", "0.66", "0.66", "0.66", "0.66", "0.66", "0.66", "0.66", "0.66", "0.66", "0.66", "0.66", "0.66", "0.66", "0.66", "0.66", "0.66", "0.66", "0.66", "0.66", "0.66", "0.66", "0.66", "0.66", "0.66", "0.66"] ("文本") -> [w1564] mode=indexing
              tunnel: [w1563] -> w1561 mode=indexing
              n1147 = Scan From String(input string=w1564) -> (output 1=w1563:dbl)  [unwired: 4 in, 3 out]
            }
            n1148 = property on="波形图 2" class="WFGraph (严格)"("Value"=w1561) -> ()  [unwired: 2 in, 2 out]
          }
          frame #7 {
            n1149 = for {
              tunnel: string[] ["0.6", "0.6", "0.6", "0.6", "0.6", "0.6", "0.6", "0.6", "0.6", "0.6", "0.6", "0.6", "0.6", "0.6", "0.6", "0.6", "0.6", "0.6", "0.6", "0.6", "0.6", "0.6", "0.6", "0.6", "0.6", "0.6", "0.6", "0.6", "0.6", "0.6", "0.6", "0.6", "0.6", "0.6", "0.6", "0.6", "0.6", "0.6", "0.6", "0.6", "0.6", "0.6", "0.6", "0.6", "0.6", "0.6", "0.6", "0.6", "0.6", "0.6", "0.6", "0.6", "0.6", "0.6", "0.6", "0.6", "0.6", "0.6", "0.6", "0.6", "0.6", "0.6", "0.6", "0.6", "0.6", "0.6", "0.6", "0.6", "0.6", "0.61", "0.61", "0.6", "0.6", "0.61", "0.61", "0.61", "0.61", "0.61", "0.61", "0.6", "0.6", "0.61", "0.61", "0.61", "0.61", "0.6", "0.6", "0.61", "0.61", "0.6", "0.6", "0.61", "0.61", "0.61", "0.61", "0.61", "0.61", "0.6", "0.6", "0.61", "0.61", "0.61", "0.61", "0.61", "0.61", "0.61", "0.61", "0.6", "0.6", "0.61", "0.61", "0.61", "0.61", "0.61", "0.61", "0.61", "0.61", "0.61", "0.61", "0.61", "0.6", "0.6", "0.61", "0.61", "0.6", "0.6", "0.61", "0.61", "0.61", "0.61", "0.61", "0.61", "0.61", "0.61", "0.61", "0.61", "0.61", "0.61", "0.6", "0.6", "0.61", "0.61", "0.61", "0.61", "0.61", "0.61", "0.61", "0.61", "0.61", "0.61", "0.61", "0.61", "0.61", "0.61", "0.61", "0.61", "0.61", "0.61", "0.61", "0.61", "0.61", "0.61", "0.61", "0.61", "0.61", "0.61", "0.61", "0.61", "0.61", "0.61", "0.61", "0.61", "0.61", "0.61", "0.61", "0.61", "0.61", "0.61", "0.61", "0.61", "0.61", "0.61", "0.61", "0.61", "0.61", "0.61", "0.61", "0.61", "0.61", "0.61", "0.61", "0.61", "0.61", "0.61", "0.61", "0.61", "0.61", "0.61", "0.61", "0.61", "0.61", "0.61", "0.61", "0.61", "0.61", "0.61", "0.61", "0.61", "0.61", "0.61", "0.61", "0.61", "0.61", "0.61", "0.61", "0.61", "0.61", "0.61", "0.61", "0.61", "0.61", "0.61", "0.61", "0.61", "0.61", "0.61", "0.61", "0.61", "0.61", "0.61", "0.61", "0.61", "0.61", "0.61", "0.61", "0.61", "0.61", "0.61", "0.61", "0.61", "0.61", "0.61", "0.61", "0.61", "0.61", "0.61", "0.61", "0.61", "0.61", "0.61", "0.61", "0.61", "0.61", "0.61", "0.61", "0.61", "0.61", "0.61", "0.61", "0.61", "0.61", "0.61", "0.61", "0.61", "0.61", "0.61", "0.61", "0.61", "0.61", "0.61", "0.61", "0.61", "0.61", "0.61", "0.61", "0.61", "0.61", "0.61", "0.61", "0.61", "0.61", "0.61", "0.61", "0.61", "0.61", "0.61", "0.61", "0.61", "0.61", "0.61", "0.61", "0.61", "0.61", "0.61", "0.61", "0.61", "0.61", "0.61", "0.61", "0.61", "0.61", "0.61", "0.61", "0.61", "0.61", "0.61", "0.61", "0.61", "0.61", "0.61", "0.61", "0.61", "0.61", "0.61", "0.61", "0.61", "0.61", "0.61", "0.61", "0.61", "0.61", "0.61", "0.61", "0.61", "0.61", "0.61", "0.61", "0.61", "0.61", "0.61", "0.61", "0.61", "0.61", "0.61", "0.61", "0.61", "0.61", "0.61", "0.61", "0.61", "0.61", "0.61", "0.61", "0.61", "0.61", "0.61", "0.61", "0.61", "0.61", "0.61", "0.61", "0.61", "0.61", "0.61", "0.61", "0.61", "0.61", "0.61", "0.61", "0.61", "0.61", "0.61", "0.61", "0.61", "0.61", "0.61", "0.61", "0.61", "0.61", "0.61", "0.61", "0.62", "0.62", "0.61", "0.61", "0.62", "0.62", "0.62", "0.62", "0.61", "0.61", "0.62", "0.62", "0.62", "0.62", "0.62", "0.62", "0.61", "0.61", "0.62", "0.62", "0.62", "0.62", "0.62", "0.62", "0.62", "0.62", "0.62", "0.62", "0.62", "0.62", "0.62", "0.62", "0.62", "0.62", "0.62", "0.62", "0.62", "0.62", "0.62", "0.62", "0.62", "0.62", "0.62", "0.62", "0.62", "0.62", "0.62", "0.62", "0.62", "0.63", "0.63", "0.63", "0.63", "0.63", "0.63", "0.63", "0.63", "0.63", "0.63", "0.63", "0.63", "0.63", "0.63", "0.63", "0.63", "0.63", "0.63", "0.63", "0.63", "0.63", "0.63", "0.63", "0.63", "0.63", "0.63", "0.63", "0.63", "0.63", "0.63", "0.63", "0.63", "0.64", "0.64", "0.64", "0.64", "0.64", "0.64", "0.64", "0.64", "0.64", "0.64", "0.64", "0.64", "0.64", "0.64", "0.64", "0.64", "0.64", "0.64", "0.64", "0.64", "0.64", "0.64", "0.64", "0.64", "0.64", "0.64", "0.64", "0.64", "0.64", "0.64", "0.64", "0.64", "0.64", "0.64", "0.64", "0.64", "0.64", "0.64", "0.64", "0.64", "0.64", "0.64", "0.64", "0.64", "0.64", "0.64", "0.64", "0.64", "0.64", "0.64", "0.64", "0.64", "0.64", "0.64", "0.64", "0.64", "0.64", "0.64", "0.64", "0.64", "0.64", "0.64", "0.64", "0.64", "0.64", "0.64", "0.64", "0.64", "0.64", "0.64", "0.64", "0.64", "0.64", "0.64", "0.65", "0.65", "0.64", "0.64", "0.64", "0.64", "0.64", "0.64", "0.64", "0.64", "0.64", "0.64", "0.64", "0.64", "0.65", "0.65", "0.65", "0.65", "0.65", "0.65", "0.65", "0.65", "0.65", "0.65", "0.65", "0.65", "0.65", "0.65", "0.65", "0.65", "0.65", "0.65", "0.65", "0.65", "0.65", "0.65", "0.65", "0.64", "0.64", "0.64", "0.64", "0.64", "0.64", "0.64", "0.64", "0.65", "0.65", "0.65", "0.65", "0.65", "0.65", "0.65", "0.65", "0.65", "0.65", "0.65", "0.65", "0.65", "0.65", "0.65", "0.65", "0.65", "0.65", "0.65", "0.65", "0.65", "0.65", "0.65", "0.65", "0.65", "0.65", "0.65", "0.65", "0.65", "0.65", "0.65", "0.65", "0.65", "0.65", "0.65", "0.65", "0.65", "0.65", "0.65", "0.65", "0.65", "0.65", "0.65", "0.65", "0.65", "0.65", "0.65", "0.65", "0.65", "0.65", "0.65", "0.65", "0.65", "0.65", "0.65", "0.65", "0.65", "0.65", "0.65", "0.65", "0.65", "0.65", "0.65", "0.65", "0.65", "0.65", "0.65", "0.65", "0.65", "0.65", "0.65", "0.65", "0.65", "0.65", "0.65", "0.65", "0.65", "0.65", "0.65", "0.65", "0.65", "0.65", "0.66", "0.66", "0.66", "0.66", "0.65", "0.65", "0.65", "0.65", "0.65", "0.65", "0.65", "0.65", "0.65", "0.65", "0.65", "0.65", "0.65", "0.65", "0.65", "0.65", "0.65", "0.65", "0.65", "0.65", "0.65", "0.65", "0.65", "0.65", "0.65", "0.65", "0.65", "0.65", "0.65", "0.65", "0.65", "0.65", "0.66", "0.66", "0.66", "0.66", "0.66", "0.66", "0.66", "0.66", "0.66", "0.66", "0.66", "0.66", "0.66", "0.66", "0.66", "0.66", "0.66", "0.66", "0.66", "0.66", "0.66", "0.65", "0.65", "0.65", "0.65", "0.66", "0.66", "0.66", "0.66", "0.66", "0.66", "0.66", "0.66", "0.66", "0.66", "0.66", "0.66", "0.66", "0.66", "0.66", "0.66", "0.66", "0.66", "0.66", "0.66", "0.66", "0.66", "0.66", "0.66", "0.66", "0.66", "0.66", "0.66", "0.66", "0.66"] ("文本") -> [w1568] mode=indexing
              tunnel: [w1567] -> w1565 mode=indexing
              n1150 = Scan From String(input string=w1568) -> (output 1=w1567:dbl)  [unwired: 4 in, 3 out]
            }
            n1151 = property on="波形图 3" class="WFGraph (严格)"("Value"=w1565) -> ()  [unwired: 2 in, 2 out]
          }
        }
      }
      event "极化x轴网格线", "极化y轴网格线", "温度x轴网格线", "温度y轴网格线", "压力x轴网格线", "压力y轴网格线", "水质x轴网格线", "水质y轴网格线": Value Change {
        n1152 = event-data() -> ("CtlRef"=w1598:refnum<vi>, "NewVal"=w1596:bool)  [unwired: 1 in, 4 out]
        n1153 = property class="Bool (严格)"(reference=w1598) -> ("Label.Text"=w1597:string)  [unwired: 1 in, 2 out]
        n1154 = case shown="\"水质y轴网格线\"" w1597 {
          tunnel: w1596 -> [w1599 w1602 w1605 w1608 w1611 w1614 w1617 w1620]
          frame "极化x轴网格线", Default {
            n1155 = case shown="假" w1599 {
              frame False {
                n1156 = property on="XY图" class="XYGraph (严格)"("XScale.MajGrdColor"=u32 16777216 ("X标尺.网格颜色:主网格颜色")) -> ()  [unwired: 2 in, 2 out]
              }
              frame True {
                n1157 = property on="XY图" class="XYGraph (严格)"("XScale.MajGrdColor"=u32 0 ("X标尺.网格颜色:主网格颜色")) -> ()  [unwired: 2 in, 2 out]
              }
            }
          }
          frame "极化y轴网格线" {
            n1158 = case shown="假" w1602 {
              frame False {
                n1159 = property on="XY图" class="XYGraph (严格)"("YScale.MajGrdColor"=u32 16777216 ("Y标尺.网格颜色:主网格颜色")) -> ()  [unwired: 2 in, 2 out]
              }
              frame True {
                n1160 = property on="XY图" class="XYGraph (严格)"("YScale.MajGrdColor"=u32 0 ("Y标尺.网格颜色:主网格颜色")) -> ()  [unwired: 2 in, 2 out]
              }
            }
          }
          frame "温度x轴网格线" {
            n1161 = case shown="假" w1605 {
              frame False {
                n1162 = property on="波形图" class="WFGraph (严格)"("XScale.MajGrdColor"=u32 16777216 ("X标尺.网格颜色:主网格颜色")) -> ()  [unwired: 2 in, 2 out]
              }
              frame True {
                n1163 = property on="波形图" class="WFGraph (严格)"("XScale.MajGrdColor"=u32 0 ("X标尺.网格颜色:主网格颜色")) -> ()  [unwired: 2 in, 2 out]
              }
            }
          }
          frame "温度y轴网格线" {
            n1164 = case shown="假" w1608 {
              frame False {
                n1165 = property on="波形图" class="WFGraph (严格)"("YScale.MajGrdColor"=u32 16777216 ("Y标尺.网格颜色:主网格颜色")) -> ()  [unwired: 2 in, 2 out]
              }
              frame True {
                n1166 = property on="波形图" class="WFGraph (严格)"("YScale.MajGrdColor"=u32 0 ("Y标尺.网格颜色:主网格颜色")) -> ()  [unwired: 2 in, 2 out]
              }
            }
          }
          frame "压力x轴网格线" {
            n1167 = case shown="假" w1611 {
              frame False {
                n1168 = property on="波形图 2" class="WFGraph (严格)"("XScale.MajGrdColor"=u32 16777216 ("X标尺.网格颜色:主网格颜色")) -> ()  [unwired: 2 in, 2 out]
              }
              frame True {
                n1169 = property on="波形图 2" class="WFGraph (严格)"("XScale.MajGrdColor"=u32 0 ("X标尺.网格颜色:主网格颜色")) -> ()  [unwired: 2 in, 2 out]
              }
            }
          }
          frame "压力y轴网格线" {
            n1170 = case shown="假" w1614 {
              frame False {
                n1171 = property on="波形图 2" class="WFGraph (严格)"("YScale.MajGrdColor"=u32 16777216 ("Y标尺.网格颜色:主网格颜色")) -> ()  [unwired: 2 in, 2 out]
              }
              frame True {
                n1172 = property on="波形图 2" class="WFGraph (严格)"("YScale.MajGrdColor"=u32 0 ("Y标尺.网格颜色:主网格颜色")) -> ()  [unwired: 2 in, 2 out]
              }
            }
          }
          frame "水质x轴网格线" {
            n1173 = case shown="假" w1617 {
              frame False {
                n1174 = property on="波形图 3" class="WFGraph (严格)"("XScale.MajGrdColor"=u32 16777216 ("X标尺.网格颜色:主网格颜色")) -> ()  [unwired: 2 in, 2 out]
              }
              frame True {
                n1175 = property on="波形图 3" class="WFGraph (严格)"("XScale.MajGrdColor"=u32 0 ("X标尺.网格颜色:主网格颜色")) -> ()  [unwired: 2 in, 2 out]
              }
            }
          }
          frame "水质y轴网格线" {
            n1176 = case shown="假" w1620 {
              frame False {
                n1177 = property on="波形图 3" class="WFGraph (严格)"("YScale.MajGrdColor"=u32 16777216 ("X标尺.网格颜色:主网格颜色")) -> ()  [unwired: 2 in, 2 out]
              }
              frame True {
                n1178 = property on="波形图 3" class="WFGraph (严格)"("YScale.MajGrdColor"=u32 0 ("X标尺.网格颜色:主网格颜色")) -> ()  [unwired: 2 in, 2 out]
              }
            }
          }
        }
      }
      event "寻找设备": Value Change {
        n1179 = event-data() -> ()  [unwired: 1 in, 6 out]
        n1180 = flat-sequence {
          tunnel: [w1630] -> w1627
          tunnel: [w1635] -> w1628
          tunnel: w1627 -> [w1635]
          tunnel: w1628 -> [w1639]
          tunnel: [w1638] -> w1625
          tunnel: [w1640] -> w1626
          tunnel: w1625 -> [w1640]
          tunnel: w1626 -> [w1644]
          tunnel: [w1642] -> w1623
          tunnel: [w1645] -> w1624
          tunnel: w1623 -> [w1645]
          tunnel: w1624 -> [w1648]
          frame #0 {
            n1181 = property on="串口号" class="Ring (严格)"() -> ("RingText.Text"=w1634:string)  [unwired: 2 in, 2 out]
            n1182 = To Variant(anything=w1634) -> (Variant=w1633:variant)
            n1183 = Variant To Data(type=refnum<visa-resource-name> refnum ("VISA resource name out"), Variant=w1633) -> (data=w1631:refnum<visa-resource-name>)  [unwired: 1 in, 1 out]
            n1184 = VISA Write(VISA resource name=w1631, write buffer="VOLT 10.00") -> (VISA resource name out=w1630:refnum<visa-resource-name>)  [unwired: 1 in, 2 out]
          }
          frame #1 {
            n1185 = Wait (ms)(milliseconds to wait=u32 100 ("等待时间（毫秒）")) -> ()  [unwired: 1 out]
          }
          frame #2 {
            n1186 = VISA Write(VISA resource name=w1639, write buffer="CURR 0") -> (VISA resource name out=w1638:refnum<visa-resource-name>)  [unwired: 1 in, 2 out]
          }
          frame #3 {
            n1187 = Wait (ms)(milliseconds to wait=u32 100 ("等待时间（毫秒）")) -> ()  [unwired: 1 out]
          }
          frame #4 {
            n1188 = VISA Write(VISA resource name=w1644, write buffer="OUTP ON") -> (VISA resource name out=w1642:refnum<visa-resource-name>)  [unwired: 1 in, 2 out]
          }
          frame #5 {
            n1189 = Wait (ms)(milliseconds to wait=u32 3000 ("等待时间（毫秒）")) -> ()  [unwired: 1 out]
          }
          frame #6 {
            n1190 = VISA Write(VISA resource name=w1648, write buffer="OUTP OFF") -> ()  [unwired: 1 in, 3 out]
          }
        }
      }
      event "连接": Mouse Enter {
        n1191 = event-data() -> ()  [unwired: 1 in, 4 out]
        n1192 = disable-structure shown="禁用" {
          frame Disabled {
            n1193 = flat-sequence {
              frame #0 {
                n1194 = flat-sequence {
                  frame #0 {
                    n1195 = stacked-sequence {
                      frame #0 {
                        n1196 = property on="分隔栏 4" class="Splitter"() -> ("Position"=w1649:i32)  [unwired: 2 in, 2 out]
                        n1197 = Add(x=w1649, y=32 ("分隔栏位置")) -> (x+y=w1651:i32)
                        n1198 = property on="分隔栏 5" class="Splitter"("Position"=w1651) -> ()  [unwired: 2 in, 2 out]
                      }
                      frame #1 {
                        n1199 = property on="分隔栏 4" class="Splitter"() -> ("Position"=w1654:i32)  [unwired: 2 in, 2 out]
                        n1200 = Add(x=w1654, y=62 ("分隔栏位置")) -> (x+y=w1653:i32)
                        n1201 = property on="分隔栏 6" class="Splitter"("Position"=w1653) -> ()  [unwired: 2 in, 2 out]
                      }
                      frame #2 {
                        n1202 = property on="分隔栏 4" class="Splitter"() -> ("Position"=w1657:i32)  [unwired: 2 in, 2 out]
                        n1203 = Add(x=w1657, y=92 ("分隔栏位置")) -> (x+y=w1656:i32)
                        n1204 = property on="分隔栏 7" class="Splitter"("Position"=w1656) -> ()  [unwired: 2 in, 2 out]
                      }
                      frame #3 {
                        n1205 = property on="分隔栏 4" class="Splitter"() -> ("Position"=w1660:i32)  [unwired: 2 in, 2 out]
                        n1206 = Add(x=w1660, y=122 ("分隔栏位置")) -> (x+y=w1658:i32)
                        n1207 = property on="分隔栏 8" class="Splitter"("Position"=w1658) -> ()  [unwired: 2 in, 2 out]
                      }
                    }
                  }
                  frame #1 {
                    n1208 = property on="1" class="Bool (严格)"("Value"=FALSE ("1")) -> ()  [unwired: 2 in, 2 out]
                    n1209 = property on="2" class="Bool (严格)"("Value"=FALSE ("2")) -> ()  [unwired: 2 in, 2 out]
                    n1210 = property on="3" class="Bool (严格)"("Value"=FALSE ("3")) -> ()  [unwired: 2 in, 2 out]
                    n1211 = property on="4" class="Bool (严格)"("Value"=FALSE ("4")) -> ()  [unwired: 2 in, 2 out]
                  }
                  frame #2 {
                    n1212 = control-ref of="窗格 8"() -> (w1669:refnum<vi>)
                    n1213 = control-ref of="窗格 7"() -> (w1670:refnum<vi>)
                    n1214 = control-ref of="窗格 6"() -> (w1671:refnum<vi>)
                    n1215 = control-ref of="窗格 9"() -> (w1672:refnum<vi>)
                    n1216 = property class="Pane"(reference=w1669, "VertScrollbarVisibility"=T3."Always Off" ("垂直滚动条可见")) -> ()  [unwired: 1 in, 2 out]
                    n1217 = property class="Pane"(reference=w1670, "VertScrollbarVisibility"=T3."Always Off" ("垂直滚动条可见")) -> ()  [unwired: 1 in, 2 out]
                    n1218 = property class="Pane"(reference=w1671, "VertScrollbarVisibility"=T3."Always Off" ("垂直滚动条可见")) -> ()  [unwired: 1 in, 2 out]
                    n1219 = property class="Pane"(reference=w1672, "VertScrollbarVisibility"=T3."Always Off" ("垂直滚动条可见")) -> ()  [unwired: 1 in, 2 out]
                  }
                }
              }
              frame #1 {
                n1220 = property on="分隔栏 3" class="Splitter"() -> ("Position"=w1675:i32)  [unwired: 2 in, 2 out]
                n1221 = Equal?(x=w1675, y=116) -> (x = y?=w1674:bool)
                n1222 = case shown="假" w1674 {
                  frame False {
                    n1223 = property on="分隔栏 3" class="Splitter"() -> ("Position"=w1677:i32)  [unwired: 2 in, 2 out]
                    n1224 = Greater?(x=w1677, y=508) -> (0:w1676:bool)
                    n1225 = case shown="真" w1676 {
                      frame False {
                      }
                      frame True {
                        n1226 = while {
                          i -> [w1686]
                          stop <- w1679 stop-if-true
                          n1227 = Multiply(x=10, y=w1686) -> (x*y=w1683:i32)
                          n1228 = Subtract(x=509, y=w1683) -> (x-y=w1680:i32)
                          n1229 = Less?(x=w1680, y=166) -> (x < y?=w1681:bool)
                          n1230 = case shown="真" w1681 {
                            tunnel: w1680 -> [w1687 _]
                            tunnel: [FALSE TRUE] -> w1679
                            frame False {
                              n1231 = property on="分隔栏 3" class="Splitter"("Position"=w1687) -> ()  [unwired: 2 in, 2 out]
                            }
                            frame True {
                              n1232 = property on="分隔栏 3" class="Splitter"("Position"=116 ("分隔栏位置")) -> ()  [unwired: 2 in, 2 out]
                            }
                          }
                        }
                      }
                    }
                  }
                  frame True {
                  }
                }
              }
              frame #2 {
                n1233 = while {
                  tunnel: u32 10 ("Delay(ms)") -> [w1695]
                  stop <- w1696 stop-if-true
                  n1234 = property on="分隔栏 2" class="Splitter"() -> ("Position"=w1692:i32)  [unwired: 2 in, 2 out]
                  n1235 = Wait (ms)(milliseconds to wait=w1695) -> ()  [unwired: 1 out]
                  n1236 = Subtract(x=510 ("y"), y=w1692) -> (x-y=w1699:i32)
                  n1237 = expression code="x/10"(w1699) -> (w1698:i32)
                  n1238 = Round Toward -Infinity(1:w1698) -> (0:w1697:i32)
                  n1239 = Add(x=w1692, y=w1697) -> (x+y=w1693:i32)
                  n1240 = Equal To 0?(x=w1697) -> (x = 0?=w1696:bool)
                  n1241 = property on="分隔栏 2" class="Splitter"("Position"=w1693) -> ()  [unwired: 2 in, 2 out]
                }
              }
            }
          }
          frame Enabled {
          }
        }
      }
      event "配置": Mouse Enter {
        n1242 = event-data() -> ()  [unwired: 1 in, 4 out]
        n1243 = disable-structure shown="禁用" {
          frame Disabled {
            n1244 = flat-sequence {
              frame #0 {
                n1245 = flat-sequence {
                  frame #0 {
                    n1246 = stacked-sequence {
                      frame #0 {
                        n1247 = property on="分隔栏 4" class="Splitter"() -> ("Position"=w1701:i32)  [unwired: 2 in, 2 out]
                        n1248 = Add(x=w1701, y=32 ("分隔栏位置")) -> (x+y=w1703:i32)
                        n1249 = property on="分隔栏 5" class="Splitter"("Position"=w1703) -> ()  [unwired: 2 in, 2 out]
                      }
                      frame #1 {
                        n1250 = property on="分隔栏 4" class="Splitter"() -> ("Position"=w1706:i32)  [unwired: 2 in, 2 out]
                        n1251 = Add(x=w1706, y=62 ("分隔栏位置")) -> (x+y=w1705:i32)
                        n1252 = property on="分隔栏 6" class="Splitter"("Position"=w1705) -> ()  [unwired: 2 in, 2 out]
                      }
                      frame #2 {
                        n1253 = property on="分隔栏 4" class="Splitter"() -> ("Position"=w1709:i32)  [unwired: 2 in, 2 out]
                        n1254 = Add(x=w1709, y=92 ("分隔栏位置")) -> (x+y=w1708:i32)
                        n1255 = property on="分隔栏 7" class="Splitter"("Position"=w1708) -> ()  [unwired: 2 in, 2 out]
                      }
                      frame #3 {
                        n1256 = property on="分隔栏 4" class="Splitter"() -> ("Position"=w1712:i32)  [unwired: 2 in, 2 out]
                        n1257 = Add(x=w1712, y=122 ("分隔栏位置")) -> (x+y=w1710:i32)
                        n1258 = property on="分隔栏 8" class="Splitter"("Position"=w1710) -> ()  [unwired: 2 in, 2 out]
                      }
                    }
                  }
                  frame #1 {
                    n1259 = property on="1" class="Bool (严格)"("Value"=FALSE ("1")) -> ()  [unwired: 2 in, 2 out]
                    n1260 = property on="2" class="Bool (严格)"("Value"=FALSE ("2")) -> ()  [unwired: 2 in, 2 out]
                    n1261 = property on="3" class="Bool (严格)"("Value"=FALSE ("3")) -> ()  [unwired: 2 in, 2 out]
                    n1262 = property on="4" class="Bool (严格)"("Value"=FALSE ("4")) -> ()  [unwired: 2 in, 2 out]
                  }
                  frame #2 {
                    n1263 = control-ref of="窗格 8"() -> (w1721:refnum<vi>)
                    n1264 = control-ref of="窗格 7"() -> (w1722:refnum<vi>)
                    n1265 = control-ref of="窗格 6"() -> (w1723:refnum<vi>)
                    n1266 = control-ref of="窗格 9"() -> (w1724:refnum<vi>)
                    n1267 = property class="Pane"(reference=w1721, "VertScrollbarVisibility"=T3."Always Off" ("垂直滚动条可见")) -> ()  [unwired: 1 in, 2 out]
                    n1268 = property class="Pane"(reference=w1722, "VertScrollbarVisibility"=T3."Always Off" ("垂直滚动条可见")) -> ()  [unwired: 1 in, 2 out]
                    n1269 = property class="Pane"(reference=w1723, "VertScrollbarVisibility"=T3."Always Off" ("垂直滚动条可见")) -> ()  [unwired: 1 in, 2 out]
                    n1270 = property class="Pane"(reference=w1724, "VertScrollbarVisibility"=T3."Always Off" ("垂直滚动条可见")) -> ()  [unwired: 1 in, 2 out]
                  }
                }
              }
              frame #1 {
                n1271 = property on="分隔栏 2" class="Splitter"() -> ("Position"=w1726:i32)  [unwired: 2 in, 2 out]
                n1272 = Equal?(x=w1726, y=113) -> (x = y?=w1727:bool)
                n1273 = case shown="假" w1727 {
                  frame False {
                    n1274 = while {
                      i -> [w1735]
                      stop <- w1728 stop-if-true
                      n1275 = Multiply(x=10, y=w1735) -> (x*y=w1732:i32)
                      n1276 = Subtract(x=448, y=w1732) -> (x-y=w1729:i32)
                      n1277 = Less?(x=w1729, y=163) -> (x < y?=w1730:bool)
                      n1278 = case shown="假" w1730 {
                        tunnel: w1729 -> [w1736 _]
                        tunnel: [FALSE TRUE] -> w1728
                        frame False {
                          n1279 = property on="分隔栏 2" class="Splitter"("Position"=w1736) -> ()  [unwired: 2 in, 2 out]
                        }
                        frame True {
                          n1280 = property on="分隔栏 2" class="Splitter"("Position"=113 ("分隔栏位置")) -> ()  [unwired: 2 in, 2 out]
                        }
                      }
                    }
                  }
                  frame True {
                  }
                }
              }
              frame #2 {
                n1281 = while {
                  tunnel: 10 -> [w1744]
                  stop <- w1745 stop-if-true
                  n1282 = property on="分隔栏 3" class="Splitter"() -> ("Position"=w1742:i32)  [unwired: 2 in, 2 out]
                  n1283 = Wait (ms)(milliseconds to wait=w1744) -> ()  [unwired: 1 out]
                  n1284 = Subtract(x=514, y=w1742) -> (x-y=w1748:i32)
                  n1285 = expression code="x/10"(w1748) -> (w1747:i32)
                  n1286 = Round Toward -Infinity(1:w1747) -> (0:w1746:i32)
                  n1287 = Add(x=w1742, y=w1746) -> (x+y=w1743:i32)
                  n1288 = Equal To 0?(x=w1746) -> (x = 0?=w1745:bool)
                  n1289 = property on="分隔栏 3" class="Splitter"("Position"=w1743) -> ()  [unwired: 2 in, 2 out]
                }
              }
            }
            n1290 = property on="选项卡控件 2" class="TabCtl (严格)"("Value"=enum32{"    设置界面", "实时数据", "选项卡 3"}."    设置界面" ("选项卡控件 2")) -> ()  [unwired: 2 in, 2 out]
          }
          frame Enabled {
          }
        }
      }
      event "分析": Mouse Enter {
        n1291 = event-data() -> ()  [unwired: 1 in, 4 out]
      }
      event "开始测量", "开始测量 2", "开始测量 3", "开始测量 4": Value Change {
        n1292 = event-data() -> ("CtlRef"=w1752:refnum<vi>, "NewVal"=w1750:bool)  [unwired: 1 in, 4 out]
        n1293 = property class="Bool (严格)"(reference=w1752) -> ("Label.Text"=w1751:string)  [unwired: 1 in, 2 out]
        n1294 = property on="测试项目" class="RadioBtnsControl (严格)"() -> ("Value"=w1749:enum32{"EIS", "极化曲线", "耐久性曲线", "线性扫描"})  [unwired: 2 in, 2 out]
        n1295 = case shown="\"极化曲线\"" w1749 {
          tunnel: w1751 -> [_ w1754 w1903 _]
          tunnel: w1750 -> [_ w1753 w1904 _]
          frame "EIS", Default {
          }
          frame "极化曲线" {
            n1296 = case shown="假" w1753 {
              tunnel: w1754 -> [w1755 w1782]
              frame False {
                n1297 = case shown="\"开始测量\", 默认" w1755 {
                  frame "开始测量", Default {
                    n1298 = flat-sequence {
                      frame #0 {
                        n1299 = Get Date/Time String() -> (date string=w1759:string, time string=w1757:string)  [unwired: 3 in]
                        n1300 = Concatenate Strings(w1759, " " ("字符串"), w1757) -> (w1756:string)
                        n1301 = property on="停止测试时间:" class="Str"("Value"=w1756) -> ()  [unwired: 2 in, 2 out]
                      }
                      frame #1 {
                        n1302 = property on="数组 4" class="Arr (严格)"() -> ("Value"=w1760:refnum<vi>[])  [unwired: 2 in, 2 out]
                        n1303 = for {
                          tunnel: w1760 -> [w1763] mode=indexing
                          n1304 = invoke class="VI" method="FP.Open"(reference=w1763, "State"=T15."Hidden" ("状态")) -> (reference out=w1762:refnum<vi>)  [unwired: 3 in, 4 out]
                          n1305 = invoke class="VI" method="Abort VI"(reference=w1762) -> (reference out=w1765:refnum<vi>)  [unwired: 2 in, 2 out]
                          n1306 = invoke class="VI" method="FP.Close"(reference=w1765) -> (reference out=w1764:refnum<vi>)  [unwired: 2 in, 2 out]
                          n1307 = Close Reference(reference=w1764) -> ()  [unwired: 1 in, 1 out]
                        }
                      }
                      frame #2 {
                        n1308 = property on="数组 4" class="Arr (严格)"("Value"=refnum<vi>[] [] ("数组 4")) -> ()  [unwired: 2 in, 2 out]
                      }
                    }
                  }
                  frame "开始测量 2" {
                    n1309 = flat-sequence {
                      frame #0 {
                        n1310 = property on="数组 5" class="Arr (严格)"() -> ("Value"=w1767:refnum<vi>[])  [unwired: 2 in, 2 out]
                        n1311 = for {
                          tunnel: w1767 -> [w1770] mode=indexing
                          n1312 = invoke class="VI" method="Abort VI"(reference=w1770) -> (reference out=w1769:refnum<vi>)  [unwired: 2 in, 2 out]
                          n1313 = invoke class="VI" method="FP.Close"(reference=w1769) -> (reference out=w1768:refnum<vi>)  [unwired: 2 in, 2 out]
                          n1314 = Close Reference(reference=w1768) -> ()  [unwired: 1 in, 1 out]
                        }
                      }
                      frame #1 {
                        n1315 = property on="数组 5" class="Arr (严格)"("Value"=refnum<vi>[] [] ("数组 5")) -> ()  [unwired: 2 in, 2 out]
                      }
                    }
                  }
                  frame "开始测量 3" {
                    n1316 = flat-sequence {
                      frame #0 {
                        n1317 = property on="数组 6" class="Arr (严格)"() -> ("Value"=w1772:refnum<vi>[])  [unwired: 2 in, 2 out]
                        n1318 = for {
                          tunnel: w1772 -> [w1775] mode=indexing
                          n1319 = invoke class="VI" method="Abort VI"(reference=w1775) -> (reference out=w1774:refnum<vi>)  [unwired: 2 in, 2 out]
                          n1320 = invoke class="VI" method="FP.Close"(reference=w1774) -> (reference out=w1773:refnum<vi>)  [unwired: 2 in, 2 out]
                          n1321 = Close Reference(reference=w1773) -> ()  [unwired: 1 in, 1 out]
                        }
                      }
                      frame #1 {
                        n1322 = property on="数组 6" class="Arr (严格)"("Value"=refnum<vi>[] [] ("数组 6")) -> ()  [unwired: 2 in, 2 out]
                      }
                    }
                  }
                  frame "开始测量 4" {
                    n1323 = flat-sequence {
                      frame #0 {
                        n1324 = property on="数组 7" class="Arr (严格)"() -> ("Value"=w1777:refnum<vi>[])  [unwired: 2 in, 2 out]
                        n1325 = for {
                          tunnel: w1777 -> [w1780] mode=indexing
                          n1326 = invoke class="VI" method="Abort VI"(reference=w1780) -> (reference out=w1779:refnum<vi>)  [unwired: 2 in, 2 out]
                          n1327 = invoke class="VI" method="FP.Close"(reference=w1779) -> (reference out=w1778:refnum<vi>)  [unwired: 2 in, 2 out]
                          n1328 = Close Reference(reference=w1778) -> ()  [unwired: 1 in, 1 out]
                        }
                      }
                      frame #1 {
                        n1329 = property on="数组 7" class="Arr (严格)"("Value"=refnum<vi>[] [] ("数组 7")) -> ()  [unwired: 2 in, 2 out]
                      }
                    }
                  }
                }
              }
              frame True {
                n1330 = case shown="\"开始测量\", 默认" w1782 {
                  frame "开始测量", Default {
                    n1331 = control-ref of="温度显示"() -> (w1805:refnum<vi>)
                    n1332 = control-ref of="水质1"() -> (w1806:refnum<vi>)
                    n1333 = control-ref of="温度1"() -> (w1807:refnum<vi>)
                    n1334 = Get Date/Time String() -> (date string=w1789:string, time string=w1787:string)  [unwired: 3 in]
                    n1335 = control-ref of="所有数据"() -> (w1808:refnum<vi>)
                    n1336 = control-ref of="数值"() -> (w1809:refnum<vi>)
                    n1337 = control-ref of="极化曲线1"() -> (w1810:refnum<vi>)
                    n1338 = control-ref of="极化电压1"() -> (w1811:refnum<vi>)
                    n1339 = control-ref of="极化电流1"() -> (w1812:refnum<vi>)
                    n1340 = control-ref of="电压1"() -> (w1813:refnum<vi>)
                    n1341 = control-ref of="电流1"() -> (w1814:refnum<vi>)
                    n1342 = Concatenate Strings(w1789, " " ("字符串"), w1787) -> (w1786:string)
                    n1343 = property on="开始测试时间:" class="Str"("Value"=w1786) -> ()  [unwired: 2 in, 2 out]
                    n1344 = property on="用户：" class="Str"() -> ("Value"=w1803:string)  [unwired: 2 in, 2 out]
                    n1345 = property on="测试类型 2" class="Str"() -> ("Value"=w1802:string)  [unwired: 2 in, 2 out]
                    n1346 = Bundle By Name(cluster=cluster{"用户名":string, "项目名称":string} {"用户名"="", "项目名称"=""}, "用户名"=w1803, "项目名称"=w1802) -> (w1801:cluster{"用户名":string, "项目名称":string})
                    n1347 = call <vilib>:"Application Directory.vi"() -> ("Application Directory"=w1785:path)
                    n1348 = Build Path(base path=w1785, name or relative path="pem\\电源函数\\输出调用01.vi") -> (appended path=w1783:path)
                    n1349 = control-ref of="压力1"() -> (w1793:refnum<vi>)
                    n1350 = property on="数组" class="Arr (严格)"() -> ("Value"=w1791:string[][])  [unwired: 2 in, 2 out]
                    n1351 = Bundle By Name(cluster=T16 {"所有数据"=refnum, "数值"=refnum, "极化曲线1"=refnum, "极化电压1"=refnum, "极化电流1"=refnum, "电压1"=refnum, "电流1"=refnum, "水质1"=refnum, "温度1"=refnum, "温度显示"=refnum, "压力1"=refnum}, "所有数据"=w1808, "数值"=w1809, "极化曲线1"=w1810, "极化电压1"=w1811, "极化电流1"=w1812, "电压1"=w1813, "电流1"=w1814, "水质1"=w1806, "温度1"=w1807, "温度显示"=w1805, "压力1"=w1793) -> (w1792:T16)
                    n1352 = Open VI Reference(type specifier VI Refnum (for type only)=refnum<vi> refnum ("类型说明符VI引用句柄（仅用于类型）"), vi path=w1783, options=128 ("选项")) -> (vi reference=w1804:refnum<vi>)  [unwired: 3 in, 1 out]
                    n1353 = property on="VISA resource name 3" class="VISAName"() -> ("Value"=w1815:refnum<visa-resource-name>)  [unwired: 2 in, 2 out]
                    n1354 = control-ref of="字符串 4"() -> (w1790:refnum<vi>)
                    n1355 = call-by-ref "开始异步调用"(reference=w1804, "输出簇"=w1801, "数组"=w1791, "字符串"=w1815, "输出簇 2"=w1792, "Str引用句柄"=w1790) -> (reference out=w1798:refnum<vi>)  [unwired: 12 in, 1 out]
                    n1356 = property on="数组 4" class="Arr (严格)"() -> ("Value"=w1800:refnum<vi>[])  [unwired: 2 in, 2 out]
                    n1357 = Insert Into Array(array=w1800, new element=w1798) -> (w1799:refnum<vi>[])  [unwired: 1 in]
                    n1358 = property on="数组 4" class="Arr (严格)"("Value"=w1799) -> ()  [unwired: 2 in, 2 out]
                  }
                  frame "开始测量 2" {
                    n1359 = property on="数组 10" class="Arr (严格)"() -> ("Value"=w1821:string[][])  [unwired: 2 in, 2 out]
                    n1360 = property on="用户：" class="Str"() -> ("Value"=w1840:string)  [unwired: 2 in, 2 out]
                    n1361 = property on="测试类型 2" class="Str"() -> ("Value"=w1839:string)  [unwired: 2 in, 2 out]
                    n1362 = Bundle By Name(cluster=cluster{"用户名":string, "项目名称":string} {"用户名"="", "项目名称"=""}, "用户名"=w1840, "项目名称"=w1839) -> (w1837:cluster{"用户名":string, "项目名称":string})
                    n1363 = control-ref of="电流2"() -> (w1825:refnum<vi>)
                    n1364 = control-ref of="电压2"() -> (w1826:refnum<vi>)
                    n1365 = control-ref of="极化电流2"() -> (w1827:refnum<vi>)
                    n1366 = control-ref of="极化曲线2"() -> (w1829:refnum<vi>)
                    n1367 = control-ref of="极化电压2"() -> (w1828:refnum<vi>)
                    n1368 = call <vilib>:"Application Directory.vi"() -> ("Application Directory"=w1818:path)
                    n1369 = control-ref of="数值 2"() -> (w1830:refnum<vi>)
                    n1370 = Build Path(base path=w1818, name or relative path="pem\\电源函数\\输出调用02.vi") -> (appended path=w1816:path)
                    n1371 = control-ref of="所有数据2"() -> (w1831:refnum<vi>)
                    n1372 = control-ref of="水质2"() -> (w1834:refnum<vi>)
                    n1373 = control-ref of="温度2"() -> (w1833:refnum<vi>)
                    n1374 = control-ref of="温度显示 2"() -> (w1832:refnum<vi>)
                    n1375 = control-ref of="压力2"() -> (w1822:refnum<vi>)
                    n1376 = Bundle By Name(cluster=T17 {"水质2"=refnum, "温度2"=refnum, "温度显示 2"=refnum, "所有数据2"=refnum, "数值 2"=refnum, "极化曲线2"=refnum, "极化电压2"=refnum, "极化电流2"=refnum, "电压2"=refnum, "电流2"=refnum, "压力2"=refnum}, "水质2"=w1834, "温度2"=w1833, "温度显示 2"=w1832, "所有数据2"=w1831, "数值 2"=w1830, "极化曲线2"=w1829, "极化电压2"=w1828, "极化电流2"=w1827, "电压2"=w1826, "电流2"=w1825, "压力2"=w1822) -> (w1820:T17)
                    n1377 = Open VI Reference(type specifier VI Refnum (for type only)=refnum<vi> refnum ("类型说明符VI引用句柄（仅用于类型）"), vi path=w1816, options=128 ("选项")) -> (vi reference=w1843:refnum<vi>)  [unwired: 3 in, 1 out]
                    n1378 = property on="VISA resource name 3" class="VISAName"() -> ("Value"=w1844:refnum<visa-resource-name>)  [unwired: 2 in, 2 out]
                    n1379 = control-ref of="字符串 5"() -> (w1819:refnum<vi>)
                    n1380 = call-by-ref "开始异步调用"(reference=w1843, "输出簇"=w1837, "数组"=w1821, "字符串"=w1844, "输出簇 2"=w1820, "Str引用句柄"=w1819) -> (reference out=w1836:refnum<vi>)  [unwired: 12 in, 1 out]
                    n1381 = property on="数组 5" class="Arr (严格)"() -> ("Value"=w1824:refnum<vi>[])  [unwired: 2 in, 2 out]
                    n1382 = Insert Into Array(array=w1824, new element=w1836) -> (w1823:refnum<vi>[])  [unwired: 1 in]
                    n1383 = property on="数组 5" class="Arr (严格)"("Value"=w1823) -> ()  [unwired: 2 in, 2 out]
                  }
                  frame "开始测量 3" {
                    n1384 = property on="用户：" class="Str"() -> ("Value"=w1865:string)  [unwired: 2 in, 2 out]
                    n1385 = property on="测试类型 2" class="Str"() -> ("Value"=w1864:string)  [unwired: 2 in, 2 out]
                    n1386 = control-ref of="水质3"() -> (w1863:refnum<vi>)
                    n1387 = control-ref of="温度3"() -> (w1862:refnum<vi>)
                    n1388 = control-ref of="温度显示 3"() -> (w1861:refnum<vi>)
                    n1389 = control-ref of="所有数据3"() -> (w1860:refnum<vi>)
                    n1390 = control-ref of="数值 3"() -> (w1859:refnum<vi>)
                    n1391 = control-ref of="极化曲线3"() -> (w1858:refnum<vi>)
                    n1392 = control-ref of="极化电压3"() -> (w1857:refnum<vi>)
                    n1393 = control-ref of="极化电流3"() -> (w1856:refnum<vi>)
                    n1394 = control-ref of="电压3"() -> (w1855:refnum<vi>)
                    n1395 = control-ref of="电流3"() -> (w1854:refnum<vi>)
                    n1396 = property on="数组 11" class="Arr (严格)"() -> ("Value"=w1849:string[][])  [unwired: 2 in, 2 out]
                    n1397 = Bundle By Name(cluster=cluster{"用户名":string, "项目名称":string} {"用户名"="", "项目名称"=""}, "用户名"=w1865, "项目名称"=w1864) -> (w1871:cluster{"用户名":string, "项目名称":string})
                    n1398 = call <vilib>:"Application Directory.vi"() -> ("Application Directory"=w1847:path)
                    n1399 = Build Path(base path=w1847, name or relative path="pem\\电源函数\\输出调用03.vi") -> (appended path=w1845:path)
                    n1400 = control-ref of="压力3"() -> (w1850:refnum<vi>)
                    n1401 = Bundle By Name(cluster=T18 {"水质3"=refnum, "温度3"=refnum, "温度显示 3"=refnum, "所有数据3"=refnum, "数值 3"=refnum, "极化曲线3"=refnum, "极化电压3"=refnum, "极化电流3"=refnum, "电压3"=refnum, "电流3"=refnum, "压力3"=refnum}, "水质3"=w1863, "温度3"=w1862, "温度显示 3"=w1861, "所有数据3"=w1860, "数值 3"=w1859, "极化曲线3"=w1858, "极化电压3"=w1857, "极化电流3"=w1856, "电压3"=w1855, "电流3"=w1854, "压力3"=w1850) -> (w1853:T18)
                    n1402 = Open VI Reference(type specifier VI Refnum (for type only)=refnum<vi> refnum ("类型说明符VI引用句柄（仅用于类型）"), vi path=w1845, options=128 ("选项")) -> (vi reference=w1872:refnum<vi>)  [unwired: 3 in, 1 out]
                    n1403 = property on="VISA resource name 3" class="VISAName"() -> ("Value"=w1873:refnum<visa-resource-name>)  [unwired: 2 in, 2 out]
                    n1404 = control-ref of="字符串 6"() -> (w1848:refnum<vi>)
                    n1405 = property on="数组 6" class="Arr (严格)"() -> ("Value"=w1852:refnum<vi>[])  [unwired: 2 in, 2 out]
                    n1406 = call-by-ref "开始异步调用"(reference=w1872, "输出簇"=w1871, "数组"=w1849, "字符串"=w1873, "输出簇 2"=w1853, "Str引用句柄"=w1848) -> (reference out=w1870:refnum<vi>)  [unwired: 12 in, 1 out]
                    n1407 = Insert Into Array(array=w1852, new element=w1870) -> (w1851:refnum<vi>[])  [unwired: 1 in]
                    n1408 = property on="数组 6" class="Arr (严格)"("Value"=w1851) -> ()  [unwired: 2 in, 2 out]
                  }
                  frame "开始测量 4" {
                    # "\\pem\\电源函数\\输出调用01.vi"
                    n1409 = control-ref of="水质4"() -> (w1892:refnum<vi>)
                    n1410 = control-ref of="温度4"() -> (w1891:refnum<vi>)
                    n1411 = control-ref of="温度显示 4"() -> (w1890:refnum<vi>)
                    n1412 = control-ref of="所有数据4"() -> (w1889:refnum<vi>)
                    n1413 = control-ref of="数值 4"() -> (w1888:refnum<vi>)
                    n1414 = control-ref of="极化曲线4"() -> (w1887:refnum<vi>)
                    n1415 = control-ref of="极化电压4"() -> (w1886:refnum<vi>)
                    n1416 = control-ref of="极化电流4"() -> (w1885:refnum<vi>)
                    n1417 = control-ref of="电压4"() -> (w1884:refnum<vi>)
                    n1418 = control-ref of="电流4"() -> (w1883:refnum<vi>)
                    n1419 = property on="用户：" class="Str"() -> ("Value"=w1894:string)  [unwired: 2 in, 2 out]
                    n1420 = property on="测试类型 2" class="Str"() -> ("Value"=w1893:string)  [unwired: 2 in, 2 out]
                    n1421 = property on="数组 12" class="Arr (严格)"() -> ("Value"=w1878:string[][])  [unwired: 2 in, 2 out]
                    n1422 = Bundle By Name(cluster=cluster{"用户名":string, "项目名称":string} {"用户名"="", "项目名称"=""}, "用户名"=w1894, "项目名称"=w1893) -> (w1900:cluster{"用户名":string, "项目名称":string})
                    n1423 = call <vilib>:"Application Directory.vi"() -> ("Application Directory"=w1876:path)
                    n1424 = Build Path(base path=w1876, name or relative path="pem\\电源函数\\输出调用04.vi") -> (appended path=w1874:path)
                    n1425 = control-ref of="压力4"() -> (w1879:refnum<vi>)
                    n1426 = Bundle By Name(cluster=T19 {"水质4"=refnum, "温度4"=refnum, "温度显示 4"=refnum, "所有数据4"=refnum, "数值 4"=refnum, "极化曲线4"=refnum, "极化电压4"=refnum, "极化电流4"=refnum, "电压4"=refnum, "电流4"=refnum, "压力4"=refnum}, "水质4"=w1892, "温度4"=w1891, "温度显示 4"=w1890, "所有数据4"=w1889, "数值 4"=w1888, "极化曲线4"=w1887, "极化电压4"=w1886, "极化电流4"=w1885, "电压4"=w1884, "电流4"=w1883, "压力4"=w1879) -> (w1882:T19)
                    n1427 = Open VI Reference(type specifier VI Refnum (for type only)=refnum<vi> refnum ("类型说明符VI引用句柄（仅用于类型）"), vi path=w1874, options=128 ("选项")) -> (vi reference=w1901:refnum<vi>)  [unwired: 3 in, 1 out]
                    n1428 = control-ref of="字符串 7"() -> (w1877:refnum<vi>)
                    n1429 = property on="VISA resource name 3" class="VISAName"() -> ("Value"=w1902:refnum<visa-resource-name>)  [unwired: 2 in, 2 out]
                    n1430 = property on="数组 7" class="Arr (严格)"() -> ("Value"=w1881:refnum<vi>[])  [unwired: 2 in, 2 out]
                    n1431 = call-by-ref "开始异步调用"(reference=w1901, "输出簇"=w1900, "数组"=w1878, "字符串"=w1902, "输出簇 2"=w1882, "Str引用句柄"=w1877) -> (reference out=w1899:refnum<vi>)  [unwired: 12 in, 1 out]
                    n1432 = Insert Into Array(array=w1881, new element=w1899) -> (w1880:refnum<vi>[])  [unwired: 1 in]
                    n1433 = property on="数组 7" class="Arr (严格)"("Value"=w1880) -> ()  [unwired: 2 in, 2 out]
                  }
                }
              }
            }
          }
          frame "耐久性曲线" {
            n1434 = case shown="真" w1904 {
              tunnel: w1903 -> [w1905 w1911]
              frame False {
                n1435 = case shown="\"开始测量\", 默认" w1905 {
                  frame "开始测量", Default {
                    n1436 = flat-sequence {
                      frame #0 {
                        n1437 = property on="数组 4" class="Arr (严格)"() -> ("Value"=w1906:refnum<vi>[])  [unwired: 2 in, 2 out]
                        n1438 = for {
                          tunnel: w1906 -> [w1909] mode=indexing
                          n1439 = invoke class="VI" method="Abort VI"(reference=w1909) -> (reference out=w1908:refnum<vi>)  [unwired: 2 in, 2 out]
                          n1440 = invoke class="VI" method="FP.Close"(reference=w1908) -> (reference out=w1907:refnum<vi>)  [unwired: 2 in, 2 out]
                          n1441 = Close Reference(reference=w1907) -> ()  [unwired: 1 in, 1 out]
                        }
                      }
                      frame #1 {
                        n1442 = property on="数组 4" class="Arr (严格)"("Value"=refnum<vi>[] [] ("数组 9")) -> ()  [unwired: 2 in, 2 out]
                      }
                    }
                  }
                  frame "开始测量 2" {
                  }
                  frame "开始测量 3" {
                  }
                  frame "开始测量 4" {
                  }
                }
              }
              frame True {
                n1443 = case shown="\"开始测量\", 默认" w1911 {
                  frame "开始测量", Default {
                    w1921 = "USB0::0x2EC7::0x3000::803489033757710017::INSTR"  # 用户名
                    n1444 = property on="施加电流(A):" class="DigNum (严格)"() -> ("Value"=w1924:dbl)  [unwired: 2 in, 2 out]
                    n1445 = property on="测试时长(H):" class="DigNum (严格)"() -> ("Value"=w1923:dbl)  [unwired: 2 in, 2 out]
                    n1446 = control-ref of="电压1"() -> (w1914:refnum<vi>)
                    n1447 = control-ref of="电流1"() -> (w1913:refnum<vi>)
                    n1448 = Bundle By Name(cluster=cluster{"电压1":refnum<vi>, "电流1":refnum<vi>} {"电压1"=refnum, "电流1"=refnum}, "电压1"=w1914, "电流1"=w1913) -> (w1912:cluster{"电压1":refnum<vi>, "电流1":refnum<vi>})
                    n1449 = Open VI Reference(type specifier VI Refnum (for type only)=refnum<vi> refnum ("类型说明符VI引用句柄（仅用于类型）"), vi path=path "C:/Users/526computer/Desktop/2022 - 副本/pem/电源函数/耐久性测试输出调用01.vi" ("VI路径"), options=128 ("选项")) -> (vi reference=w1925:refnum<vi>)  [unwired: 3 in, 1 out]
                    n1450 = call-by-ref "开始异步调用"(reference=w1925, "电流"=w1924, "时长"=w1923, "字符串"=w1921, "输出簇"=w1912) -> (reference out=w1922:refnum<vi>)  [unwired: 13 in, 1 out]
                    n1451 = property on="数组 4" class="Arr (严格)"() -> ("Value"=w1916:refnum<vi>[])  [unwired: 2 in, 2 out]
                    n1452 = Insert Into Array(array=w1916, new element=w1922) -> (w1917:refnum<vi>[])  [unwired: 1 in]
                    n1453 = property on="数组 4" class="Arr (严格)"("Value"=w1917) -> ()  [unwired: 2 in, 2 out]
                  }
                  frame "开始测量 2" {
                  }
                  frame "开始测量 3" {
                  }
                  frame "开始测量 4" {
                  }
                }
              }
            }
          }
          frame "线性扫描" {
          }
        }
      }
      event "测试项目": Value Change {
        n1454 = event-data() -> ("NewVal"=w1926:enum32{"EIS", "极化曲线", "耐久性曲线", "线性扫描"})  [unwired: 1 in, 5 out]
        n1455 = case shown="\"EIS\", 默认" w1926 {
          frame "EIS", Default {
            n1456 = flat-sequence {
              frame #0 {
                n1457 = property on="测试项目 2" class="TabCtl (严格)"("Value"=enum32{"极化曲线", "耐久性测试", "EIS"}."EIS" ("测试项目 2")) -> ()  [unwired: 2 in, 2 out]
              }
              frame #1 {
                w1928 = T4."Disabled and Grayed Out" ("禁用")
                n1458 = property on="连接" class="Bool (严格)"("DisabledEnum"=w1928) -> ()  [unwired: 2 in, 2 out]
                n1459 = property on="保存所有" class="Bool (严格)"("DisabledEnum"=w1928) -> ()  [unwired: 2 in, 2 out]
                n1460 = property on="配置" class="Bool (严格)"("DisabledEnum"=w1928) -> ()  [unwired: 2 in, 2 out]
                n1461 = property on="分析" class="Bool (严格)"("DisabledEnum"=w1928) -> ()  [unwired: 2 in, 2 out]
                n1462 = property on="3" class="Bool (严格)"("DisabledEnum"=w1928) -> ()  [unwired: 2 in, 2 out]
                n1463 = property on="4" class="Bool (严格)"("DisabledEnum"=w1928) -> ()  [unwired: 2 in, 2 out]
                n1464 = property on="2" class="Bool (严格)"("DisabledEnum"=w1928) -> ()  [unwired: 2 in, 2 out]
                n1465 = property on="通道选择" class="RadioBtnsControl (严格)"("DisabledEnum"=w1928) -> ()  [unwired: 2 in, 2 out]
              }
            }
          }
          frame "极化曲线" {
            n1466 = flat-sequence {
              frame #0 {
                n1467 = property on="测试项目 2" class="TabCtl (严格)"("Value"=enum32{"极化曲线", "耐久性测试"}."极化曲线" ("测试项目 2")) -> ()  [unwired: 2 in, 2 out]
              }
              frame #1 {
                w1930 = T4."Enabled" ("禁用")
                n1468 = property on="连接" class="Bool (严格)"("DisabledEnum"=w1930) -> ()  [unwired: 2 in, 2 out]
                n1469 = property on="保存所有" class="Bool (严格)"("DisabledEnum"=w1930) -> ()  [unwired: 2 in, 2 out]
                n1470 = property on="配置" class="Bool (严格)"("DisabledEnum"=w1930) -> ()  [unwired: 2 in, 2 out]
                n1471 = property on="分析" class="Bool (严格)"("DisabledEnum"=w1930) -> ()  [unwired: 2 in, 2 out]
                n1472 = property on="3" class="Bool (严格)"("DisabledEnum"=w1930) -> ()  [unwired: 2 in, 2 out]
                n1473 = property on="4" class="Bool (严格)"("DisabledEnum"=w1930) -> ()  [unwired: 2 in, 2 out]
                n1474 = property on="2" class="Bool (严格)"("DisabledEnum"=w1930) -> ()  [unwired: 2 in, 2 out]
                n1475 = property on="通道选择" class="RadioBtnsControl (严格)"("DisabledEnum"=w1930) -> ()  [unwired: 2 in, 2 out]
              }
            }
          }
          frame "耐久性曲线" {
            n1476 = flat-sequence {
              frame #0 {
                n1477 = property on="测试项目 2" class="TabCtl (严格)"("Value"=enum32{"极化曲线", "耐久性测试"}."耐久性测试" ("测试项目 2")) -> ()  [unwired: 2 in, 2 out]
              }
              frame #1 {
                w1932 = T4."Enabled" ("禁用")
                n1478 = property on="连接" class="Bool (严格)"("DisabledEnum"=w1932) -> ()  [unwired: 2 in, 2 out]
                n1479 = property on="保存所有" class="Bool (严格)"("DisabledEnum"=w1932) -> ()  [unwired: 2 in, 2 out]
                n1480 = property on="配置" class="Bool (严格)"("DisabledEnum"=w1932) -> ()  [unwired: 2 in, 2 out]
                n1481 = property on="分析" class="Bool (严格)"("DisabledEnum"=w1932) -> ()  [unwired: 2 in, 2 out]
                n1482 = property on="3" class="Bool (严格)"("DisabledEnum"=w1932) -> ()  [unwired: 2 in, 2 out]
                n1483 = property on="4" class="Bool (严格)"("DisabledEnum"=w1932) -> ()  [unwired: 2 in, 2 out]
                n1484 = property on="2" class="Bool (严格)"("DisabledEnum"=w1932) -> ()  [unwired: 2 in, 2 out]
                n1485 = property on="通道选择" class="RadioBtnsControl (严格)"("DisabledEnum"=w1932) -> ()  [unwired: 2 in, 2 out]
              }
            }
          }
        }
      }
      event "重排所有视图": Value Change {
        n1486 = event-data() -> ()  [unwired: 1 in, 6 out]
        n1487 = stacked-sequence {
          frame #0 {
            (unwired) FALSE
            n1488 = disable-structure shown="禁用" {
              frame Disabled {
                n1489 = for {
                  tunnel: "数组 3" -> [w2073] mode=indexing
                  n1490 = property class="VI"(reference=w2073) -> (reference out=w2070:refnum<vi>, "Front Panel.Title"=w2074:string)  [unwired: 1 in, 1 out]
                  n1491 = Wait (ms)(milliseconds to wait=u32 100 ("等待时间（毫秒）")) -> ()  [unwired: 1 out]
                  n1492 = flat-sequence {
                    tunnel: w2074 -> [w2077]
                    tunnel: [w2077] -> w2071
                    tunnel: w2070 -> [w2076]
                    tunnel: w2071 -> [w2086]
                    frame #0 {
                      n1493 = property class="VI"(reference=w2076, "FP.State"=T15."Standard" ("前面板窗口:状态")) -> ()  [unwired: 1 in, 2 out]
                    }
                    frame #1 {
                      n1494 = case shown="\"压力\"" w2086 {
                        tunnel: ["" ("winname") "极化曲线" ("winname") "温度" ("winname") "水质" ("winname") "工步列表" ("winname") "压力" ("winname") "列表" ("winname")] -> w2084
                        tunnel: [_ 729 129 1310 129 732 129] -> w2082
                        tunnel: [_ 348 721 721 348 721 195] -> w2078
                        tunnel: [_ 1157 601 583 598 578 1760] -> w2079
                        tunnel: [_ 370 317 317 370 317 150] -> w2080
                        frame "假", Default {
                        }
                        frame "极化曲线" {
                        }
                        frame "温度" {
                        }
                        frame "水质" {
                        }
                        frame "工步列表" {
                        }
                        frame "压力" {
                          # "left:126,top:568,right:729,bottom:933"
                        }
                        frame "列表" {
                        }
                      }
                      n1495 = dll-call lib="PTH2Dabs CUsers526computerDesktop测试软件pemLABVIEW.dll" fn="findlabview"("lpcallsname"=0, "winname"=w2084, "layer"=-1, "x"=w2082, "y"=w2078, "cx"=w2079, "cy"=w2080, "flag"=4) -> ()  [unwired: 12 in, 2 out]
                    }
                    frame #2 {
                    }
                  }
                }
              }
              frame Enabled {
              }
            }
            n1496 = property on="数组 3" class="Arr (严格)"() -> ("Value"=w1933:refnum<vi>[])  [unwired: 2 in, 2 out]
            n1497 = for {
              tunnel: w1933 -> [w1935] mode=indexing
              n1498 = invoke class="VI" method="FP.Close"(reference=w1935) -> (reference out=w1934:refnum<vi>)  [unwired: 2 in, 2 out]
              n1499 = property class="VI"(reference=w1934) -> ("Front Panel.Title"=w1936:string)  [unwired: 1 in, 2 out]
              n1500 = case shown="\"列表\"" w1936 {
                tunnel: w1934 -> [_ w1940 w1962 w1981 w2003 w2025 w2047]
                frame "假", Default {
                }
                frame "压力" {
                  n1501 = property class="VI"(reference=w1940) -> (reference out=w1939:refnum<vi>, error out=w1937:errorcluster, "Exec.State"=w1938:T23)  [unwired: 1 in]
                  n1502 = case shown="\"Running\"" w1938 {
                    tunnel: w1939 -> [_ w1948 w1955 w1958]
                    tunnel: w1937 -> [w1941 w1945 w1952 w1957]
                    tunnel: [w1941 w1942 w1949 w1956] -> _
                    frame "Bad", Default {
                      # "VI包含错误并且无法执行。"
                    }
                    frame "Idle" {
                      # "VI位于内存中但没有运行"
                      n1503 = invoke class="VI" method="Run VI"(reference=w1948, error in=w1945, "Wait until done"=FALSE ("结束前等待"), "Auto Dispose Ref"=FALSE ("自动销毁引用")) -> (reference out=w1944:refnum<vi>, error out=w1943:errorcluster)  [unwired: 1 in, 3 out]
                      n1504 = invoke on="子面板4" class="SubPnl" method="Insert VI"(error in=w1943, "VI Ref"=w1944) -> (error out=w1942:errorcluster)  [unwired: 2 in, 3 out]
                    }
                    frame "Run top level" {
                      # "VI是活动层次结构中的顶层VI"
                      n1505 = property class="VI"(reference=w1955, error in=w1952, "FP.State"=T15."Closed" ("前面板窗口:状态")) -> (reference out=w1951:refnum<vi>, error out=w1953:errorcluster)
                      n1506 = call <vilib>:"Clear Errors.vi"("error in (no error)"=w1953) -> ("error out"=w1950:errorcluster)  [unwired: 5 in, 1 out]
                      n1507 = invoke on="子面板4" class="SubPnl" method="Insert VI"(error in=w1950, "VI Ref"=w1951) -> (error out=w1949:errorcluster)  [unwired: 2 in, 3 out]
                    }
                    frame "Running" {
                      # "VI已由一个或多个处于活动状态的顶层VI保留为执行"
                      n1508 = invoke on="子面板4" class="SubPnl" method="Insert VI"(error in=w1957, "VI Ref"=w1958) -> (error out=w1956:errorcluster)  [unwired: 2 in, 3 out]
                    }
                  }
                }
                frame "水质" {
                  n1509 = property class="VI"(reference=w1962) -> (reference out=w1959:refnum<vi>, error out=w1961:errorcluster, "Exec.State"=w1960:T23)  [unwired: 1 in]
                  n1510 = case shown="\"Running\"" w1960 {
                    tunnel: w1959 -> [_ w1970 w1977 w1980]
                    tunnel: w1961 -> [w1963 w1967 w1974 w1979]
                    tunnel: [w1963 w1964 w1971 w1978] -> _
                    frame "Bad", Default {
                      # "VI包含错误并且无法执行。"
                    }
                    frame "Idle" {
                      # "VI位于内存中但没有运行"
                      n1511 = invoke class="VI" method="Run VI"(reference=w1970, error in=w1967, "Wait until done"=FALSE ("结束前等待"), "Auto Dispose Ref"=FALSE ("自动销毁引用")) -> (reference out=w1966:refnum<vi>, error out=w1965:errorcluster)  [unwired: 1 in, 3 out]
                      n1512 = invoke on="子面板5" class="SubPnl" method="Insert VI"(error in=w1965, "VI Ref"=w1966) -> (error out=w1964:errorcluster)  [unwired: 2 in, 3 out]
                    }
                    frame "Run top level" {
                      # "VI是活动层次结构中的顶层VI"
                      n1513 = property class="VI"(reference=w1977, error in=w1974, "FP.State"=T15."Closed" ("前面板窗口:状态")) -> (reference out=w1973:refnum<vi>, error out=w1975:errorcluster)
                      n1514 = call <vilib>:"Clear Errors.vi"("error in (no error)"=w1975) -> ("error out"=w1972:errorcluster)  [unwired: 5 in, 1 out]
                      n1515 = invoke on="子面板5" class="SubPnl" method="Insert VI"(error in=w1972, "VI Ref"=w1973) -> (error out=w1971:errorcluster)  [unwired: 2 in, 3 out]
                    }
                    frame "Running" {
                      # "VI已由一个或多个处于活动状态的顶层VI保留为执行"
                      n1516 = invoke on="子面板5" class="SubPnl" method="Insert VI"(error in=w1979, "VI Ref"=w1980) -> (error out=w1978:errorcluster)  [unwired: 2 in, 3 out]
                    }
                  }
                }
                frame "温度" {
                  n1517 = property class="VI"(reference=w1981) -> (reference out=w1982:refnum<vi>, error out=w1984:errorcluster, "Exec.State"=w1983:T23)  [unwired: 1 in]
                  n1518 = case shown="\"Running\"" w1983 {
                    tunnel: w1982 -> [_ w1992 w1999 w2002]
                    tunnel: w1984 -> [w1985 w1989 w1996 w2001]
                    tunnel: [w1985 w1986 w1993 w2000] -> _
                    frame "Bad", Default {
                      # "VI包含错误并且无法执行。"
                    }
                    frame "Idle" {
                      # "VI位于内存中但没有运行"
                      n1519 = invoke class="VI" method="Run VI"(reference=w1992, error in=w1989, "Wait until done"=FALSE ("结束前等待"), "Auto Dispose Ref"=FALSE ("自动销毁引用")) -> (reference out=w1988:refnum<vi>, error out=w1987:errorcluster)  [unwired: 1 in, 3 out]
                      n1520 = invoke on="子面板3" class="SubPnl" method="Insert VI"(error in=w1987, "VI Ref"=w1988) -> (error out=w1986:errorcluster)  [unwired: 2 in, 3 out]
                    }
                    frame "Run top level" {
                      # "VI是活动层次结构中的顶层VI"
                      n1521 = property class="VI"(reference=w1999, error in=w1996, "FP.State"=T15."Closed" ("前面板窗口:状态")) -> (reference out=w1995:refnum<vi>, error out=w1997:errorcluster)
                      n1522 = call <vilib>:"Clear Errors.vi"("error in (no error)"=w1997) -> ("error out"=w1994:errorcluster)  [unwired: 5 in, 1 out]
                      n1523 = invoke on="子面板3" class="SubPnl" method="Insert VI"(error in=w1994, "VI Ref"=w1995) -> (error out=w1993:errorcluster)  [unwired: 2 in, 3 out]
                    }
                    frame "Running" {
                      # "VI已由一个或多个处于活动状态的顶层VI保留为执行"
                      n1524 = invoke on="子面板3" class="SubPnl" method="Insert VI"(error in=w2001, "VI Ref"=w2002) -> (error out=w2000:errorcluster)  [unwired: 2 in, 3 out]
                    }
                  }
                }
                frame "极化曲线" {
                  n1525 = property class="VI"(reference=w2003) -> (reference out=w2004:refnum<vi>, error out=w2006:errorcluster, "Exec.State"=w2005:T23)  [unwired: 1 in]
                  n1526 = case shown="\"Running\"" w2005 {
                    tunnel: w2004 -> [_ w2014 w2021 w2024]
                    tunnel: w2006 -> [w2007 w2011 w2018 w2023]
                    tunnel: [w2007 w2008 w2015 w2022] -> _
                    frame "Bad", Default {
                      # "VI包含错误并且无法执行。"
                    }
                    frame "Idle" {
                      # "VI位于内存中但没有运行"
                      n1527 = invoke class="VI" method="Run VI"(reference=w2014, error in=w2011, "Wait until done"=FALSE ("结束前等待"), "Auto Dispose Ref"=FALSE ("自动销毁引用")) -> (reference out=w2010:refnum<vi>, error out=w2009:errorcluster)  [unwired: 1 in, 3 out]
                      n1528 = invoke on="子面板2" class="SubPnl" method="Insert VI"(error in=w2009, "VI Ref"=w2010) -> (error out=w2008:errorcluster)  [unwired: 2 in, 3 out]
                    }
                    frame "Run top level" {
                      # "VI是活动层次结构中的顶层VI"
                      n1529 = property class="VI"(reference=w2021, error in=w2018, "FP.State"=T15."Closed" ("前面板窗口:状态")) -> (reference out=w2017:refnum<vi>, error out=w2019:errorcluster)
                      n1530 = call <vilib>:"Clear Errors.vi"("error in (no error)"=w2019) -> ("error out"=w2016:errorcluster)  [unwired: 5 in, 1 out]
                      n1531 = invoke on="子面板2" class="SubPnl" method="Insert VI"(error in=w2016, "VI Ref"=w2017) -> (error out=w2015:errorcluster)  [unwired: 2 in, 3 out]
                    }
                    frame "Running" {
                      # "VI已由一个或多个处于活动状态的顶层VI保留为执行"
                      n1532 = invoke on="子面板2" class="SubPnl" method="Insert VI"(error in=w2023, "VI Ref"=w2024) -> (error out=w2022:errorcluster)  [unwired: 2 in, 3 out]
                    }
                  }
                }
                frame "工步列表" {
                  n1533 = property class="VI"(reference=w2025) -> (reference out=w2026:refnum<vi>, error out=w2028:errorcluster, "Exec.State"=w2027:T23)  [unwired: 1 in]
                  n1534 = case shown="\"Run top level\"" w2027 {
                    tunnel: w2026 -> [_ w2036 w2043 w2046]
                    tunnel: w2028 -> [w2029 w2033 w2040 w2045]
                    tunnel: [w2029 w2030 w2037 w2044] -> _
                    frame "Bad", Default {
                      # "VI包含错误并且无法执行。"
                    }
                    frame "Idle" {
                      # "VI位于内存中但没有运行"
                      n1535 = invoke class="VI" method="Run VI"(reference=w2036, error in=w2033, "Wait until done"=FALSE ("结束前等待"), "Auto Dispose Ref"=FALSE ("自动销毁引用")) -> (reference out=w2032:refnum<vi>, error out=w2031:errorcluster)  [unwired: 1 in, 3 out]
                      n1536 = invoke on="子面板1" class="SubPnl" method="Insert VI"(error in=w2031, "VI Ref"=w2032) -> (error out=w2030:errorcluster)  [unwired: 2 in, 3 out]
                    }
                    frame "Run top level" {
                      # "VI是活动层次结构中的顶层VI"
                      n1537 = property class="VI"(reference=w2043, error in=w2040, "FP.State"=T15."Closed" ("前面板窗口:状态")) -> (reference out=w2039:refnum<vi>, error out=w2041:errorcluster)
                      n1538 = call <vilib>:"Clear Errors.vi"("error in (no error)"=w2041) -> ("error out"=w2038:errorcluster)  [unwired: 5 in, 1 out]
                      n1539 = invoke on="子面板1" class="SubPnl" method="Insert VI"(error in=w2038, "VI Ref"=w2039) -> (error out=w2037:errorcluster)  [unwired: 2 in, 3 out]
                    }
                    frame "Running" {
                      # "VI已由一个或多个处于活动状态的顶层VI保留为执行"
                      n1540 = invoke on="子面板1" class="SubPnl" method="Insert VI"(error in=w2045, "VI Ref"=w2046) -> (error out=w2044:errorcluster)  [unwired: 2 in, 3 out]
                    }
                  }
                }
                frame "列表" {
                  n1541 = property class="VI"(reference=w2047) -> (reference out=w2050:refnum<vi>, error out=w2048:errorcluster, "Exec.State"=w2049:T23)  [unwired: 1 in]
                  n1542 = case shown="\"Running\"" w2049 {
                    tunnel: w2050 -> [_ w2058 w2065 w2068]
                    tunnel: w2048 -> [w2051 w2055 w2062 w2067]
                    tunnel: [w2051 w2052 w2059 w2066] -> _
                    frame "Bad", Default {
                      # "VI包含错误并且无法执行。"
                    }
                    frame "Idle" {
                      # "VI位于内存中但没有运行"
                      n1543 = invoke class="VI" method="Run VI"(reference=w2058, error in=w2055, "Wait until done"=FALSE ("结束前等待"), "Auto Dispose Ref"=FALSE ("自动销毁引用")) -> (reference out=w2054:refnum<vi>, error out=w2053:errorcluster)  [unwired: 1 in, 3 out]
                      n1544 = invoke on="子面板" class="SubPnl" method="Insert VI"(error in=w2053, "VI Ref"=w2054) -> (error out=w2052:errorcluster)  [unwired: 2 in, 3 out]
                    }
                    frame "Run top level" {
                      # "VI是活动层次结构中的顶层VI"
                      n1545 = property class="VI"(reference=w2065, error in=w2062, "FP.State"=T15."Closed" ("前面板窗口:状态")) -> (reference out=w2061:refnum<vi>, error out=w2063:errorcluster)
                      n1546 = call <vilib>:"Clear Errors.vi"("error in (no error)"=w2063) -> ("error out"=w2060:errorcluster)  [unwired: 5 in, 1 out]
                      n1547 = invoke on="子面板" class="SubPnl" method="Insert VI"(error in=w2060, "VI Ref"=w2061) -> (error out=w2059:errorcluster)  [unwired: 2 in, 3 out]
                    }
                    frame "Running" {
                      # "VI已由一个或多个处于活动状态的顶层VI保留为执行"
                      n1548 = invoke on="子面板" class="SubPnl" method="Insert VI"(error in=w2067, "VI Ref"=w2068) -> (error out=w2066:errorcluster)  [unwired: 2 in, 3 out]
                    }
                  }
                }
              }
            }
          }
          frame #1 {
            n1549 = property on="重排所有视图" class="Bool (严格)"("Value"=FALSE ("重排所有视图")) -> ()  [unwired: 2 in, 2 out]
          }
        }
      }
      event "显示所有视图": Value Change {
        n1550 = event-data() -> ()  [unwired: 1 in, 6 out]
        n1551 = stacked-sequence {
          frame #0 {
            n1552 = property on="数组 3" class="Arr (严格)"() -> ("Value"=w2119:refnum<vi>[])  [unwired: 2 in, 2 out]
            n1553 = for {
              tunnel: w2119 -> [w2123] mode=indexing
              n1554 = property class="VI"(reference=w2123) -> ("Front Panel.Title"=w2122:string)  [unwired: 1 in, 2 out]
              n1555 = Equal?(x=w2122, y="工步列表") -> (x = y?=w2120:bool)
              n1556 = case shown="真" w2120 {
                tunnel: w2123 -> [_ w2125]
                frame False {
                }
                frame True {
                  n1557 = flat-sequence {
                    tunnel: w2125 -> [w2127]
                    tunnel: [w2127] -> w2124
                    tunnel: w2124 -> [w2128]
                    frame #0 {
                      n1558 = invoke class="VI" method="FP.Open"(reference=w2127, "State"=T15."Standard" ("状态")) -> ()  [unwired: 3 in, 5 out]
                    }
                    frame #1 {
                      n1559 = property class="VI"(reference=w2128, "Front Panel.PanelBounds"=T20 {"Left"=681, "Top"=371, "Right"=1260, "Bottom"=688} ("前面板窗口:前面板边界")) -> ()  [unwired: 1 in, 2 out]
                    }
                  }
                }
              }
            }
          }
          frame #1 {
            n1560 = property on="数组 3" class="Arr (严格)"() -> ("Value"=w2130:refnum<vi>[])  [unwired: 2 in, 2 out]
            n1561 = for {
              tunnel: w2130 -> [w2131] mode=indexing
              n1562 = property class="VI"(reference=w2131) -> ("Front Panel.Title"=w2134:string)  [unwired: 1 in, 2 out]
              n1563 = Equal?(x=w2134, y="列表") -> (x = y?=w2132:bool)
              n1564 = case shown="真" w2132 {
                tunnel: w2131 -> [_ w2136]
                frame False {
                }
                frame True {
                  n1565 = flat-sequence {
                    tunnel: w2136 -> [w2138]
                    tunnel: [w2137] -> w2135
                    tunnel: w2135 -> [w2140]
                    frame #0 {
                      n1566 = invoke class="VI" method="FP.Open"(reference=w2138, "State"=T15."Standard" ("状态")) -> (reference out=w2137:refnum<vi>)  [unwired: 3 in, 4 out]
                    }
                    frame #1 {
                      n1567 = property class="VI"(reference=w2140, "Front Panel.PanelBounds"=T20 {"Left"=691, "Top"=381, "Right"=1270, "Bottom"=698} ("前面板窗口:前面板边界")) -> ()  [unwired: 1 in, 2 out]
                    }
                  }
                }
              }
            }
          }
          frame #2 {
            n1568 = property on="数组 3" class="Arr (严格)"() -> ("Value"=w2142:refnum<vi>[])  [unwired: 2 in, 2 out]
            n1569 = for {
              tunnel: w2142 -> [w2143] mode=indexing
              n1570 = property class="VI"(reference=w2143) -> ("Front Panel.Title"=w2146:string)  [unwired: 1 in, 2 out]
              n1571 = Equal?(x=w2146, y="极化曲线") -> (x = y?=w2144:bool)
              n1572 = case shown="真" w2144 {
                tunnel: w2143 -> [_ w2148]
                frame False {
                }
                frame True {
                  n1573 = flat-sequence {
                    tunnel: w2148 -> [w2150]
                    tunnel: [w2149] -> w2147
                    tunnel: w2147 -> [w2152]
                    frame #0 {
                      n1574 = invoke class="VI" method="FP.Open"(reference=w2150, "State"=T15."Standard" ("状态")) -> (reference out=w2149:refnum<vi>)  [unwired: 3 in, 4 out]
                    }
                    frame #1 {
                      n1575 = property class="VI"(reference=w2152, "Front Panel.PanelBounds"=T20 {"Left"=701, "Top"=391, "Right"=1280, "Bottom"=708} ("前面板窗口:前面板边界")) -> ()  [unwired: 1 in, 2 out]
                    }
                  }
                }
              }
            }
          }
          frame #3 {
            n1576 = property on="数组 3" class="Arr (严格)"() -> ("Value"=w2154:refnum<vi>[])  [unwired: 2 in, 2 out]
            n1577 = for {
              tunnel: w2154 -> [w2155] mode=indexing
              n1578 = property class="VI"(reference=w2155) -> ("Front Panel.Title"=w2158:string)  [unwired: 1 in, 2 out]
              n1579 = Equal?(x=w2158, y="压力") -> (x = y?=w2156:bool)
              n1580 = case shown="真" w2156 {
                tunnel: w2155 -> [_ w2160]
                frame False {
                }
                frame True {
                  n1581 = flat-sequence {
                    tunnel: w2160 -> [w2162]
                    tunnel: [w2161] -> w2159
                    tunnel: w2159 -> [w2164]
                    frame #0 {
                      n1582 = invoke class="VI" method="FP.Open"(reference=w2162, "State"=T15."Standard" ("状态")) -> (reference out=w2161:refnum<vi>)  [unwired: 3 in, 4 out]
                    }
                    frame #1 {
                      n1583 = property class="VI"(reference=w2164, "Front Panel.PanelBounds"=T20 {"Left"=711, "Top"=401, "Right"=1290, "Bottom"=718} ("前面板窗口:前面板边界")) -> ()  [unwired: 1 in, 2 out]
                    }
                  }
                }
              }
            }
          }
          frame #4 {
            n1584 = property on="数组 3" class="Arr (严格)"() -> ("Value"=w2166:refnum<vi>[])  [unwired: 2 in, 2 out]
            n1585 = for {
              tunnel: w2166 -> [w2167] mode=indexing
              n1586 = property class="VI"(reference=w2167) -> ("Front Panel.Title"=w2170:string)  [unwired: 1 in, 2 out]
              n1587 = Equal?(x=w2170, y="温度") -> (x = y?=w2168:bool)
              n1588 = case shown="真" w2168 {
                tunnel: w2167 -> [_ w2172]
                frame False {
                }
                frame True {
                  n1589 = flat-sequence {
                    tunnel: w2172 -> [w2174]
                    tunnel: [w2173] -> w2171
                    tunnel: w2171 -> [w2176]
                    frame #0 {
                      n1590 = invoke class="VI" method="FP.Open"(reference=w2174, "State"=T15."Standard" ("状态")) -> (reference out=w2173:refnum<vi>)  [unwired: 3 in, 4 out]
                    }
                    frame #1 {
                      n1591 = property class="VI"(reference=w2176, "Front Panel.PanelBounds"=T20 {"Left"=722, "Top"=411, "Right"=1300, "Bottom"=728} ("前面板窗口:前面板边界")) -> ()  [unwired: 1 in, 2 out]
                    }
                  }
                }
              }
            }
          }
          frame #5 {
            n1592 = property on="数组 3" class="Arr (严格)"() -> ("Value"=w2178:refnum<vi>[])  [unwired: 2 in, 2 out]
            n1593 = for {
              tunnel: w2178 -> [w2179] mode=indexing
              n1594 = property class="VI"(reference=w2179) -> ("Front Panel.Title"=w2182:string)  [unwired: 1 in, 2 out]
              n1595 = Equal?(x=w2182, y="水质") -> (x = y?=w2180:bool)
              n1596 = case shown="真" w2180 {
                tunnel: w2179 -> [_ w2184]
                frame False {
                }
                frame True {
                  n1597 = flat-sequence {
                    tunnel: w2184 -> [w2186]
                    tunnel: [w2185] -> w2183
                    tunnel: w2183 -> [w2188]
                    frame #0 {
                      n1598 = invoke class="VI" method="FP.Open"(reference=w2186, "State"=T15."Standard" ("状态")) -> (reference out=w2185:refnum<vi>)  [unwired: 3 in, 4 out]
                    }
                    frame #1 {
                      n1599 = property class="VI"(reference=w2188, "Front Panel.PanelBounds"=T20 {"Left"=732, "Top"=421, "Right"=1310, "Bottom"=738} ("前面板窗口:前面板边界")) -> ()  [unwired: 1 in, 2 out]
                    }
                  }
                }
              }
            }
          }
          frame #6 {
            n1600 = property on="显示所有视图" class="Bool (严格)"("Value"=FALSE ("显示所有视图")) -> ()  [unwired: 2 in, 2 out]
          }
        }
      }
      event "退出": Mouse Down {
        n1601 = event-data() -> ()  [unwired: 1 in, 8 out]
        n1602 = flat-sequence {
          tunnel: [w2205] -> w2192
          tunnel: w2192 -> [w2209]
          tunnel: [w2209] -> w2191
          tunnel: w2191 -> [w2211]
          frame #0 {
            n1603 = flat-sequence {
              frame #0 {
                n1604 = invoke on="子面板2" class="SubPnl" method="Remove VI"() -> ()  [unwired: 3 in, 3 out]
                n1605 = invoke on="子面板3" class="SubPnl" method="Remove VI"() -> ()  [unwired: 3 in, 3 out]
                n1606 = invoke on="子面板4" class="SubPnl" method="Remove VI"() -> ()  [unwired: 3 in, 3 out]
                n1607 = invoke on="子面板1" class="SubPnl" method="Remove VI"() -> ()  [unwired: 3 in, 3 out]
                n1608 = invoke on="子面板5" class="SubPnl" method="Remove VI"() -> ()  [unwired: 3 in, 3 out]
                n1609 = invoke on="子面板10" class="SubPnl" method="Remove VI"() -> ()  [unwired: 3 in, 3 out]
                n1610 = invoke on="子面板" class="SubPnl" method="Remove VI"() -> ()  [unwired: 3 in, 3 out]
                n1611 = invoke on="子面板6" class="SubPnl" method="Remove VI"() -> ()  [unwired: 3 in, 3 out]
              }
            }
          }
          frame #1 {
            n1612 = property on="数组 4" class="Arr (严格)"() -> ("Value"=w2196:refnum<vi>[])  [unwired: 2 in, 2 out]
            n1613 = property on="数组 7" class="Arr (严格)"() -> ("Value"=w2193:refnum<vi>[])  [unwired: 2 in, 2 out]
            n1614 = for {
              tunnel: w2193 -> [w2198] mode=indexing
              n1615 = invoke class="VI" method="Abort VI"(reference=w2198) -> (reference out=w2197:refnum<vi>)  [unwired: 2 in, 2 out]
              n1616 = invoke class="VI" method="FP.Close"(reference=w2197) -> ()  [unwired: 2 in, 3 out]
            }
            n1617 = for {
              tunnel: w2196 -> [w2204] mode=indexing
              n1618 = invoke class="VI" method="Abort VI"(reference=w2204) -> (reference out=w2203:refnum<vi>)  [unwired: 2 in, 2 out]
              n1619 = invoke class="VI" method="FP.Close"(reference=w2203) -> ()  [unwired: 2 in, 3 out]
            }
            n1620 = property on="数组 6" class="Arr (严格)"() -> ("Value"=w2194:refnum<vi>[])  [unwired: 2 in, 2 out]
            n1621 = property on="数组 5" class="Arr (严格)"() -> ("Value"=w2195:refnum<vi>[])  [unwired: 2 in, 2 out]
            n1622 = for {
              tunnel: w2195 -> [w2202] mode=indexing
              n1623 = invoke class="VI" method="Abort VI"(reference=w2202) -> (reference out=w2201:refnum<vi>)  [unwired: 2 in, 2 out]
              n1624 = invoke class="VI" method="FP.Close"(reference=w2201) -> ()  [unwired: 2 in, 3 out]
            }
            n1625 = for {
              tunnel: w2194 -> [w2200] mode=indexing
              n1626 = invoke class="VI" method="Abort VI"(reference=w2200) -> (reference out=w2199:refnum<vi>)  [unwired: 2 in, 2 out]
              n1627 = invoke class="VI" method="FP.Close"(reference=w2199) -> ()  [unwired: 2 in, 3 out]
            }
          }
          frame #2 {
            n1628 = property on="数组 3" class="Arr (严格)"() -> ("Value"=w2205:refnum<vi>[])  [unwired: 2 in, 2 out]
            n1629 = for {
              tunnel: w2205 -> [w2208] mode=indexing
              n1630 = invoke class="VI" method="FP.Open"(reference=w2208, "State"=T15."Standard" ("状态")) -> (reference out=w2207:refnum<vi>)  [unwired: 3 in, 4 out]
              n1631 = invoke class="VI" method="Abort VI"(reference=w2207) -> ()  [unwired: 2 in, 3 out]
            }
          }
          frame #3 {
            n1632 = for {
              tunnel: w2209 -> [w2210] mode=indexing
              n1633 = invoke class="VI" method="FP.Close"(reference=w2210) -> ()  [unwired: 2 in, 3 out]
            }
          }
          frame #4 {
            n1634 = for {
              tunnel: w2211 -> [w2212] mode=indexing
              n1635 = Close Reference(reference=w2212) -> ()  [unwired: 1 in, 1 out]
            }
          }
          frame #5 {
            n1636 = Stop(stop? (T)=TRUE ("停止？(T)")) -> ()
          }
        }
      }
      event "通道选择 2": Value Change {
        n1637 = event-data() -> ("NewVal"=w2214:enum32{"未选择", "A1", "A2", "A3", "A4"})  [unwired: 1 in, 5 out]
        n1638 = case shown="\"A1\", 默认" w2214 {
          frame "A1", Default {
            n1639 = property on="开始测量 4" class="Bool (严格)"("Visible"=FALSE ("可见")) -> ()  [unwired: 2 in, 2 out]
            n1640 = property on="开始测量 3" class="Bool (严格)"("Visible"=FALSE ("可见")) -> ()  [unwired: 2 in, 2 out]
            n1641 = property on="开始测量" class="Bool (严格)"("Visible"=TRUE ("可见")) -> ()  [unwired: 2 in, 2 out]
            n1642 = property on="开始测量 2" class="Bool (严格)"("Visible"=FALSE ("可见")) -> ()  [unwired: 2 in, 2 out]
          }
          frame "A2" {
            n1643 = property on="开始测量 4" class="Bool (严格)"("Visible"=FALSE ("可见")) -> ()  [unwired: 2 in, 2 out]
            n1644 = property on="开始测量 3" class="Bool (严格)"("Visible"=FALSE ("可见")) -> ()  [unwired: 2 in, 2 out]
            n1645 = property on="开始测量" class="Bool (严格)"("Visible"=FALSE ("可见")) -> ()  [unwired: 2 in, 2 out]
            n1646 = property on="开始测量 2" class="Bool (严格)"("Visible"=TRUE ("可见")) -> ()  [unwired: 2 in, 2 out]
          }
          frame "A3" {
            n1647 = property on="开始测量 4" class="Bool (严格)"("Visible"=FALSE ("可见")) -> ()  [unwired: 2 in, 2 out]
            n1648 = property on="开始测量 3" class="Bool (严格)"("Visible"=TRUE ("可见")) -> ()  [unwired: 2 in, 2 out]
            n1649 = property on="开始测量" class="Bool (严格)"("Visible"=FALSE ("可见")) -> ()  [unwired: 2 in, 2 out]
            n1650 = property on="开始测量 2" class="Bool (严格)"("Visible"=FALSE ("可见")) -> ()  [unwired: 2 in, 2 out]
          }
          frame "A4" {
            n1651 = property on="开始测量 4" class="Bool (严格)"("Visible"=TRUE ("可见")) -> ()  [unwired: 2 in, 2 out]
            n1652 = property on="开始测量 3" class="Bool (严格)"("Visible"=FALSE ("可见")) -> ()  [unwired: 2 in, 2 out]
            n1653 = property on="开始测量" class="Bool (严格)"("Visible"=FALSE ("可见")) -> ()  [unwired: 2 in, 2 out]
            n1654 = property on="开始测量 2" class="Bool (严格)"("Visible"=FALSE ("可见")) -> ()  [unwired: 2 in, 2 out]
          }
        }
      }
      event "历史曲线": Value Change {
        n1655 = event-data() -> ()  [unwired: 1 in, 6 out]
        n1656 = Current VI's Path() -> (path=w2238:path)
        n1657 = Strip Path(path=w2238) -> (stripped path=w2239:path)  [unwired: 1 out]
        n1658 = Build Path(base path=w2239, name or relative path=path "TEMPDATA" ("名称或相对路径")) -> (appended path=w2240:path)
        n1659 = call "文件对话框4"("start path"=w2240) -> ("selected path"=w2236:path, "error out"=w2232:errorcluster)  [unwired: 11 in, 2 out]
        n1660 = Build Path(base path=w2236, name or relative path=path "索引.txt" ("名称或相对路径")) -> (appended path=w2234:path)
        n1661 = Open/Create/Replace File(file path (use dialog)=w2234, error in=w2232, operation (0:open)=T21."open" ("操作(0:open)")) -> (refnum out=w2242:refnum<file>, error out=w2241:errorcluster)  [unwired: 3 in, 1 out]
        n1662 = Unbundle(w2241) -> ("status"=w2231:bool)  [unwired: 2 out]
        n1663 = case shown="假" w2231 {
          tunnel: w2242 -> [w2244 _]
          tunnel: w2241 -> [w2243 _]
          frame False {
            n1664 = disable-structure shown="禁用" {
              disable-tunnel: w2244 -> [w2246 _]
              disable-tunnel: w2243 -> [w2245 _]
              frame Disabled {
                n1665 = flat-sequence {
                  tunnel: w2245 -> [w2252]
                  tunnel: w2246 -> [w2253]
                  tunnel: [w2253] -> w2250
                  tunnel: [w2252] -> w2249
                  tunnel: [w2256] -> w2248
                  tunnel: [w2255] -> w2247
                  tunnel: w2250 -> [w2265]
                  tunnel: w2249 -> [w2264]
                  tunnel: w2248 -> [w2287]
                  tunnel: w2247 -> [w2288]
                  frame #0 {
                    w2251 = cluster{dbl[], dbl[]} {[], []} ("XY图 2")
                  }
                  frame #1 {
                    n1666 = while {
                      tunnel: w2265 -> [w2279]
                      tunnel: w2264 -> [w2278]
                      tunnel: [w2271] -> w2254 mode=indexing
                      tunnel: [w2270] -> w2260
                      stop <- w2268 stop-if-true
                      n1667 = Read from Text File(file (use dialog)=w2279, count=1 ("计数"), error in=w2278) -> (refnum out=w2270:refnum<file>, text=w2275:string[], error out=w2276:errorcluster)  [unwired: 1 in, 1 out]
                      n1668 = Unbundle(w2276) -> ("status"=w2269:bool)  [unwired: 2 out]
                      n1669 = Index Array(array=w2275, index=0 ("索引")) -> (element=w2272:string)
                      n1670 = Not Equal?(x=w2272, y="") -> (x != y?=w2267:bool)
                      n1671 = case shown="假" w2267 {
                        tunnel: w2272 -> [_ w2283]
                        tunnel: [0 w2281] -> w2271
                        frame False {
                        }
                        frame True {
                          n1672 = Scan From String(format string="%d" ("格式字符串"), input string=w2283) -> (output 1=w2281:i32)  [unwired: 3 in, 3 out]
                        }
                      }
                      n1673 = Not(x=w2267) -> (.not. x?=w2266:bool)
                      n1674 = Or(x=w2266, y=w2269) -> (x .or. y?=w2268:bool)
                    }
                    n1675 = Array Size(array=w2254) -> (size(s)=w2263:i32)
                    n1676 = Close File(refnum=w2260) -> (path=w2259:path)  [unwired: 1 in, 1 out]
                    n1677 = Decrement(x=w2263) -> (x-1=w2261:i32)
                    n1678 = Strip Path(path=w2259) -> (stripped path=w2258:path)  [unwired: 1 out]
                    n1679 = Build Path(base path=w2258, name or relative path=path "数据.txt" ("名称或相对路径")) -> (appended path=w2256:path)
                    n1680 = Delete From Array(array=w2254, length=1 ("长度"), index=w2261) -> (array with subset deleted=w2255:i32[])  [unwired: 1 out]
                  }
                  frame #2 {
                    n1681 = Open/Create/Replace File(file path (use dialog)=w2287, operation (0:open)=T21."open" ("操作(0:open)")) -> (refnum out=w2290:refnum<file>, error out=w2291:errorcluster)  [unwired: 4 in, 1 out]
                    n1682 = for {
                      tunnel: w2290 -> [w2308]
                      tunnel: w2291 -> [w2307]
                      tunnel: [w2302] -> _
                      tunnel: [w2301] -> _
                      tunnel: [w2296] -> w2286 mode=indexing
                      tunnel: [w2295] -> w2285 mode=indexing
                      tunnel: w2288 -> [w2294] mode=indexing
                      n1683 = Decrement(x=w2294) -> (x-1=w2300:i32)
                      n1684 = Read from Text File(file (use dialog)=w2308, count=w2294, error in=w2307) -> (refnum out=w2306:refnum<file>, text=w2293:string[], error out=w2305:errorcluster)  [unwired: 1 in, 1 out]
                      n1685 = Index Array(array=w2293, index=w2300) -> (element=w2292:string)
                      n1686 = Set File Position(offset (in bytes) (0)=i64 0 ("偏移量（字节）（0）"), refnum=w2306, from (0:start)=enum16{"start", "end", "current"}."start" ("自（0:起始）"), error in=w2305) -> (refnum out=w2302:refnum<file>, error out=w2301:errorcluster)
                      n1687 = Search/Split String(string=w2292, search string/char (-)="电流" ("搜索字符串/字符(-)")) -> (match + rest of string=w2298:string)  [unwired: 1 in, 2 out]
                      n1688 = Scan From String(format string="电流：%f 电压：%f" ("格式字符串"), input string=w2298) -> (output 1=w2296:dbl, output 2=w2295:dbl)  [unwired: 4 in, 3 out]
                    }
                    n1689 = Bundle(w2286, w2285) -> (w2284:cluster{dbl[], dbl[]})  [unwired: 1 in]
                  }
                  frame #3 {
                  }
                }
              }
              frame Enabled {
              }
            }
          }
          frame True {
          }
        }
      }
      event "导出曲线": Value Change {
        n1690 = event-data() -> ("NewVal"=w2309:bool)  [unwired: 1 in, 5 out]
        n1691 = property on="新值" class="Bool (严格)"("Val(Sgnl)"=w2309) -> ()  [unwired: 2 in, 2 out]
      }
      event "保存当前设置", "打开历史设置", "撤销当前设置": Value Change {
        n1692 = event-data() -> ("CtlRef"=w2311:refnum<vi>)  [unwired: 1 in, 3 out]
        n1693 = property class="Bool"(reference=w2311) -> ("BoolText.Text"=w2310:string)  [unwired: 1 in, 2 out]
        n1694 = property on="队列输出 2" class="TypRef (严格)" props=["Value"]() -> ()  [unwired: 2 in, 3 out]
        n1695 = case shown="\"保存设置\"" w2310 {
          frame "假", Default {
          }
          frame "保存设置" {
            n1696 = case shown="\"ALL\"" "通道选择" {
              selector: "通道选择" -> [_ w2368]
              frame "ALL" {
                n1697 = Current VI's Path() -> (path=w2326:path)
                n1698 = Strip Path(path=w2326) -> (stripped path=w2325:path)  [unwired: 1 out]
                n1699 = String To Path(string="设置文件") -> (path=w2324:path)
                n1700 = Build Path(base path=w2325, name or relative path=w2324) -> (appended path=w2323:path)
                n1701 = call "文件对话框"("start path"=w2323, "default name"="配置文件", "pattern (all files)"="*.ini", "pattern label"="类型文件") -> ("selected path"=w2322:path, "error out"=w2316:errorcluster)  [unwired: 8 in, 2 out]
                n1702 = call <vilib>:"Open Config Data.vi"("create file if necessary (T)"=TRUE, "configuration file path"=w2322) -> ("error out"=w2313:errorcluster, "refnum"=w2314:T25)  [unwired: 7 in, 1 out]
                n1703 = Unbundle By Name(w2316) -> ("status"=w2315:bool)
                n1704 = case shown="假" w2315 {
                  tunnel: w2314 -> [w2328 _]
                  tunnel: w2313 -> [w2327 _]
                  frame False {
                    n1705 = flat-sequence {
                      tunnel: [w2336] -> w2332
                      tunnel: [w2335] -> w2331
                      tunnel: w2328 -> [w2334]
                      tunnel: w2327 -> [w2333]
                      tunnel: w2332 -> [w2358]
                      tunnel: [w2353] -> w2330
                      tunnel: w2331 -> [w2357]
                      tunnel: [w2352] -> w2329
                      tunnel: w2330 -> [w2360]
                      tunnel: w2329 -> [w2359]
                      frame #0 {
                        n1706 = for {
                          tunnel: string[] ["A1", "A2", "A3", "A4"] -> [w2341] mode=indexing
                          tunnel: w2334 -> [w2340]
                          tunnel: w2333 -> [_]
                          tunnel: [w2339] -> w2336
                          tunnel: [w2338] -> w2335
                          i -> [w2342]
                          n1707 = property on="树形控件 2" class="Tree (严格)"() -> ("All Tags"=w2343:string[])  [unwired: 2 in, 2 out]
                          n1708 = for {
                            tunnel: w2343 -> [w2347] mode=indexing
                            tunnel: w2342 -> [w2350]
                            tunnel: w2341 -> [w2349]
                            tunnel: w2340 -> [w2348]
                            tunnel: [w2345] -> w2339
                            tunnel: [w2344] -> w2338
                            n1709 = Increment(x=w2350) -> (x+1=w2351:i32)
                            n1710 = property on="树形控件 2" class="Tree (严格)"("Active Item Tag"=w2347, "ActiveColNum"=w2351) -> ("Cell String"=w2346:string)  [unwired: 2 in, 2 out]
                            n1711 = call-poly <vilib>:"Write Key.vi"("section"=w2349, "value"=w2346, "key"=w2347, "refnum"=w2348) -> ("error out"=w2344:errorcluster, "refnum out"=w2345:T25)  [unwired: 5 in, 1 out]
                          }
                        }
                      }
                      frame #1 {
                        n1712 = call-poly <vilib>:"Write Key.vi"("section"="通道数量", "error in (no error)"=w2357, "value"="4", "key"="数量", "refnum"=w2358) -> ("error out"=w2352:errorcluster, "refnum out"=w2353:T25)  [unwired: 4 in, 1 out]
                      }
                      frame #2 {
                        n1713 = call <vilib>:"Close Config Data.vi"("error in (no error)"=w2359, "refnum"=w2360) -> ()  [unwired: 8 in, 2 out]
                      }
                    }
                  }
                  frame True {
                  }
                }
              }
              frame "A1", Default {
                n1714 = Current VI's Path() -> (path=w2382:path)
                n1715 = String To Path(string="设置文件") -> (path=w2380:path)
                n1716 = Strip Path(path=w2382) -> (stripped path=w2381:path)  [unwired: 1 out]
                n1717 = Build Path(base path=w2381, name or relative path=w2380) -> (appended path=w2379:path)
                n1718 = call "文件对话框2"("start path"=w2379, "default name"="配置文件", "pattern (all files)"="*.ini", "pattern label"="类型文件") -> ("selected path"=w2378:path)  [unwired: 8 in, 3 out]
                n1719 = property on="树形控件 2" class="Tree (严格)"() -> ("All Tags"=w2369:string[])  [unwired: 2 in, 2 out]
                n1720 = call <vilib>:"Open Config Data.vi"("create file if necessary (T)"=TRUE, "configuration file path"=w2378) -> ("error out"=w2371:errorcluster, "refnum"=w2372:T25)  [unwired: 7 in, 1 out]
                n1721 = for {
                  tunnel: w2372 -> [w2390]
                  tunnel: w2371 -> [w2389]
                  tunnel: "通道配置" -> [w2388]
                  tunnel: w2369 -> [w2386] mode=indexing
                  tunnel: w2368 -> [w2387]
                  tunnel: [w2384] -> w2364
                  tunnel: [w2383] -> w2363
                  n1722 = property on="树形控件 2" class="Tree (严格)"("Active Item Tag"=w2386, "ActiveColNum"=w2387) -> ("Cell String"=w2385:string)  [unwired: 2 in, 2 out]
                  n1723 = call-poly <vilib>:"Write Key.vi"("section"=w2388, "error in (no error)"=w2389, "value"=w2385, "key"=w2386, "refnum"=w2390) -> ("error out"=w2383:errorcluster, "refnum out"=w2384:T25)  [unwired: 4 in, 1 out]
                }
                n1724 = call-poly <vilib>:"Write Key.vi"("section"="通道数量", "error in (no error)"=w2363, "value"="1", "key"="数量", "refnum"=w2364) -> ("error out"=w2361:errorcluster, "refnum out"=w2362:T25)  [unwired: 4 in, 1 out]
                n1725 = call <vilib>:"Close Config Data.vi"("error in (no error)"=w2361, "refnum"=w2362) -> ()  [unwired: 8 in, 2 out]
              }
            }
          }
          frame "打开设置" {
            n1726 = Current VI's Path() -> (path=w2401:path)
            n1727 = String To Path(string="设置文件") -> (path=w2399:path)
            n1728 = Strip Path(path=w2401) -> (stripped path=w2400:path)  [unwired: 1 out]
            n1729 = Build Path(base path=w2400, name or relative path=w2399) -> (appended path=w2398:path)
            n1730 = call "文件对话框5"("start path"=w2398, "default name"="配置文件", "pattern (all files)"="*.ini", "pattern label"="类型文件") -> ("selected path"=w2397:path, "error out"=w2392:errorcluster)  [unwired: 8 in, 2 out]
            n1731 = Unbundle By Name(w2392) -> ("status"=w2391:bool)
            n1732 = case shown="假" w2391 {
              tunnel: w2397 -> [w2413 _]
              frame False {
                n1733 = property on="通道选择" class="RadioBtnsControl (严格)"() -> ("Value"=w2407:enum32{"ALL", "A1", "A2", "A3", "A4"})  [unwired: 2 in, 2 out]
                n1734 = case shown="\"ALL\"" w2407 {
                  tunnel: ["4" "1"] -> w2405
                  frame "ALL" {
                  }
                  frame "A1", Default {
                  }
                }
                n1735 = call <vilib>:"Open Config Data.vi"("create file if necessary (T)"=FALSE, "configuration file path"=w2413) -> ("error out"=w2410:errorcluster, "refnum"=w2411:T25)  [unwired: 7 in, 1 out]
                n1736 = call-poly <vilib>:"Read Key.vi"("section"="通道数量", "error in (no error)"=w2410, "key"="数量", "refnum"=w2411) -> ("error out"=w2402:errorcluster, "value"=w2406:string, "refnum out"=w2403:T25)  [unwired: 4 in, 1 out]
                n1737 = Equal?(x=w2406, y=w2405) -> (x = y?=w2404:bool)
                n1738 = case shown="真" w2404 {
                  tunnel: w2403 -> [_ w2419]
                  tunnel: w2402 -> [_ w2416]
                  frame False {
                    n1739 = One Button Dialog(message="配置文件通道数与通道选项不相等" ("消息"), button name ("OK")="确定" ("按钮名称（“确定”）")) -> ()  [unwired: 1 out]
                  }
                  frame True {
                    n1740 = flat-sequence {
                      tunnel: w2419 -> [w2422]
                      tunnel: [w2422] -> w2418
                      tunnel: [w2420] -> w2417
                      tunnel: w2418 -> [w2426]
                      tunnel: w2417 -> [w2427]
                      tunnel: w2416 -> [w2425]
                      frame #0 {
                        n1741 = property on="通道选择" class="RadioBtnsControl (严格)"() -> ("Value"=w2421:enum32{"ALL", "A1", "A2", "A3", "A4"})  [unwired: 2 in, 2 out]
                        n1742 = case shown="\"A1\", 默认" w2421 {
                          tunnel: ["ALL" "通道配置"] -> w2420
                          frame "ALL" {
                          }
                          frame "A1", Default {
                          }
                        }
                      }
                      frame #1 {
                        n1743 = flat-sequence {
                          tunnel: w2427 -> [w2432]
                          tunnel: w2426 -> [w2431]
                          tunnel: w2425 -> [w2430]
                          frame #0 {
                            n1744 = case shown="\"ALL\"" w2432 {
                              selector: w2432 -> [_ w2454]
                              tunnel: w2431 -> [w2435 w2456]
                              tunnel: [w2434 w2453] -> w2429
                              tunnel: [w2433 w2452] -> w2428
                              tunnel: w2430 -> [_ w2451]
                              frame "ALL" {
                                n1745 = for {
                                tunnel: string[] ["A1", "A2", "A3", "A4"] -> [w2440] mode=indexing
                                tunnel: w2435 -> [w2441]
                                tunnel: [w2438] -> w2434
                                tunnel: [w2437] -> w2433
                                i -> [w2439]
                                n1746 = property on="树形控件 2" class="Tree (严格)"() -> ("All Tags"=w2442:string[])  [unwired: 2 in, 2 out]
                                n1747 = for {
                                tunnel: w2442 -> [w2448] mode=indexing
                                tunnel: w2441 -> [w2450]
                                tunnel: w2440 -> [w2449]
                                tunnel: w2439 -> [w2446]
                                tunnel: [w2444] -> w2438
                                tunnel: [w2443] -> w2437
                                n1748 = call-poly <vilib>:"Read Key.vi"("section"=w2449, "key"=w2448, "refnum"=w2450) -> ("error out"=w2443:errorcluster, "value"=w2445:string, "refnum out"=w2444:T25)  [unwired: 5 in, 1 out]
                                n1749 = Increment(x=w2446) -> (x+1=w2447:i32)
                                n1750 = property on="树形控件 2" class="Tree (严格)"("Active Item Tag"=w2448, "ActiveColNum"=w2447, "Cell String"=w2445) -> ()  [unwired: 2 in, 2 out]
                                }
                                }
                              }
                              frame "A1", Default {
                                n1751 = property on="树形控件 2" class="Tree (严格)"() -> ("All Tags"=w2455:string[])  [unwired: 2 in, 2 out]
                                n1752 = for {
                                tunnel: w2456 -> [w2464]
                                tunnel: w2455 -> [w2462] mode=indexing
                                tunnel: w2454 -> [w2463]
                                tunnel: [w2459] -> w2453
                                tunnel: [w2458] -> w2452
                                tunnel: w2451 -> [w2457]
                                n1753 = call-poly <vilib>:"Read Key.vi"("section"=w2463, "error in (no error)"=w2457, "key"=w2462, "refnum"=w2464) -> ("error out"=w2458:errorcluster, "value"=w2460:string, "refnum out"=w2459:T25)  [unwired: 4 in, 1 out]
                                n1754 = property on="通道选择" class="RadioBtnsControl (严格)"() -> ("Value"=w2461:enum32{"ALL", "A1", "A2", "A3", "A4"})  [unwired: 2 in, 2 out]
                                n1755 = property on="树形控件 2" class="Tree (严格)"("Active Item Tag"=w2462, "ActiveColNum"=w2461, "Cell String"=w2460) -> ()  [unwired: 2 in, 2 out]
                                }
                              }
                            }
                            n1756 = call <vilib>:"Close Config Data.vi"("error in (no error)"=w2428, "refnum"=w2429) -> ()  [unwired: 8 in, 2 out]
                          }
                          frame #1 {
                            n1757 = property on="通道选择" class="RadioBtnsControl (严格)"() -> ("Value"=w2465:enum32{"ALL", "A1", "A2", "A3", "A4"})  [unwired: 2 in, 2 out]
                            n1758 = stacked-sequence {
                              seq-local: [w2467 _ _] -> [_ _ _]
                              tunnel: w2465 -> [w2467 _ _]
                              frame #0 {
                                n1759 = property on="树形控件 2" class="Tree (严格)" props=["Active Item Tag", "ActiveColNum", "Cell String"]("Active Item Tag"="循环水温度" ("活动项:标识符"), "ActiveColNum"=w2467) -> ()  [unwired: 2 in, 3 out]
                              }
                              frame #1 {
                              }
                              frame #2 {
                              }
                            }
                          }
                        }
                      }
                    }
                  }
                }
              }
              frame True {
              }
            }
          }
        }
      }
      event "保存": Value Change {
        n1760 = event-data() -> ()  [unwired: 1 in, 6 out]
        n1761 = property on="通道选择" class="RadioBtnsControl (严格)"() -> ("Value"=w2470:enum32{"ALL", "A1", "A2", "A3", "A4"})  [unwired: 2 in, 2 out]
        n1762 = disable-structure shown="禁用" {
          frame Disabled {
            n1763 = property on="树形控件 2" class="Tree (严格)" props=["Active Item Tag", "ActiveColNum", "Cell String"]() -> ()  [unwired: 4 in, 3 out]
          }
          frame Enabled {
          }
        }
        n1764 = case shown="\"A1\", 默认" w2470 {
          frame "ALL" {
          }
          frame "A1", Default {
            # "<=10℃"
            n1765 = property on="水质换水" class="DigNum (严格)"() -> ("Value"=w2529:dbl)  [unwired: 2 in, 2 out]
            n1766 = property on="氢气出口背压设定：" class="DigNum (严格)"() -> ("Value"=w2533:dbl)  [unwired: 2 in, 2 out]
            n1767 = property on="氢气出口最大压力：" class="DigNum (严格)"() -> ("Value"=w2499:dbl)  [unwired: 2 in, 2 out]
            n1768 = property on="冷却水最高温度：" class="DigNum (严格)"() -> ("Value"=w2479:dbl)  [unwired: 2 in, 2 out]
            n1769 = property on="电解槽最高温度：" class="DigNum (严格)"() -> ("Value"=w2511:dbl)  [unwired: 2 in, 2 out]
            n1770 = property on="水箱补水液位：" class="DigNum (严格)"() -> ("Value"=w2524:dbl)  [unwired: 2 in, 2 out]
            n1771 = property on="气液分离液位：" class="DigNum (严格)"() -> ("Value"=w2518:dbl)  [unwired: 2 in, 2 out]
            n1772 = property on="氢气最大露点：" class="DigNum (严格)"() -> ("Value"=w2514:dbl)  [unwired: 2 in, 2 out]
            n1773 = property on="电解槽最大电压" class="DigNum (严格)"() -> ("Value"=w2507:dbl)  [unwired: 2 in, 2 out]
            n1774 = property on="循环水最差水质" class="DigNum (严格)"() -> ("Value"=w2494:dbl)  [unwired: 2 in, 2 out]
            n1775 = property on="水箱最低液位" class="DigNum (严格)"() -> ("Value"=w2504:dbl)  [unwired: 2 in, 2 out]
            n1776 = Format Into String(format string="%.2f" ("格式字符串"), w2529) -> (resulting string=w2527:string)  [unwired: 2 in, 1 out]
            n1777 = Format Into String(format string="%d" ("格式字符串"), w2524) -> (resulting string=w2523:string)  [unwired: 2 in, 1 out]
            n1778 = Format Into String(format string="%d" ("格式字符串"), w2511) -> (resulting string=w2510:string)  [unwired: 2 in, 1 out]
            n1779 = Format Into String(format string="%d" ("格式字符串"), w2479) -> (resulting string=w2478:string)  [unwired: 2 in, 1 out]
            n1780 = Format Into String(format string="%d" ("格式字符串"), w2504) -> (resulting string=w2503:string)  [unwired: 2 in, 1 out]
            n1781 = Format Into String(format string="%.2f" ("格式字符串"), w2533) -> (resulting string=w2532:string)  [unwired: 2 in, 1 out]
            n1782 = Format Into String(format string="%.2f" ("格式字符串"), w2518) -> (resulting string=w2520:string)  [unwired: 2 in, 1 out]
            n1783 = Format Into String(format string="%.1f" ("格式字符串"), w2514) -> (resulting string=w2516:string)  [unwired: 2 in, 1 out]
            n1784 = Format Into String(format string="%.2f" ("格式字符串"), w2507) -> (resulting string=w2506:string)  [unwired: 2 in, 1 out]
            n1785 = Format Into String(format string="%.2f" ("格式字符串"), w2499) -> (resulting string=w2501:string)  [unwired: 2 in, 1 out]
            n1786 = Format Into String(format string="%.2f" ("格式字符串"), w2494) -> (resulting string=w2496:string)  [unwired: 2 in, 1 out]
            n1787 = Concatenate Strings(w2506, "V" ("字符串")) -> (w2487:string)
            n1788 = Concatenate Strings(w2510, "℃" ("字符串")) -> (w2488:string)
            n1789 = Concatenate Strings(w2478, "℃" ("字符串")) -> (w2476:string)
            n1790 = Concatenate Strings("<=" ("字符串"), w2527, "MΩ.cm" ("字符串")) -> (w2492:string)
            n1791 = Concatenate Strings(w2523, "cm" ("字符串")) -> (w2491:string)
            n1792 = Concatenate Strings(w2520, "cm" ("字符串")) -> (w2490:string)
            n1793 = Concatenate Strings("<=" ("字符串"), w2516, "℃" ("字符串")) -> (w2489:string)
            n1794 = Concatenate Strings(w2503, "cm" ("字符串")) -> (w2486:string)
            n1795 = Concatenate Strings(w2532, "MPa" ("字符串")) -> (w2493:string)
            n1796 = Concatenate Strings(w2501, "MPa" ("字符串")) -> (w2485:string)
            n1797 = Concatenate Strings(w2496, "MΩ.cm" ("字符串")) -> (w2484:string)
            n1798 = Build Array(w2493, w2492, w2491, w2490, w2489, w2488, w2487, w2476, w2486, w2485, w2484) -> (w2483:string[])
            n1799 = case shown="\"200ml/min\", 默认" "流量" {
              tunnel: ["200ml/min" "600l/min" "800l/min" "1000l/min" "1200l/min" "1400l/min" "1600l/min" "400ml/min"] -> w2536
              frame "200ml/min", Default {
              }
              frame "600ml/min" {
              }
              frame "800ml/min" {
              }
              frame "1000ml/min" {
              }
              frame "1200ml/min" {
              }
              frame "1400ml/min" {
              }
              frame "1600ml/min" {
              }
              frame "400lml/min" {
              }
            }
            n1800 = case shown="\"二线\"" "单选按钮 2" {
              tunnel: ["四线制" "二线制"] -> w2535
              frame "四线", Default {
              }
              frame "二线" {
              }
            }
            n1801 = Divide(x="温度25", y=10) -> (x/y=w2473:dbl)
            n1802 = Format Into String(format string="%d" ("格式字符串"), w2473) -> (resulting string=w2537:string)  [unwired: 2 in, 1 out]
            n1803 = property on="数据" class="Str"() -> ("Value"=w2471:string)  [unwired: 2 in, 2 out]
            n1804 = Build Array (concatenate)(w2537, w2471, w2536, w2471, w2535, w2483) -> (w2481:string[])
            n1805 = for {
              tunnel: string[] ["循环水温度", "温度控制串口", "循环水流速", "流速控制串口", "采样方式", "氢气出口背压设定", "水质换水", "水箱补水液位", "气液分离器排水液位", "氢气最大露点", "电解槽最高温度", "电解槽最大电压", "冷却水最高温度", "水箱最低液位", "氢气出口最大压力", "循环水最差水质"] -> [w2543] mode=indexing
              tunnel: w2481 -> [w2541] mode=indexing
              n1806 = property on="通道选择" class="RadioBtnsControl (严格)"() -> ("Value"=w2542:enum32{"ALL", "A1", "A2", "A3", "A4"})  [unwired: 2 in, 2 out]
              n1807 = property on="树形控件 2" class="Tree (严格)"("Active Item Tag"=w2543, "ActiveColNum"=w2542, "Cell String"=w2541) -> ()  [unwired: 2 in, 2 out]
            }
          }
        }
      }
      event "温度25": Value Change {
        n1808 = event-data() -> ("NewVal"=w2555:u16)  [unwired: 1 in, 5 out]
        n1809 = Quotient & Remainder(x=w2555, y=u16 100) -> (x-y*floor(x/y)=w2558:u16)  [unwired: 1 out]
        n1810 = Equal?(x=w2558, y=u16 0) -> (x = y?=w2556:bool)
        n1811 = case shown="假" w2556 {
          tunnel: w2555 -> [w2564 w2618]
          tunnel: w2554 -> [w2562 w2611]
          frame True {
            n1812 = flat-sequence {
              tunnel: w2562 -> [w2574]
              tunnel: [w2574] -> w2560
              tunnel: [w2575] -> w2561
              tunnel: w2560 -> [w2575]
              tunnel: [w2579] -> w2572
              tunnel: [w2578] -> w2571
              tunnel: w2561 -> [w2577]
              tunnel: w2572 -> [w2587]
              tunnel: w2571 -> [w2586]
              tunnel: [w2583] -> w2570
              tunnel: [w2582] -> w2569
              tunnel: w2570 -> [w2593]
              tunnel: w2569 -> [w2592]
              tunnel: [w2590] -> w2568
              tunnel: [w2589] -> w2567
              tunnel: w2564 -> [w2588]
              tunnel: [w2588] -> w2563
              tunnel: w2568 -> [w2603]
              tunnel: w2567 -> [w2601]
              tunnel: [w2596] -> w2566
              tunnel: [w2595] -> w2565
              tunnel: w2563 -> [w2594]
              tunnel: w2566 -> [w2605]
              tunnel: w2565 -> [w2604]
              frame #0 {
                n1813 = property on="字符串" class="Str"("Value"="0" ("字符串")) -> ()  [unwired: 2 in, 2 out]
              }
              frame #1 {
                n1814 = Wait (ms)(milliseconds to wait=u32 800 ("等待时间（毫秒）")) -> ()  [unwired: 1 out]
              }
              frame #2 {
                n1815 = call-dynamic "Write Single Holding Register.vi"("holding register value"=u16 2, "address"=u16 271, "Modbus master in"=w2577) -> ("error out"=w2578:errorcluster, "Modbus master out"=w2579:refnum<class "Modbus Master.lvclass">)  [unwired: 7 in]
              }
              frame #3 {
                n1816 = call-dynamic "Write Single Holding Register.vi"("error in (no error)"=w2586, "holding register value"=u16 9999, "address"=u16 20484, "Modbus master in"=w2587) -> ("error out"=w2582:errorcluster, "Modbus master out"=w2583:refnum<class "Modbus Master.lvclass">)  [unwired: 6 in]
              }
              frame #4 {
                n1817 = call-dynamic "Write Single Holding Register.vi"("error in (no error)"=w2592, "holding register value"=w2588, "address"=u16 20485, "Modbus master in"=w2593) -> ("error out"=w2589:errorcluster, "Modbus master out"=w2590:refnum<class "Modbus Master.lvclass">)  [unwired: 6 in]
              }
              frame #5 {
                n1818 = call-dynamic "Write Single Holding Register.vi"("error in (no error)"=w2601, "holding register value"=u16 0, "address"=u16 20488, "Modbus master in"=w2603) -> ("error out"=w2600:errorcluster, "Modbus master out"=w2602:refnum<class "Modbus Master.lvclass">)  [unwired: 6 in]
                n1819 = call-dynamic "Write Single Holding Register.vi"("error in (no error)"=w2600, "holding register value"=w2594, "address"=u16 20489, "Modbus master in"=w2602) -> ("error out"=w2595:errorcluster, "Modbus master out"=w2596:refnum<class "Modbus Master.lvclass">)  [unwired: 6 in]
              }
              frame #6 {
                n1820 = call-dynamic "Write Single Holding Register.vi"("error in (no error)"=w2604, "holding register value"=u16 0, "address"=u16 271, "Modbus master in"=w2605) -> ()  [unwired: 6 in, 2 out]
              }
              frame #7 {
                n1821 = property on="字符串" class="Str"("Value"="2" ("字符串")) -> ()  [unwired: 2 in, 2 out]
              }
              frame #8 {
                n1822 = Wait (ms)(milliseconds to wait=u32 800 ("等待时间（毫秒）")) -> ()  [unwired: 1 out]
              }
            }
          }
          frame False {
            n1823 = flat-sequence {
              tunnel: w2618 -> [w2629]
              tunnel: [w2629] -> w2617
              tunnel: [w2628] -> w2612
              tunnel: w2611 -> [w2628]
              tunnel: w2617 -> [w2631]
              tunnel: [w2631] -> w2615
              tunnel: w2612 -> [w2630]
              tunnel: [w2630] -> w2610
              tunnel: [w2636] -> w2626
              tunnel: [w2635] -> w2625
              tunnel: [w2634] -> w2616
              tunnel: w2615 -> [w2634]
              tunnel: w2610 -> [w2633]
              tunnel: w2626 -> [w2645]
              tunnel: w2625 -> [w2644]
              tunnel: [w2641] -> w2624
              tunnel: [w2640] -> w2623
              tunnel: w2616 -> [w2639]
              tunnel: [w2639] -> w2614
              tunnel: w2624 -> [w2651]
              tunnel: w2623 -> [w2650]
              tunnel: [w2648] -> w2622
              tunnel: [w2647] -> w2621
              tunnel: w2614 -> [w2646]
              tunnel: [w2646] -> w2613
              tunnel: w2622 -> [w2661]
              tunnel: w2621 -> [w2659]
              tunnel: [w2654] -> w2620
              tunnel: [w2653] -> w2619
              tunnel: w2613 -> [w2652]
              tunnel: w2620 -> [w2663]
              tunnel: w2619 -> [w2662]
              frame #0 {
                n1824 = property on="字符串" class="Str"("Value"="0" ("字符串")) -> ()  [unwired: 2 in, 2 out]
              }
              frame #1 {
                n1825 = Wait (ms)(milliseconds to wait=u32 800 ("等待时间（毫秒）")) -> ()  [unwired: 1 out]
              }
              frame #2 {
                n1826 = call-dynamic "Write Single Holding Register.vi"("holding register value"=u16 2, "address"=u16 271, "Modbus master in"=w2633) -> ("error out"=w2635:errorcluster, "Modbus master out"=w2636:refnum<class "Modbus Master.lvclass">)  [unwired: 7 in]
              }
              frame #3 {
                n1827 = call-dynamic "Write Single Holding Register.vi"("error in (no error)"=w2644, "holding register value"=u16 9999, "address"=u16 20484, "Modbus master in"=w2645) -> ("error out"=w2640:errorcluster, "Modbus master out"=w2641:refnum<class "Modbus Master.lvclass">)  [unwired: 6 in]
              }
              frame #4 {
                n1828 = call-dynamic "Write Single Holding Register.vi"("error in (no error)"=w2650, "holding register value"=w2646, "address"=u16 20485, "Modbus master in"=w2651) -> ("error out"=w2647:errorcluster, "Modbus master out"=w2648:refnum<class "Modbus Master.lvclass">)  [unwired: 6 in]
              }
              frame #5 {
                n1829 = call-dynamic "Write Single Holding Register.vi"("error in (no error)"=w2659, "holding register value"=u16 0, "address"=u16 20488, "Modbus master in"=w2661) -> ("error out"=w2658:errorcluster, "Modbus master out"=w2660:refnum<class "Modbus Master.lvclass">)  [unwired: 6 in]
                n1830 = call-dynamic "Write Single Holding Register.vi"("error in (no error)"=w2658, "holding register value"=w2652, "address"=u16 20489, "Modbus master in"=w2660) -> ("error out"=w2653:errorcluster, "Modbus master out"=w2654:refnum<class "Modbus Master.lvclass">)  [unwired: 6 in]
              }
              frame #6 {
                n1831 = call-dynamic "Write Single Holding Register.vi"("error in (no error)"=w2662, "holding register value"=u16 0, "address"=u16 271, "Modbus master in"=w2663) -> ()  [unwired: 6 in, 2 out]
              }
              frame #7 {
                n1832 = property on="字符串" class="Str"("Value"="1" ("字符串")) -> ()  [unwired: 2 in, 2 out]
              }
              frame #8 {
                n1833 = Wait (ms)(milliseconds to wait=u32 800 ("等待时间（毫秒）")) -> ()  [unwired: 1 out]
              }
            }
          }
        }
        n1834 = property on="温度25" class="Ring (严格)" props=["Value"]() -> ()  [unwired: 2 in, 3 out]
      }
      event "添加工步", "保存工步": Value Change {
        n1835 = event-data() -> ("CtlRef"=w2669:refnum<vi>)  [unwired: 1 in, 5 out]
        n1836 = property class="Bool"(reference=w2669) -> ("BoolText.Text"=w2668:string)  [unwired: 1 in, 2 out]
        n1837 = case shown="\"保存工步\"" w2668 {
          frame "假", Default {
          }
          frame "显示工步曲线" {
            n1838 = flat-sequence {
              frame #0 {
                (unwired) dbl[] []
              }
              frame #1 {
              }
              frame #2 {
                n1839 = property on="数组" class="Arr (严格)"() -> ("Value"=w2675:string[][])  [unwired: 2 in, 2 out]
                n1840 = Index Array(array=w2675, index (col)=3 ("禁用的索引 (列)")) -> (element=w2672:string[])  [unwired: 1 in]
                n1841 = Index Array(array=w2675, index (col)=5 ("禁用的索引 (列)")) -> (element=w2671:string[])  [unwired: 1 in]
                n1842 = Search 1D Array(1D array=w2672, element=" " ("元素")) -> (index of element=w2673:i32)  [unwired: 1 in]
                n1843 = for {
                  N: w2673 -> [_]
                  tunnel: w2672 -> [w2690] mode=indexing
                  tunnel: w2671 -> [w2687] mode=indexing
                  shift-right: [w2679] -> _
                  shift-left: dbl[] [] -> [w2680]
                  n1844 = Scan From String(format string="%.2f" ("格式字符串"), input string=w2690) -> (output 1=w2683:dbl)  [unwired: 3 in, 3 out]
                  n1845 = Scan From String(format string="%.2f" ("格式字符串"), input string=w2687) -> (output 1=w2686:dbl)  [unwired: 3 in, 3 out]
                  n1846 = Divide(x=w2686, y=10.0) -> (x/y=w2684:dbl)
                  n1847 = Round Toward +Infinity(x=w2684) -> (ceil(x): smallest int >= x=w2682:dbl)
                  n1848 = To Long Integer(number=w2682) -> (32bit integer=w2678:i32)
                  n1849 = Initialize Array(w2683, w2678) -> (w2681:dbl[])
                  n1850 = Build Array (concatenate)(w2680, w2681) -> (w2679:dbl[])
                }
              }
            }
          }
          frame "保存工步" {
            n1851 = Current VI's Path() -> (path=w2703:path)
            n1852 = Strip Path(path=w2703) -> (stripped path=w2702:path)  [unwired: 1 out]
            n1853 = String To Path(string="工步") -> (path=w2700:path)
            n1854 = Build Path(base path=w2702, name or relative path=w2700) -> (appended path=w2699:path)
            n1855 = call "文件对话框3"("start path"=w2699, "pattern (all files)"=".xls" ("pattern label"), "pattern label"="工步文件" ("pattern (all files)")) -> ("selected path"=w2698:path)  [unwired: 9 in, 3 out]
            n1856 = call-poly <vilib>:"Write Delimited Spreadsheet.vi"("file path (dialog if empty)"=w2698, "1D data"=string[] ["序号", "电源模式", "电压(V)", "电流(A)", "功率(W)", "运行时间(S)"]) -> ("new file path (Not A Path if cancelled)"=w2696:path, "error out"=w2695:errorcluster)  [unwired: 12 in]
            n1857 = property on="数组" class="Arr (严格)"() -> ("Value"=w2691:string[][])  [unwired: 2 in, 2 out]
            n1858 = call-poly <vilib>:"Write Delimited Spreadsheet.vi"("file path (dialog if empty)"=w2696, "2D data"=w2691, "append to file? (new file:F)"=TRUE, "error in (no error)"=w2695) -> ()  [unwired: 10 in, 2 out]
          }
          frame "添加工步" {
            n1859 = flat-sequence {
              tunnel: [w2719] -> w2707
              tunnel: [w2715] -> w2706
              tunnel: [w2713] -> w2705
              tunnel: [w2712] -> w2704
              tunnel: w2706 -> [w2737]
              tunnel: w2707 -> [w2738]
              tunnel: w2705 -> [w2736]
              tunnel: w2704 -> [w2735]
              frame #0 {
                # "\\pem\\添加工步.vi"
                n1860 = property on="队列输出 2" class="TypRef (严格)" props=["Value"]() -> ()  [unwired: 2 in, 3 out]
                n1861 = property on="电源类型" class="Ring (严格)"() -> ("Value"=w2711:u16)  [unwired: 2 in, 2 out]
                n1862 = call <vilib>:"Application Directory.vi"() -> ("Application Directory"=w2710:path)
                n1863 = Build Path(base path=w2710, name or relative path="\\pem\\添加工步.vi") -> (appended path=w2708:path)
                n1864 = case shown="0, 默认" w2711 {
                  tunnel: ["ITECH" "TDK"] -> w2720
                  frame 0, Default {
                  }
                  frame 1 {
                  }
                }
                n1865 = property on="通道选择 2" class="RadioBtnsControl (严格)"() -> ("Value"=w2714:enum32{"未选择", "A1", "A2", "A3", "A4"})  [unwired: 2 in, 2 out]
                n1866 = Open VI Reference(type specifier VI Refnum (for type only)=refnum<vi> refnum ("类型说明符VI引用句柄（仅用于类型）"), vi path=w2708, options=128 ("选项")) -> (vi reference=w2722:refnum<vi>, error out=w2721:errorcluster)  [unwired: 3 in]
                n1867 = case shown="\"A1\", 默认" w2714 {
                  tunnel: [w2726 w2728 w2730 w2732] -> w2713
                  tunnel: [w2725 w2727 w2729 w2731] -> w2712
                  frame "A1", Default {
                    n1868 = control-ref of="数组"() -> (w2726:refnum<vi>)
                    n1869 = property on="数组" class="Arr (严格)"() -> ("Value"=w2725:string[][])  [unwired: 2 in, 2 out]
                  }
                  frame "A2" {
                    n1870 = control-ref of="数组 10"() -> (w2728:refnum<vi>)
                    n1871 = property on="数组 10" class="Arr (严格)"() -> ("Value"=w2727:string[][])  [unwired: 2 in, 2 out]
                  }
                  frame "A3" {
                    n1872 = control-ref of="数组 11"() -> (w2730:refnum<vi>)
                    n1873 = property on="数组 11" class="Arr (严格)"() -> ("Value"=w2729:string[][])  [unwired: 2 in, 2 out]
                  }
                  frame "A4" {
                    n1874 = control-ref of="数组 12"() -> (w2732:refnum<vi>)
                    n1875 = property on="数组 12" class="Arr (严格)"() -> ("Value"=w2731:string[][])  [unwired: 2 in, 2 out]
                  }
                }
                n1876 = call-by-ref "?"(reference=w2722, error in=w2721, "字符串"=w2720, "Arr引用句柄"=w2713) -> (reference out=w2717:refnum<vi>, error out=w2719:errorcluster, "布尔"=w2715:bool)  [unwired: 9 in]
                n1877 = property on="数组 2" class="Arr (严格)"() -> ("Value"=w2718:refnum<vi>[])  [unwired: 2 in, 2 out]
                n1878 = Insert Into Array(array=w2718, new element=w2717) -> (w2716:refnum<vi>[])  [unwired: 1 in]
                n1879 = property on="数组 2" class="Arr (严格)"("Value"=w2716) -> ()  [unwired: 2 in, 2 out]
              }
              frame #1 {
                n1880 = case shown="真" w2737 {
                  tunnel: w2738 -> [_ w2742]
                  tunnel: w2736 -> [_ w2740]
                  tunnel: w2735 -> [_ w2739]
                  frame False {
                  }
                  frame True {
                    n1881 = flat-sequence {
                      tunnel: w2742 -> [w2748]
                      tunnel: [w2747] -> w2741
                      tunnel: w2740 -> [w2746]
                      tunnel: w2741 -> [w2754]
                      tunnel: [w2762] -> w2745
                      tunnel: [w2759] -> w2744
                      tunnel: [w2764] -> w2743
                      tunnel: w2739 -> [w2759]
                      tunnel: w2745 -> [w2777]
                      tunnel: w2744 -> [w2778]
                      tunnel: w2743 -> [w2779]
                      frame #0 {
                        n1882 = property class="Arr (严格)"(reference=w2746, error in=w2748) -> (error out=w2752:errorcluster, "Value"=w2750:string[][])  [unwired: 1 out]
                        n1883 = Insert Into Array(array=w2750, new element=string[] [" ", " ", " ", " ", " ", " "] ("new element/subarray")) -> (w2751:string[][])  [unwired: 2 in]
                        n1884 = property class="Arr (严格)"(reference=w2746, error in=w2752, "Value"=w2751) -> (error out=w2747:errorcluster)  [unwired: 1 out]
                      }
                      frame #1 {
                        (unwired) TRUE ("删除子项？")
                        (unwired) "A1" ("标识符")
                        n1885 = Unbundle(w2754) -> ("status"=w2758:bool, "code"=w2757:i32)  [unwired: 1 out]
                        n1886 = property on="队列输出 2" class="TypRef (严格)"() -> ("Value"=w2756:refnum<queue>)  [unwired: 2 in, 2 out]
                        n1887 = Bundle("status"=w2758, "code"=w2757, "添加工步") -> (w2753:cluster{"status":bool, "code":i32, string})  [unwired: 1 in]
                        n1888 = Enqueue Element(queue=w2756, element=w2753) -> ()  [unwired: 2 in, 3 out]
                        n1889 = call <vilib>:"Clear Errors.vi"() -> ()  [unwired: 6 in, 2 out]
                      }
                      frame #2 {
                        n1890 = Index Array(array=w2759, index (col)=1 ("索引 (行)")) -> (element=w2771:string[])  [unwired: 1 in]
                        n1891 = Index Array(array=w2759, index (row)=0 ("索引 (行)")) -> (element=w2767:string[])  [unwired: 1 in]
                        n1892 = Index Array(array=w2759, index (row)=0 ("索引 (行)")) -> (element=w2772:string[])  [unwired: 1 in]
                        n1893 = Search 1D Array(1D array=w2771, element=" ") -> (index of element=w2762:i32)  [unwired: 1 in]
                        n1894 = Index Array(array=w2772, index=4 ("索引")) -> (element=w2773:string)
                        n1895 = case shown="\"400\"" w2773 {
                          tunnel: ["ITECH" "ITECH"] -> w2764
                          frame "1700", Default {
                          }
                          frame "400" {
                          }
                        }
                        n1896 = Equal?(x=w2762, y=-1) -> (x = y?=w2760:bool)
                        n1897 = Build Array (concatenate)(w2764, w2767, "未运行") -> (w2765:string[])
                        n1898 = case shown="真" w2760 {
                          tunnel: w2765 -> [_ _]
                          frame False {
                            (unwired) 0 ("新项缩进")
                            (unwired) "A1" ("左单元格字符串")
                          }
                          frame True {
                          }
                        }
                      }
                      frame #3 {
                        n1899 = for {
                          N: w2777 -> [_]
                          tunnel: w2779 -> [w2781]
                          tunnel: w2778 -> [w2782]
                          tunnel: [w2783] -> _ mode=indexing
                          i -> [w2791]
                          n1900 = Index Array(array=w2782, index (row)=w2791) -> (element=w2780:string[])  [unwired: 1 in]
                          n1901 = Build Array (concatenate)(w2781, w2780, "未运行") -> (w2788:string[])
                          n1902 = Bundle("A1", w2788, "", 1, FALSE, 6) -> (w2783:T26)  [unwired: 1 in]
                        }
                      }
                    }
                  }
                }
              }
            }
          }
        }
      }
      event "搜索设备": Value Change {
        n1903 = event-data() -> ()  [unwired: 1 in, 6 out]
        n1904 = property on="表格" class="Tbl (严格)"("Value"=string[][] [] ("表格")) -> (error out=w2792:errorcluster)  [unwired: 2 in, 1 out]
        n1905 = property on="数值 5" class="DigNum (严格)"(error in=w2792, "Value"=0 ("数值 5")) -> (error out=w2795:errorcluster)  [unwired: 1 in, 1 out]
        n1906 = case shown="\"USB\", 默认" "通讯方式选择" {
          tunnel: w2795 -> [_ _ _ _]
          frame "USB", Default {
            n1907 = stacked-sequence {
              frame #0 {
                w2799 = T27 0 items=["仅允许规范名称"=0, "只允许别名"=2, "包含匹配别名"=3, "包含所有别名"=4] ("Search Mode")
                n1908 = VISA Find Resource(10:w2799, 11:"/?*" ("表达式(\"?*\")")) -> (3:w2797:string[])  [unwired: 1 in, 2 out]
                "查找列表" <- w2797
                n1909 = for {
                  tunnel: w2797 -> [w2805] mode=indexing
                  i -> [w2801]
                  n1910 = String Subset(string=w2805, length (rest)=3 ("长度（剩余）")) -> (substring=w2804:string)  [unwired: 1 in]
                  n1911 = Equal?(x=w2804, y="USB") -> (x = y?=w2802:bool)
                  n1912 = case shown="假" w2802 {
                    tunnel: w2801 -> [w2806 _]
                    frame False {
                      n1913 = flat-sequence {
                        tunnel: w2806 -> [w2809]
                        frame #0 {
                          n1914 = property on="查找列表" class="Arr (严格)"() -> ("Value"=w2811:string[])  [unwired: 2 in, 2 out]
                          n1915 = property on="数值 5" class="DigNum (严格)"() -> ("Value"=w2808:i32)  [unwired: 2 in, 2 out]
                          n1916 = Subtract(x=w2809, y=w2808) -> (x-y=w2807:i32)
                          n1917 = Delete From Array(array=w2811, index=w2807) -> (array with subset deleted=w2810:string[])  [unwired: 1 in, 1 out]
                          n1918 = property on="查找列表" class="Arr (严格)"("Value"=w2810) -> ()  [unwired: 2 in, 2 out]
                        }
                        frame #1 {
                          n1919 = Increment(x="数值 5") -> (x+1=w2813:i32)
                          n1920 = property on="数值 5" class="DigNum (严格)"("Value"=w2813) -> ()  [unwired: 2 in, 2 out]
                        }
                      }
                    }
                    frame True {
                    }
                  }
                }
              }
              frame #1 {
                n1921 = property on="查找列表" class="Arr (严格)"() -> ("Value"=w2818:string[])  [unwired: 2 in, 2 out]
                n1922 = for {
                  tunnel: w2818 -> [w2823] mode=indexing
                  tunnel: [w2819] -> w2817 mode=indexing
                  n1923 = To Variant(anything=w2823) -> (Variant=w2822:variant)
                  n1924 = Variant To Data(type=refnum<visa-resource-name> refnum ("VISA resource name out"), Variant=w2822) -> (data=w2820:refnum<visa-resource-name>)  [unwired: 1 in, 1 out]
                  n1925 = property class="Instr"(reference=w2820) -> ("Model Name"=w2819:string)  [unwired: 1 in, 2 out]
                }
                n1926 = property on="查找列表" class="Arr (严格)"() -> ("Value"=w2816:string[])  [unwired: 2 in, 2 out]
                n1927 = Build Array(w2817, w2816) -> (w2815:string[][])
                n1928 = Transpose 2D Array(2D array=w2815) -> (transposed array=w2814:string[][])
                n1929 = property on="表格" class="Tbl (严格)"("Value"=w2814) -> ()  [unwired: 2 in, 2 out]
              }
              frame #2 {
                n1930 = property on="表格" class="Tbl (严格)"() -> ("Value"=w2825:string[][])  [unwired: 2 in, 2 out]
                n1931 = Index Array(array=w2825, index (col)=1 ("禁用的索引 (列)")) -> (element=w2826:string[])  [unwired: 1 in]
                n1932 = property on="串口号" class="Ring (严格)"("Strings []"=w2826) -> ()  [unwired: 2 in, 2 out]
              }
            }
          }
          frame "ETHERNET" {
          }
          frame "RS485" {
          }
          frame "GPIB" {
          }
        }
      }
    }
  }
  n1933 = property class="VI"() -> ("Name"=w6:string)  [unwired: 2 in, 2 out]
  n1934 = Obtain Queue(name (unnamed)=w6, element data type=w6) -> (queue out=w7:refnum<queue>)  [unwired: 3 in, 2 out]
  n1935 = Enqueue Element(queue=w7, element="初始化" ("元素")) -> (queue out=w4:refnum<queue>)  [unwired: 2 in, 2 out]
  n1936 = while {
    tunnel: [w2830] -> w5
    tunnel: w4 -> [w2829]
    stop <- FALSE stop-if-true
    n1937 = Dequeue Element(queue=w2829) -> (queue out=w2828:refnum<queue>, element=w2827:string)  [unwired: 2 in, 2 out]
    n1938 = case shown="\"所有数据退回\"" w2827 {
      tunnel: w2828 -> [w2832 w2833 w2834 w2838 w2842 w2846 w2850 w2854 w2859 w2887 w2915 w2943 w2971 w2999]
      tunnel: [w2832 w2833 w2834 w2838 w2842 w2846 w2850 w2854 w2859 w2887 w2915 w2943 w2971 w2999] -> w2830
      frame "eee", Default {
      }
      frame "初始化" {
      }
      frame "所有数据弹出" {
        n1939 = flat-sequence {
          frame #0 {
            n1940 = invoke on="子面板" class="SubPnl" method="Remove VI"() -> ()  [unwired: 3 in, 3 out]
          }
          frame #1 {
            w2835 = "列表.vi" ("名称（未命名）")
            n1941 = Obtain Queue(name (unnamed)=w2835, element data type=w2835) -> (queue out=w2837:refnum<queue>)  [unwired: 3 in, 2 out]
            n1942 = Enqueue Element(queue=w2837, element="111" ("元素")) -> ()  [unwired: 2 in, 3 out]
          }
        }
      }
      frame "工步弹出" {
        n1943 = flat-sequence {
          frame #0 {
            n1944 = invoke on="子面板1" class="SubPnl" method="Remove VI"() -> ()  [unwired: 3 in, 3 out]
          }
          frame #1 {
            w2839 = "工步列表.vi" ("名称（未命名）")
            n1945 = Obtain Queue(name (unnamed)=w2839, element data type=w2839) -> (queue out=w2841:refnum<queue>)  [unwired: 3 in, 2 out]
            n1946 = Enqueue Element(queue=w2841, element="111" ("元素")) -> ()  [unwired: 2 in, 3 out]
          }
        }
      }
      frame "极化弹出" {
        n1947 = flat-sequence {
          frame #0 {
            n1948 = invoke on="子面板2" class="SubPnl" method="Remove VI"() -> ()  [unwired: 3 in, 3 out]
          }
          frame #1 {
            w2843 = "极化曲线.vi" ("名称（未命名）")
            n1949 = Obtain Queue(name (unnamed)=w2843, element data type=w2843) -> (queue out=w2845:refnum<queue>)  [unwired: 3 in, 2 out]
            n1950 = Enqueue Element(queue=w2845, element="111" ("元素")) -> ()  [unwired: 2 in, 3 out]
          }
        }
      }
      frame "温度弹出" {
        n1951 = flat-sequence {
          frame #0 {
            n1952 = invoke on="子面板3" class="SubPnl" method="Remove VI"() -> ()  [unwired: 3 in, 3 out]
          }
          frame #1 {
            w2847 = "温度.vi" ("名称（未命名）")
            n1953 = Obtain Queue(name (unnamed)=w2847, element data type=w2847) -> (queue out=w2849:refnum<queue>)  [unwired: 3 in, 2 out]
            n1954 = Enqueue Element(queue=w2849, element="111" ("元素")) -> ()  [unwired: 2 in, 3 out]
          }
        }
      }
      frame "压力弹出" {
        n1955 = flat-sequence {
          frame #0 {
            n1956 = invoke on="子面板4" class="SubPnl" method="Remove VI"() -> ()  [unwired: 3 in, 3 out]
          }
          frame #1 {
            w2851 = "压力.vi" ("名称（未命名）")
            n1957 = Obtain Queue(name (unnamed)=w2851, element data type=w2851) -> (queue out=w2853:refnum<queue>)  [unwired: 3 in, 2 out]
            n1958 = Enqueue Element(queue=w2853, element="111" ("元素")) -> ()  [unwired: 2 in, 3 out]
          }
        }
      }
      frame "水质弹出" {
        n1959 = flat-sequence {
          frame #0 {
            n1960 = invoke on="子面板5" class="SubPnl" method="Remove VI"() -> ()  [unwired: 3 in, 3 out]
          }
          frame #1 {
            w2855 = "水质.vi" ("名称（未命名）")
            n1961 = Obtain Queue(name (unnamed)=w2855, element data type=w2855) -> (queue out=w2857:refnum<queue>)  [unwired: 3 in, 2 out]
            n1962 = Enqueue Element(queue=w2857, element="111" ("元素")) -> ()  [unwired: 2 in, 3 out]
          }
        }
      }
      frame "所有数据退回" {
        n1963 = property on="数组 3" class="Arr (严格)"() -> ("Value"=w2858:refnum<vi>[])  [unwired: 2 in, 2 out]
        n1964 = for {
          tunnel: w2858 -> [w2860] mode=indexing
          n1965 = property class="VI"(reference=w2860) -> ("Name"=w2863:string)  [unwired: 1 in, 2 out]
          n1966 = Equal?(x=w2863, y="列表.vi") -> (x = y?=w2861:bool)
          n1967 = case shown="真" w2861 {
            tunnel: w2860 -> [_ w2864]
            frame False {
            }
            frame True {
              n1968 = property class="VI"(reference=w2864) -> (reference out=w2867:refnum<vi>, error out=w2865:errorcluster, "Exec.State"=w2866:T23)  [unwired: 1 in]
              n1969 = case shown="\"Running\"" w2866 {
                tunnel: w2867 -> [_ w2875 w2882 w2885]
                tunnel: w2865 -> [w2868 w2872 w2879 w2884]
                tunnel: [w2868 w2869 w2876 w2883] -> _
                frame "Bad", Default {
                  # "VI包含错误并且无法执行。"
                }
                frame "Idle" {
                  # "VI位于内存中但没有运行"
                  n1970 = invoke class="VI" method="Run VI"(reference=w2875, error in=w2872, "Wait until done"=FALSE ("结束前等待"), "Auto Dispose Ref"=FALSE ("自动销毁引用")) -> (reference out=w2871:refnum<vi>, error out=w2870:errorcluster)  [unwired: 1 in, 3 out]
                  n1971 = invoke on="子面板" class="SubPnl" method="Insert VI"(error in=w2870, "VI Ref"=w2871) -> (error out=w2869:errorcluster)  [unwired: 2 in, 3 out]
                }
                frame "Run top level" {
                  # "VI是活动层次结构中的顶层VI"
                  n1972 = property class="VI"(reference=w2882, error in=w2879, "FP.State"=T15."Closed" ("前面板窗口:状态")) -> (reference out=w2878:refnum<vi>, error out=w2880:errorcluster)
                  n1973 = call <vilib>:"Clear Errors.vi"("error in (no error)"=w2880) -> ("error out"=w2877:errorcluster)  [unwired: 5 in, 1 out]
                  n1974 = invoke on="子面板" class="SubPnl" method="Insert VI"(error in=w2877, "VI Ref"=w2878) -> (error out=w2876:errorcluster)  [unwired: 2 in, 3 out]
                }
                frame "Running" {
                  # "VI已由一个或多个处于活动状态的顶层VI保留为执行"
                  n1975 = invoke on="子面板" class="SubPnl" method="Insert VI"(error in=w2884, "VI Ref"=w2885) -> (error out=w2883:errorcluster)  [unwired: 2 in, 3 out]
                }
              }
            }
          }
        }
      }
      frame "工步退回" {
        n1976 = property on="数组 3" class="Arr (严格)"() -> ("Value"=w2886:refnum<vi>[])  [unwired: 2 in, 2 out]
        n1977 = for {
          tunnel: w2886 -> [w2888] mode=indexing
          n1978 = property class="VI"(reference=w2888) -> ("Name"=w2891:string)  [unwired: 1 in, 2 out]
          n1979 = Equal?(x=w2891, y="工步列表.vi") -> (x = y?=w2889:bool)
          n1980 = case shown="真" w2889 {
            tunnel: w2888 -> [_ w2892]
            frame False {
            }
            frame True {
              n1981 = property class="VI"(reference=w2892) -> (reference out=w2893:refnum<vi>, error out=w2895:errorcluster, "Exec.State"=w2894:T23)  [unwired: 1 in]
              n1982 = case shown="\"Run top level\"" w2894 {
                tunnel: w2893 -> [_ w2903 w2910 w2913]
                tunnel: w2895 -> [w2896 w2900 w2907 w2912]
                tunnel: [w2896 w2897 w2904 w2911] -> _
                frame "Bad", Default {
                  # "VI包含错误并且无法执行。"
                }
                frame "Idle" {
                  # "VI位于内存中但没有运行"
                  n1983 = invoke class="VI" method="Run VI"(reference=w2903, error in=w2900, "Wait until done"=FALSE ("结束前等待"), "Auto Dispose Ref"=FALSE ("自动销毁引用")) -> (reference out=w2899:refnum<vi>, error out=w2898:errorcluster)  [unwired: 1 in, 3 out]
                  n1984 = invoke on="子面板1" class="SubPnl" method="Insert VI"(error in=w2898, "VI Ref"=w2899) -> (error out=w2897:errorcluster)  [unwired: 2 in, 3 out]
                }
                frame "Run top level" {
                  # "VI是活动层次结构中的顶层VI"
                  n1985 = property class="VI"(reference=w2910, error in=w2907, "FP.State"=T15."Closed" ("前面板窗口:状态")) -> (reference out=w2906:refnum<vi>, error out=w2908:errorcluster)
                  n1986 = call <vilib>:"Clear Errors.vi"("error in (no error)"=w2908) -> ("error out"=w2905:errorcluster)  [unwired: 5 in, 1 out]
                  n1987 = invoke on="子面板1" class="SubPnl" method="Insert VI"(error in=w2905, "VI Ref"=w2906) -> (error out=w2904:errorcluster)  [unwired: 2 in, 3 out]
                }
                frame "Running" {
                  # "VI已由一个或多个处于活动状态的顶层VI保留为执行"
                  n1988 = invoke on="子面板1" class="SubPnl" method="Insert VI"(error in=w2912, "VI Ref"=w2913) -> (error out=w2911:errorcluster)  [unwired: 2 in, 3 out]
                }
              }
            }
          }
        }
      }
      frame "极化退回" {
        n1989 = property on="数组 3" class="Arr (严格)"() -> ("Value"=w2914:refnum<vi>[])  [unwired: 2 in, 2 out]
        n1990 = for {
          tunnel: w2914 -> [w2916] mode=indexing
          n1991 = property class="VI"(reference=w2916) -> ("Name"=w2919:string)  [unwired: 1 in, 2 out]
          n1992 = Equal?(x=w2919, y="极化曲线.vi") -> (x = y?=w2917:bool)
          n1993 = case shown="真" w2917 {
            tunnel: w2916 -> [_ w2920]
            frame False {
            }
            frame True {
              n1994 = property class="VI"(reference=w2920) -> (reference out=w2921:refnum<vi>, error out=w2923:errorcluster, "Exec.State"=w2922:T23)  [unwired: 1 in]
              n1995 = case shown="\"Running\"" w2922 {
                tunnel: w2921 -> [_ w2931 w2938 w2941]
                tunnel: w2923 -> [w2924 w2928 w2935 w2940]
                tunnel: [w2924 w2925 w2932 w2939] -> _
                frame "Bad", Default {
                  # "VI包含错误并且无法执行。"
                }
                frame "Idle" {
                  # "VI位于内存中但没有运行"
                  n1996 = invoke class="VI" method="Run VI"(reference=w2931, error in=w2928, "Wait until done"=FALSE ("结束前等待"), "Auto Dispose Ref"=FALSE ("自动销毁引用")) -> (reference out=w2927:refnum<vi>, error out=w2926:errorcluster)  [unwired: 1 in, 3 out]
                  n1997 = invoke on="子面板2" class="SubPnl" method="Insert VI"(error in=w2926, "VI Ref"=w2927) -> (error out=w2925:errorcluster)  [unwired: 2 in, 3 out]
                }
                frame "Run top level" {
                  # "VI是活动层次结构中的顶层VI"
                  n1998 = property class="VI"(reference=w2938, error in=w2935, "FP.State"=T15."Closed" ("前面板窗口:状态")) -> (reference out=w2934:refnum<vi>, error out=w2936:errorcluster)
                  n1999 = call <vilib>:"Clear Errors.vi"("error in (no error)"=w2936) -> ("error out"=w2933:errorcluster)  [unwired: 5 in, 1 out]
                  n2000 = invoke on="子面板2" class="SubPnl" method="Insert VI"(error in=w2933, "VI Ref"=w2934) -> (error out=w2932:errorcluster)  [unwired: 2 in, 3 out]
                }
                frame "Running" {
                  # "VI已由一个或多个处于活动状态的顶层VI保留为执行"
                  n2001 = invoke on="子面板2" class="SubPnl" method="Insert VI"(error in=w2940, "VI Ref"=w2941) -> (error out=w2939:errorcluster)  [unwired: 2 in, 3 out]
                }
              }
            }
          }
        }
      }
      frame "温度退回" {
        n2002 = property on="数组 3" class="Arr (严格)"() -> ("Value"=w2942:refnum<vi>[])  [unwired: 2 in, 2 out]
        n2003 = for {
          tunnel: w2942 -> [w2944] mode=indexing
          n2004 = property class="VI"(reference=w2944) -> ("Name"=w2947:string)  [unwired: 1 in, 2 out]
          n2005 = Equal?(x=w2947, y="温度.vi") -> (x = y?=w2945:bool)
          n2006 = case shown="真" w2945 {
            tunnel: w2944 -> [_ w2948]
            frame False {
            }
            frame True {
              n2007 = property class="VI"(reference=w2948) -> (reference out=w2949:refnum<vi>, error out=w2951:errorcluster, "Exec.State"=w2950:T23)  [unwired: 1 in]
              n2008 = case shown="\"Running\"" w2950 {
                tunnel: w2949 -> [_ w2959 w2966 w2969]
                tunnel: w2951 -> [w2952 w2956 w2963 w2968]
                tunnel: [w2952 w2953 w2960 w2967] -> _
                frame "Bad", Default {
                  # "VI包含错误并且无法执行。"
                }
                frame "Idle" {
                  # "VI位于内存中但没有运行"
                  n2009 = invoke class="VI" method="Run VI"(reference=w2959, error in=w2956, "Wait until done"=FALSE ("结束前等待"), "Auto Dispose Ref"=FALSE ("自动销毁引用")) -> (reference out=w2955:refnum<vi>, error out=w2954:errorcluster)  [unwired: 1 in, 3 out]
                  n2010 = invoke on="子面板3" class="SubPnl" method="Insert VI"(error in=w2954, "VI Ref"=w2955) -> (error out=w2953:errorcluster)  [unwired: 2 in, 3 out]
                }
                frame "Run top level" {
                  # "VI是活动层次结构中的顶层VI"
                  n2011 = property class="VI"(reference=w2966, error in=w2963, "FP.State"=T15."Closed" ("前面板窗口:状态")) -> (reference out=w2962:refnum<vi>, error out=w2964:errorcluster)
                  n2012 = call <vilib>:"Clear Errors.vi"("error in (no error)"=w2964) -> ("error out"=w2961:errorcluster)  [unwired: 5 in, 1 out]
                  n2013 = invoke on="子面板3" class="SubPnl" method="Insert VI"(error in=w2961, "VI Ref"=w2962) -> (error out=w2960:errorcluster)  [unwired: 2 in, 3 out]
                }
                frame "Running" {
                  # "VI已由一个或多个处于活动状态的顶层VI保留为执行"
                  n2014 = invoke on="子面板3" class="SubPnl" method="Insert VI"(error in=w2968, "VI Ref"=w2969) -> (error out=w2967:errorcluster)  [unwired: 2 in, 3 out]
                }
              }
            }
          }
        }
      }
      frame "压力退回" {
        n2015 = property on="数组 3" class="Arr (严格)"() -> ("Value"=w2970:refnum<vi>[])  [unwired: 2 in, 2 out]
        n2016 = for {
          tunnel: w2970 -> [w2972] mode=indexing
          n2017 = property class="VI"(reference=w2972) -> ("Name"=w2975:string)  [unwired: 1 in, 2 out]
          n2018 = Equal?(x=w2975, y="压力.vi") -> (x = y?=w2973:bool)
          n2019 = case shown="真" w2973 {
            tunnel: w2972 -> [_ w2976]
            frame False {
            }
            frame True {
              n2020 = property class="VI"(reference=w2976) -> (reference out=w2979:refnum<vi>, error out=w2977:errorcluster, "Exec.State"=w2978:T23)  [unwired: 1 in]
              n2021 = case shown="\"Running\"" w2978 {
                tunnel: w2979 -> [_ w2987 w2994 w2997]
                tunnel: w2977 -> [w2980 w2984 w2991 w2996]
                tunnel: [w2980 w2981 w2988 w2995] -> _
                frame "Bad", Default {
                  # "VI包含错误并且无法执行。"
                }
                frame "Idle" {
                  # "VI位于内存中但没有运行"
                  n2022 = invoke class="VI" method="Run VI"(reference=w2987, error in=w2984, "Wait until done"=FALSE ("结束前等待"), "Auto Dispose Ref"=FALSE ("自动销毁引用")) -> (reference out=w2983:refnum<vi>, error out=w2982:errorcluster)  [unwired: 1 in, 3 out]
                  n2023 = invoke on="子面板4" class="SubPnl" method="Insert VI"(error in=w2982, "VI Ref"=w2983) -> (error out=w2981:errorcluster)  [unwired: 2 in, 3 out]
                }
                frame "Run top level" {
                  # "VI是活动层次结构中的顶层VI"
                  n2024 = property class="VI"(reference=w2994, error in=w2991, "FP.State"=T15."Closed" ("前面板窗口:状态")) -> (reference out=w2990:refnum<vi>, error out=w2992:errorcluster)
                  n2025 = call <vilib>:"Clear Errors.vi"("error in (no error)"=w2992) -> ("error out"=w2989:errorcluster)  [unwired: 5 in, 1 out]
                  n2026 = invoke on="子面板4" class="SubPnl" method="Insert VI"(error in=w2989, "VI Ref"=w2990) -> (error out=w2988:errorcluster)  [unwired: 2 in, 3 out]
                }
                frame "Running" {
                  # "VI已由一个或多个处于活动状态的顶层VI保留为执行"
                  n2027 = invoke on="子面板4" class="SubPnl" method="Insert VI"(error in=w2996, "VI Ref"=w2997) -> (error out=w2995:errorcluster)  [unwired: 2 in, 3 out]
                }
              }
            }
          }
        }
      }
      frame "水质退回" {
        n2028 = property on="数组 3" class="Arr (严格)"() -> ("Value"=w2998:refnum<vi>[])  [unwired: 2 in, 2 out]
        n2029 = for {
          tunnel: w2998 -> [w3000] mode=indexing
          n2030 = property class="VI"(reference=w3000) -> ("Name"=w3003:string)  [unwired: 1 in, 2 out]
          n2031 = Equal?(x=w3003, y="水质.vi") -> (x = y?=w3001:bool)
          n2032 = case shown="真" w3001 {
            tunnel: w3000 -> [_ w3004]
            frame False {
            }
            frame True {
              n2033 = property class="VI"(reference=w3004) -> (reference out=w3005:refnum<vi>, error out=w3007:errorcluster, "Exec.State"=w3006:T23)  [unwired: 1 in]
              n2034 = case shown="\"Running\"" w3006 {
                tunnel: w3005 -> [_ w3015 w3022 w3025]
                tunnel: w3007 -> [w3008 w3012 w3019 w3024]
                tunnel: [w3008 w3009 w3016 w3023] -> _
                frame "Bad", Default {
                  # "VI包含错误并且无法执行。"
                }
                frame "Idle" {
                  # "VI位于内存中但没有运行"
                  n2035 = invoke class="VI" method="Run VI"(reference=w3015, error in=w3012, "Wait until done"=FALSE ("结束前等待"), "Auto Dispose Ref"=FALSE ("自动销毁引用")) -> (reference out=w3011:refnum<vi>, error out=w3010:errorcluster)  [unwired: 1 in, 3 out]
                  n2036 = invoke on="子面板5" class="SubPnl" method="Insert VI"(error in=w3010, "VI Ref"=w3011) -> (error out=w3009:errorcluster)  [unwired: 2 in, 3 out]
                }
                frame "Run top level" {
                  # "VI是活动层次结构中的顶层VI"
                  n2037 = property class="VI"(reference=w3022, error in=w3019, "FP.State"=T15."Closed" ("前面板窗口:状态")) -> (reference out=w3018:refnum<vi>, error out=w3020:errorcluster)
                  n2038 = call <vilib>:"Clear Errors.vi"("error in (no error)"=w3020) -> ("error out"=w3017:errorcluster)  [unwired: 5 in, 1 out]
                  n2039 = invoke on="子面板5" class="SubPnl" method="Insert VI"(error in=w3017, "VI Ref"=w3018) -> (error out=w3016:errorcluster)  [unwired: 2 in, 3 out]
                }
                frame "Running" {
                  # "VI已由一个或多个处于活动状态的顶层VI保留为执行"
                  n2040 = invoke on="子面板5" class="SubPnl" method="Insert VI"(error in=w3024, "VI Ref"=w3025) -> (error out=w3023:errorcluster)  [unwired: 2 in, 3 out]
                }
              }
            }
          }
        }
      }
    }
  }
  n2041 = Release Queue(queue=w5) -> ()  [unwired: 2 in, 3 out]
  "字符串 3" <- "测量" ("字符串 3")
  "用户：" <- "张三" ("用户：")
  "登录时间：" <- "2022-7-28:10:52:12" ("测试时间：")
  "报警信息" <- "水箱缺水" ("报警信息")
  "电流范围" <- "100A" ("电流范围")
  "电压范围" <- "10V" ("电压范围")
  "测试类型 2" <- "阶梯扫描" ("测试类型 2")
  "通讯方式" <- "LAN" ("通讯方式")
  "当前温度" <- "50" ("当前温度")
  "电源模式" <- "CC" ("电源模式")
  "水箱液位" <- "50.17 %"
  "水箱温度" <- "35.22 ℃"
  "氢中氧" <- "0.32%LEL"
  "氢渗" <- "0.42%LEL"
  "冷却水水压" <- "0.1MPa"
  "循环水压" <- "0.1MPa"
  "水质电导率" <- "0.1MΩ·cm"
  "电解电流" <- "320.0A"
  "电解电压" <- "73.9V"
  "气分液位" <- "22.61 %"
  "纯度仪" <- "99.999 %"
  "微量氧" <- "5.0PPM" ("微量氧")
  "露点仪" <- "-76.1 ℃" ("露点仪")
  "冷凝器液位" <- "1.07%" ("露点仪")
  "水箱液位 2" <- "50.17 %"
  "水箱温度 2" <- "35.22 ℃"
  "氢中氧 2" <- "0.32%LEL"
  "氢渗 2" <- "0.42%LEL"
  "冷却水水压 2" <- "0.1MPa"
  "循环水压 2" <- "0.1MPa"
  "水质电导率 2" <- "0.1MΩ·cm"
  "电解电流 2" <- "320.0A"
  "电解电压 2" <- "73.9V"
  "气分液位 2" <- "22.61 %"
  "纯度仪 2" <- "99.999 %"
  "微量氧 2" <- "5.0PPM" ("微量氧")
  "露点仪 2" <- "-76.1 ℃" ("露点仪")
  "冷凝器液位 2" <- "1.07%" ("露点仪")
